vi "Main.vi"() -> ()   [LabVIEW 2015]
uses:
  CustomControl/Model.ctl
  CustomControl/Main Cluster.ctl
  CustomControl/TestParameter.ctl
  CustomControl/MLFB Info.ctl
  CustomControl/Report Info.ctl
  CustomControl/ReportTitle.ctl
  CustomControl/addrPower.ctl
  <vilib>/addons/database/Connection.llb/Conn ObjectReference.ctl
  CustomControl/Lang_Control.ctl
  CustomControl/Autority.ctl
  CustomControl/Keithly Action.ctl
  CustomControl/JustCode.ctl
  CustomControl/Process.ctl
  CustomControl/UserRight.ctl
  <vilib>/addons/database/NI_Database_API.lvlib
panel:
  in  "DisableCurtain":bool caption="关闭安全光幕"
  out "EnablePLC":i32
  out "Register":i32[](array[numeric])
  out "Current":dbl
  out "PLC":refnum<visa-resource-name>
  in  "LCOneT":bool
  out "LightCurtain":bool
  out "No Current":bool
  out "Abort":bool
  in  "Voltage Reset":bool caption="Reset"
  out "voltage":dbl[](array[numeric])
  out "34461":refnum<visa-resource-name>
  in  "Keithly":T1=enum."Null"
  out "IOLightCurtain":bool
  out "Run?":bool=TRUE
  in  "Output":refnum<k21>="Output"
  in  "Input":refnum<k21>="Input"
  out "Operator":string caption="员工"
  in  "Lang":T2
  in  "MainCluster":T3={"parameter"={"Instr"={"34461"="GPIB0::16::INSTR", "PLC"="221", "pwr485"="COM3"}, "pwrSwitch"="Power", "voltage"=[], "mesCurrent"=0.0, "testCurrent"=0.0, "baseCurrent"=0.0, "KG20"=[1.0500000000000007, 1.2, 1.3, 1.4], "KG"=0.0, "KTu"=[], "temperature"=[], "MLFB Info"={"MLFB"="", "Frame"="", "curRange"="", "thermoRs"=0.0, "releaseRs"=0.0, "circuitRs"=0.0, "IL_Current"=0.0, "IL_KG"=0.0, "IL_consTIme"=0, "uL_Current"=0.0, "uL_KG"=0.0, "uL_consTIme"=0, "DA"=0.0, "Action_P1"=0, "Action_P2"=0, "Limit_P1"=0, "Limit_P2"=0, "Limit_P3"=0, "Limit_P4"=0, "reTemperature"=0, "iGauge"=0.0, "oGauge"=0.0, "Torque"=""}, "path"={"template (empty)"=path "", "Report path"=path "", "Backup path"=path ""}, "Report"={"Title"={"订单数量"="", "订单号"="", "生产代码"="", "日期"="", "开始时间"="", "结束时间"="", "测试数量"="", "预载荷时间"=0, "载荷时间"=0, "检验员"="", "MLFB"="", "电流范围"="", "起动时间"="", "快速时间范围"=""}, "uL"={"KTU"=[], "Testing temp"=[], "consTime"=0, "KG"=0.0, "Tripped Time"=[], "test?"=FALSE, "KGR"=[]}, "IL"={"KTU"=[], "Testing temp"=[], "consTime"=0, "KG"=0.0, "Tripped Time"=[], "test?"=FALSE, "KGR"=[]}, "Voltage"=[], "preLoad"=0, "Load"=0, "Total"=0, "JustCode"=[]}, "IO"={"Break"="Tripped", "Out"="Output", "Input"="Input", "Contactor"="Tripped"}, "recordVoltageTime"=60, "buffer"={"temp"=0.0, "PowerSwitch"=[]}, "UL?"=FALSE, "numTrip"=[0, 0, 0, 0], "unIndex"=[], "Message"="", "addrPower"=enum."5A power", "errPower"=FALSE, "Tripped Time"=[], "KGR"=[], "consTime"=0, "Authority"=0, "MLFB"=refnum, "uninstallNum"=0, "trip"=[]}, "File Path"={"reportPath"=path "", "limitTemplate"=path "", "actionTemplate"=path "", "initialPath"=path "", "backupPath"=path ""}, "Period"=0, "Elapse"=0, "Start"=FALSE, "Clear"=FALSE, "Test Count"=0, "TrippedCount"=0, "DelayByUser"=0.0, "DelayInCase"=0.0, "CheckVoltage"=FALSE, "UpLimitVol"=0.0, "DownLimitVol"=0.0}
  in  "exit":bool
  in  "Set":bool
  in  "Edit":bool
  in  "New":bool
  in  "btnAbort":bool
  in  "Start":bool
  in  "Logout":bool caption="3RV极限电流测试系统"
  out "action2CurFactor":dbl caption="动作特性2"
  out "Tab":T10(tab)
  in  "Login":bool caption="登录"
  in  "Password":string caption="密码:"
  in  "UserID":string caption="员工号:"
  out "ShowTripTime":T11
  out "Total":string
  out "remaing":string caption="P1"
  out "EndTime":string caption="测试结束"
  out "StartTime":string caption="测试开始"
  out "totalHour":string
  out "totalSec":string caption="最长测试时间"
  out "trippedStatus":T12={"1"=TRUE, "2"=TRUE, "3"=TRUE, "4"=TRUE, "5"=TRUE, "6"=TRUE, "7"=TRUE, "8"=TRUE, "9"=TRUE, "10"=TRUE, "11"=TRUE, "12"=TRUE, "13"=TRUE, "14"=TRUE, "15"=TRUE, "16"=TRUE, "17"=TRUE, "18"=TRUE, "19"=TRUE, "20"=TRUE}
  in  "Report":bool caption="Generator Report"
  out "orderNum_M":string caption="订单号"
  out "MLFB_show":string caption="MLFB"
  out "process":string caption="测试类型"
  out "current":dbl caption="当前测试电流" format="%#.2g"
  in  "parameter":i32[](listbox)
  out "RunInfo":string caption="运行信息"
  out "Pass":bool caption="通过"
  out "Fail":bool caption="失败"
  out "pirntProcess":u8(slide) scale=0.0..10.0
  in  "ThermalTmFrame":string caption="快速时间范围"
  in  "AccelerationTime":string caption="起动时间"
  out "action2preload":i32 caption="动作特性2"
  out "Factor_Action2":string="7.2"
  out "action2":i32 caption="动作特性2"
  in  "orderNum_P":string caption="订单号"
  out "testCount":string caption="测试数量"
  in  "productCode":string caption="生产代码"
  in  "orderCount":string caption="订单数量"
  in  "TestModel":T13
  in  "Cancel_Para":bool caption="Test"
  in  "ok_Para":bool
  out "load_Limit":i32 caption="载荷"
  out "preload_Limit":i32 caption="预载荷"
  out "Test Date":string caption="测试日期"
  out "Frame":string caption="框架"
  out "Reference temp":i32=20 caption="基准温度"
  out "load_Action":i32 caption="动作特性 1"
  out "preload_Action":i32 caption="极限电流"
  out "Gauge_Out":dbl caption="出现线径"
  out "Gauge_In":dbl caption="进线线径"
  out "Factor_Limit":string="1.05->1.2->1.3->1.4" caption="电流系数"
  out "Factor_Action":string="1.05->1.2" caption="动作特性 2"
  out "Torque":string caption="扭矩"
  out "DA_uL":dbl
  out "DA_IL":dbl caption="期望值"
  out "KG20_uL":dbl
  out "KG20_IL":dbl caption="温度系数"
  out "consTime_uL":i32
  out "consTime_IL":i32 caption="时间常数"
  out "Current_uL":dbl
  out "Current_IL":dbl caption="测试电流"
  out "Operator_test":string caption="操作员"
  in  "MLFB":string
  out "Temperature":string caption="温度"
  in  "Just Code":T14
  in  "Cancel Add":bool
  in  "Add MLFB":bool caption="Add"
  in  "curRange N":string caption="电流范围"
  out "Factor_Limit N":string="1.05->1.2->1.3->1.4" caption="电流系数"
  in  "Preload_Limit N":i32 caption="预载荷"
  in  "Load_Limit N":i32 caption="载荷"
  in  "Resistance N":dbl caption="内阻"
  out "Factor_Action N":string="1.05->1.2"
  in  "Frame N":string caption="框架"
  in  "Current_IL N":dbl caption="电流范围"
  in  "Current_uL N":dbl
  in  "consTime_IL N":i32 caption="时间常数"
  in  "consTime_uL N":i32
  in  "KG20_IL N":dbl caption="温度系数"
  in  "KG20_uL N":dbl
  in  "DA N":dbl caption="期望值"
  in  "Torque N":string caption="扭矩"
  in  "Gauge_In N":dbl caption="进线线径"
  in  "Gauge_Out N":dbl caption="出线线径"
  in  "Preload_Release N":i32 caption="极限电流"
  in  "Load_Release N":i32 caption="动作特性"
  in  "reTemperature N":i32=20 caption="基准温度"
  in  "thermoRs":dbl caption="热元件电阻值"
  in  "releaseRs":dbl caption="电流脱扣器电阻值"
  in  "MLFB N":string caption="MLFB"
  in  "btnDelete":bool caption="删除"
  in  "Cancel_Edit":bool caption="Cancel"
  in  "Ok_Edit":bool caption="Edit"
  in  "Load_Limit E":i32 caption="载荷"
  in  "Preload_Limit E":i32 caption="预载荷"
  out "FactorLimit E":string="1.05->1.2->1.3->1.4" caption="电流系数"
  in  "reTemperature E":i32=20 caption="基准温度"
  in  "Load_Action E":i32 caption="动作特性"
  in  "Preload_Action E":i32 caption="极限电流"
  in  "Gauge_Out E":dbl caption="出线线径"
  in  "Gauge_In E":dbl caption="进线线径"
  in  "Torque E":string caption="扭矩"
  in  "DA E":dbl caption="期望值"
  in  "KG_uL E":dbl
  in  "KG_IL E":dbl caption="温度系数"
  in  "consTime_uL E":i32
  in  "consTime_IL E":i32 caption="时间常数"
  in  "Current_uL E":dbl
  in  "Current_IL E":dbl caption="电流范围"
  in  "MLFB E":string caption="MLFB"
  in  "Frame E":string caption="框架"
  out "FactorRelease E":string="1.05->1.2"
  in  "circuitRs E":dbl caption="内阻"
  in  "curRange E":string caption="电流范围"
  in  "releaseRs E":dbl caption="电流脱扣器电阻值"
  in  "thermoRs E":dbl caption="热元件电阻值"
  in  "btnEditLCConfig":bool caption="New"
  in  "btnReadLCConfig":bool caption="安全光幕"
  out "vlCalTpr":dbl caption="实测温度"
  in  "btnCalTpr":bool caption="温度校验"
  in  "btnReadUser":bool caption="New"
  in  "readCalibra":bool caption="Read"
  out "valueCalibra":dbl caption="测试值"
  in  "Authority":T15 caption="权限"
  in  "btnDeleteUser":bool
  in  "btnEditUser":bool
  in  "btnNewUser":bool caption="用户权限"
  in  "txtPassword":string caption="密码"
  in  "txtName":string caption="姓名"
  in  "txtID":string caption="用户ID"
  in  "setCalibra":dbl caption="设定值"
  in  "btnCalibration":bool caption="电流校验"
  in  "abortCalibra":bool caption="Abort"
  in  "btnReturn":bool caption="Return"
  in  "DelayByUser":string caption="自恢复时间"
  in  "DelayToFailed":string caption="误触发极限"
  # "3RV Limit Current"
  # "sec."
  # "sec."
  # "sec."
  # "A"
  # "h/min/sec"
  # "Test"
  # "Sec"
  # "Sec"
  # "I.L"
  # "u.L"
  # "A"
  # "N.m"
  # "mm2"
  # "mm2"
  # "℃"
  # "℃"
  # "Add"
  # "mΩ"
  # "sec"
  # "sec"
  # "mΩ"
  # "mΩ"
  # "A"
  # "I.L"
  # "u.L"
  # "mm2"
  # "A"
  # "℃"
  # "mm2"
  # "N.m"
  # "Edit"
  # "mΩ"
  # "sec"
  # "sec"
  # "mΩ"
  # "mΩ"
  # "I.L"
  # "u.L"
  # "A"
  # "mm2"
  # "A"
  # "℃"
  # "mm2"
  # "N.m"
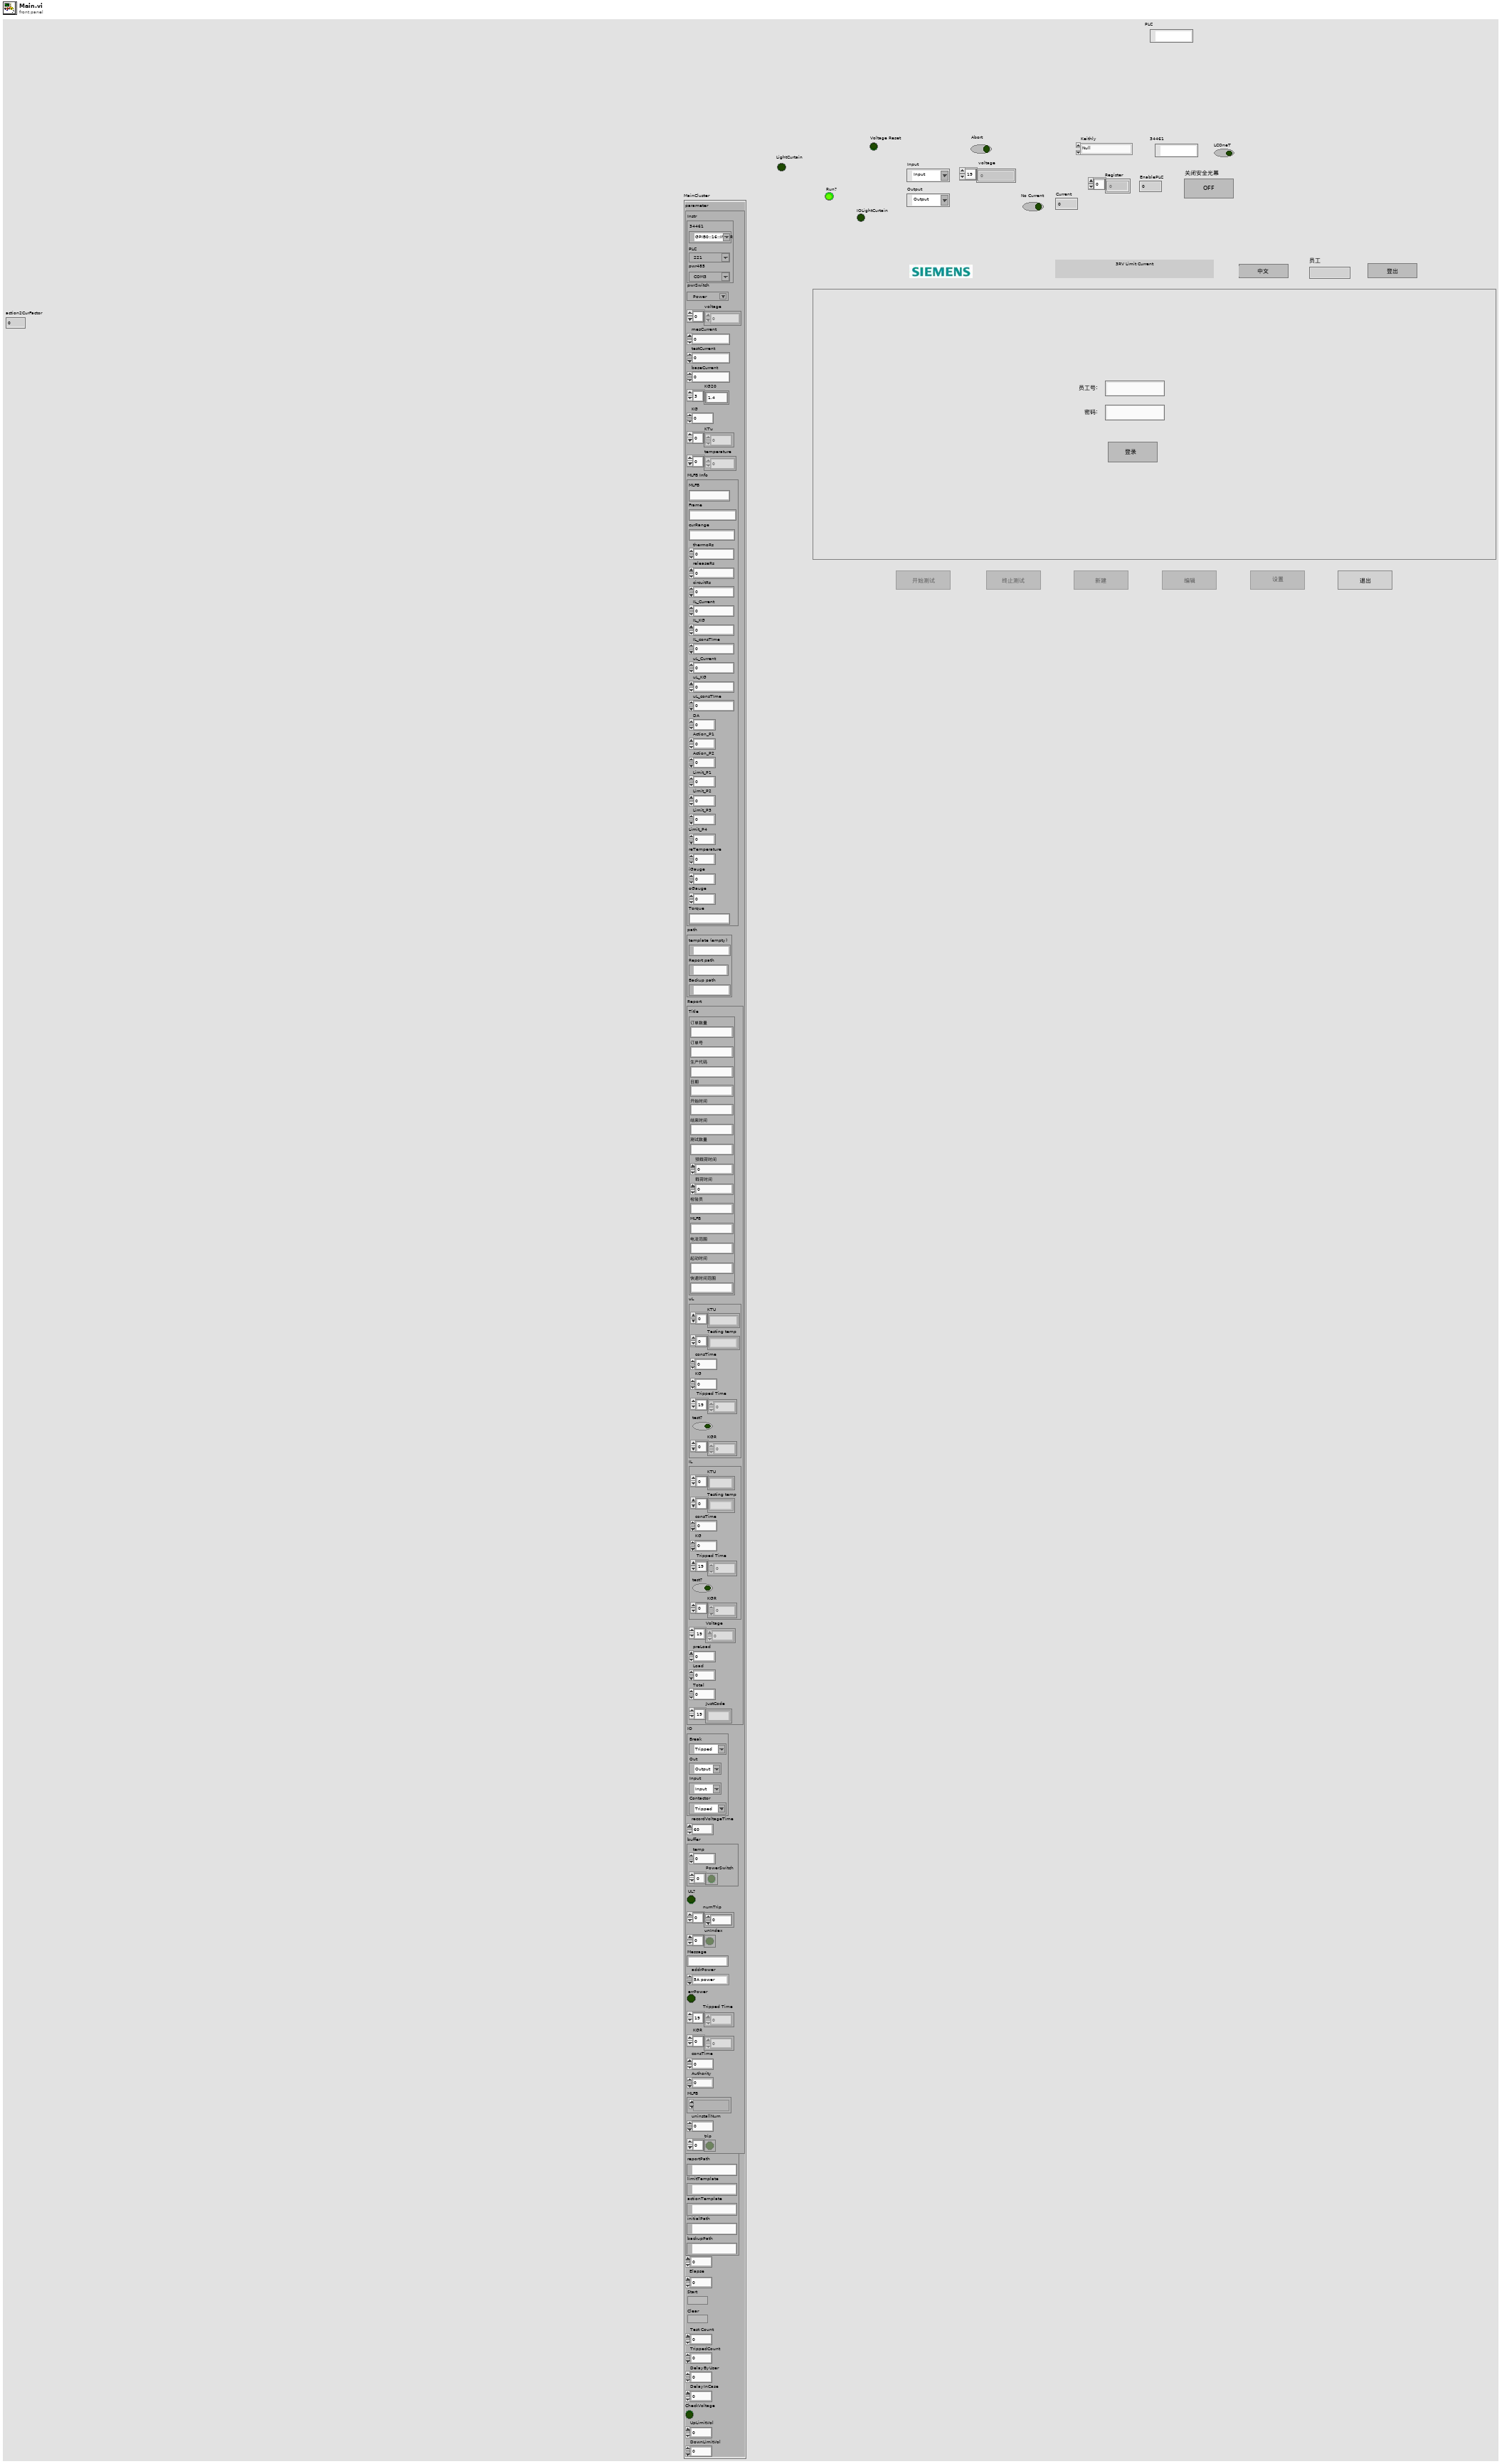
[diagram p1: front panel]
types:
  T1 = typedef "Keithly Action.ctl" = enum16{"Get Voltage", "Null"}
  T2 = typedef "Lang_Control.ctl" = enum16{"中文", "English"}
  T3 = typedef "Main Cluster.ctl" = cluster{"parameter":T4, "File Path":cluster{"reportPath":path, "limitTemplate":path, "actionTemplate":path, "initialPath":path, "backupPath":path}, "Period":u8, "Elapse":i32, "Start":bool, "Clear":bool, "Test Count":u8, "TrippedCount":i32, "DelayByUser":dbl, "DelayInCase":dbl, "CheckVoltage":bool, "UpLimitVol":dbl, "DownLimitVol":dbl}
  T4 = typedef "TestParameter.ctl" = cluster{"Instr":cluster{"34461":refnum<visa-resource-name>, "PLC":refnum<visa-resource-name>, "pwr485":refnum<visa-resource-name>}, "pwrSwitch":refnum<k21>, "voltage":dbl[], "mesCurrent":dbl, "testCurrent":dbl, "baseCurrent":dbl, "KG20":dbl[], "KG":dbl, "KTu":dbl[], "temperature":dbl[], "MLFB Info":T5, "path":cluster{"template (empty)":path, "Report path":path, "Backup path":path}, "Report":T6, "IO":cluster{"Break":refnum<k21>, "Out":refnum<k21>, "Input":refnum<k21>, "Contactor":refnum<k21>}, "recordVoltageTime":i32, "buffer":cluster{"temp":dbl, "PowerSwitch":bool[]}, "UL?":bool, "numTrip":i32[], "unIndex":bool[], "Message":string, "addrPower":T8, "errPower":bool, "Tripped Time":i32[], "KGR":dbl[], "consTime":i32, "Authority":u32, "MLFB":T9, "uninstallNum":i32, "trip":bool[]}
  T5 = typedef "MLFB Info.ctl" = cluster{"MLFB":string, "Frame":string, "curRange":string, "thermoRs":dbl, "releaseRs":dbl, "circuitRs":dbl, "IL_Current":dbl, "IL_KG":dbl, "IL_consTIme":i32, "uL_Current":dbl, "uL_KG":dbl, "uL_consTIme":i32, "DA":dbl, "Action_P1":i32, "Action_P2":i32, "Limit_P1":i32, "Limit_P2":i32, "Limit_P3":i32, "Limit_P4":i32, "reTemperature":i32, "iGauge":dbl, "oGauge":dbl, "Torque":string}
  T6 = typedef "Report Info.ctl" = cluster{"Title":T7, "uL":cluster{"KTU":string[], "Testing temp":string[], "consTime":i32, "KG":dbl, "Tripped Time":i32[], "test?":bool, "KGR":dbl[]}, "IL":cluster{"KTU":string[], "Testing temp":string[], "consTime":i32, "KG":dbl, "Tripped Time":i32[], "test?":bool, "KGR":dbl[]}, "Voltage":dbl[], "preLoad":i32, "Load":i32, "Total":i32, "JustCode":string[]}
  T7 = typedef "ReportTitle.ctl" = cluster{"订单数量":string, "订单号":string, "生产代码":string, "日期":string, "开始时间":string, "结束时间":string, "测试数量":string, "预载荷时间":i32, "载荷时间":i32, "检验员":string, "MLFB":string, "电流范围":string, "起动时间":string, "快速时间范围":string}
  T8 = typedef "addrPower.ctl" = enum16{"5A power", "300A power"}
  T9 = typedef "NI_Database_API.lvlib/Conn ObjectReference.ctl" = refnum<k1>
  T10 = enum32{"Login", "Test", "Parameter", "Add MLFB", "Edit MLFB", "Calibration Power"}
  T11 = cluster{"1":i32, "2":i32, "3":i32, "4":i32, "5":i32, "6":i32, "7":i32, "8":i32, "9":i32, "10":i32, "11":i32, "12":i32, "13":i32, "14":i32, "15":i32, "16":i32, "17":i32, "18":i32, "19":i32, "20":i32}
  T12 = cluster{"1":bool, "2":bool, "3":bool, "4":bool, "5":bool, "6":bool, "7":bool, "8":bool, "9":bool, "10":bool, "11":bool, "12":bool, "13":bool, "14":bool, "15":bool, "16":bool, "17":bool, "18":bool, "19":bool, "20":bool}
  T13 = typedef "Model.ctl" = enum32{"lowLimit", "upLimit", "lowAction1", "upAction1", "lowAction2", "upAction2"}
  T14 = typedef "JustCode.ctl" = cluster{"1":string, "2":string, "3":string, "4":string, "5":string, "6":string, "7":string, "8":string, "9":string, "10":string, "11":string, "12":string, "13":string, "14":string, "15":string, "16":string, "17":string, "18":string, "19":string, "20":string}
  T15 = typedef "Autority.ctl" = enum16{"Operator", "Engineer"}
  T16 = typedef "Process.ctl" = enum16{"Initial_Data", "Initial_HMI", "Language", "UI", "Login", "Authority", "Clear", "Initial Test Data", "Initial Test Data1", "Initial Test UI", "Test Parameter", "PowerRemote", "PowerON", "PowerCalibration", "PowerOFF", "Temperature", "TempOffset", "Trip", "ShowInfo", "Finish?", "Period?", "LoopCurrent", "Procedure", "KGR", "Passed", "Failed", "MLFB Decoding", "MLFB Test Info", "MLFB Edit Info", "MLFB Edit", "MLFB Insert", "MLFB Delete", "ReportGeneralInfo", "ReportResultInfo", "ReportPath", "Generate Report", "Print Report", "New User", "Edit User", "Delete User", "Read User", "Voltage", "Time", "Current Calibration", "ErrorHandle", "StartTest", "ActiveLightCur", "Uninstall Record", "Get Uninstall Count", "Abort Test", "Test Model?", "CheckLoopCurrent", "Release HW Source", "Exit", "Close DB Connection", "Test UI BTN Status", "unTest UI BTN Status", "Disable All BTN", "AbortCalibration", "TprCalibration", "ClearReportInfo", "Set Uninstall", "TestResult", "SetLightCur", "CheckVoltage", "ShowTripTime"}
  T17 = enum16{"HighVoltage", "LowVoltage", "Temperature", "AllOFF"}
  T18 = enum8{"Enabled", "Disabled", "Disabled and Grayed Out"}
  T19 = enum16{"HighVoltage", "LowVoltage", "Temperature"}
  T20 = typedef "UserRight.ctl" = cluster{"ID_Number":string, "Name":string, "Password":string, "Authority":i32}
  T21 = enum32{"invalid app kind", "Development System", "Run Time System", "Student Edition", "Embedded LabVIEW", "Evaluation", "Custom"}
  T22 = cluster{"[0]":bool, "[1]":bool, "[2]":bool, "[3]":bool, "[4]":bool, "[5]":bool, "[6]":bool, "[7]":bool, "[8]":bool, "[9]":bool, "[10]":bool, "[11]":bool, "[12]":bool, "[13]":bool, "[14]":bool, "[15]":bool, "[16]":bool, "[17]":bool, "[18]":bool, "[19]":bool}
  T23 = cluster{"[0]":i32, "[1]":i32, "[2]":i32, "[3]":i32, "[4]":i32, "[5]":i32, "[6]":i32, "[7]":i32, "[8]":i32, "[9]":i32, "[10]":i32, "[11]":i32, "[12]":i32, "[13]":i32, "[14]":i32, "[15]":i32, "[16]":i32, "[17]":i32, "[18]":i32, "[19]":i32}
  T24 = cluster{"trip[0]":bool, "trip[1]":bool, "trip[2]":bool, "trip[3]":bool, "trip[4]":bool, "trip[5]":bool, "trip[6]":bool, "trip[7]":bool, "trip[8]":bool, "trip[9]":bool, "trip[10]":bool, "trip[11]":bool, "trip[12]":bool, "trip[13]":bool, "trip[14]":bool, "trip[15]":bool, "trip[16]":bool, "trip[17]":bool, "trip[18]":bool, "trip[19]":bool}
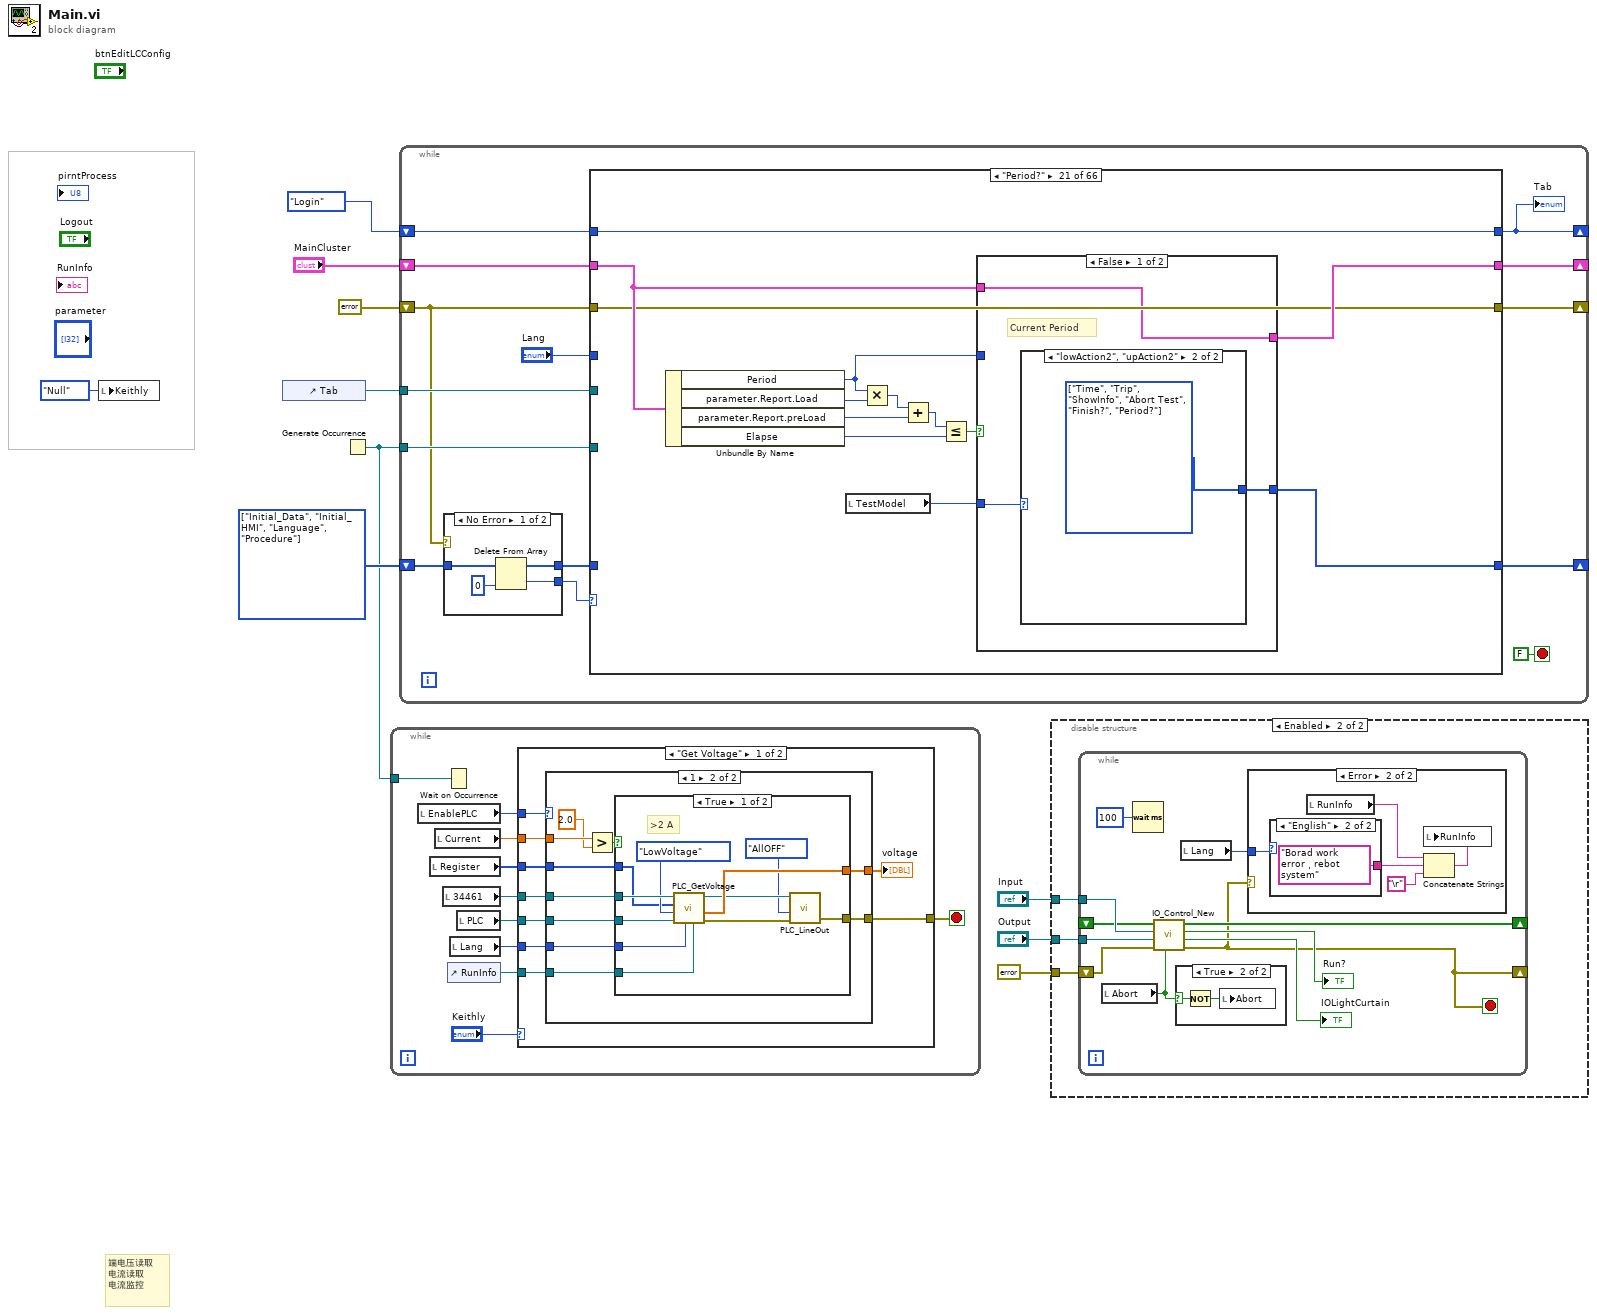
[diagram p0: block diagram]
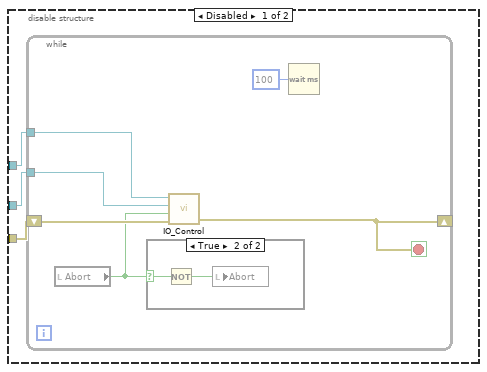
[diagram p2: hidden frame]
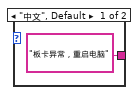
[diagram p5: hidden frame]
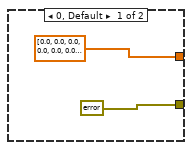
[diagram p7: hidden frame]
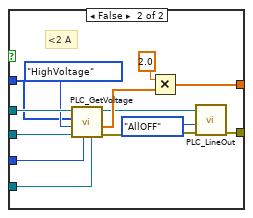
[diagram p8: hidden frame]
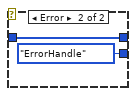
[diagram p10: hidden frame]
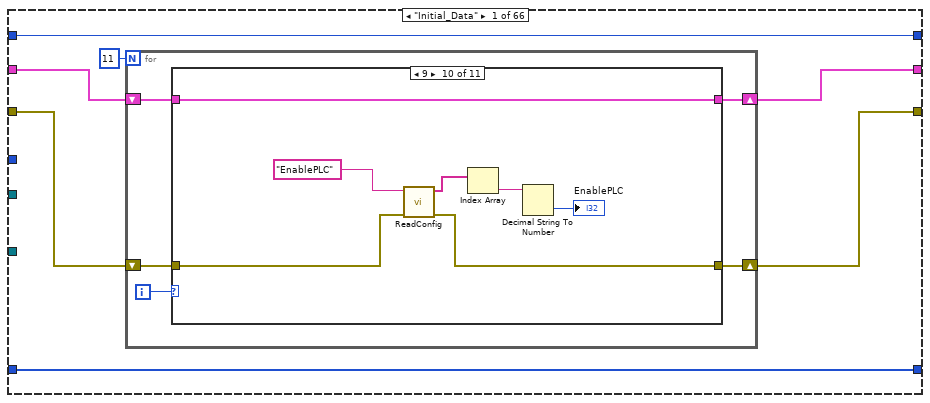
[diagram p11: hidden frame]
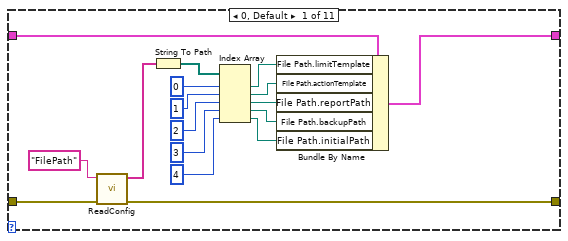
[diagram p12: hidden frame]
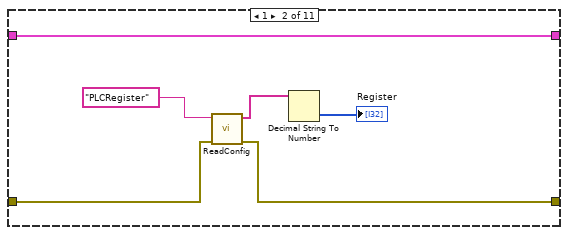
[diagram p13: hidden frame]
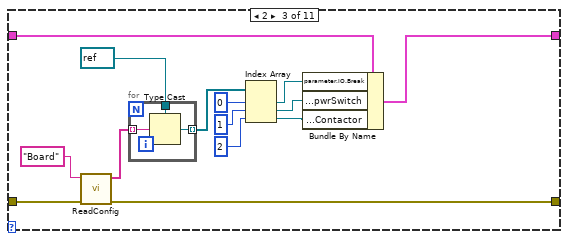
[diagram p14: hidden frame]
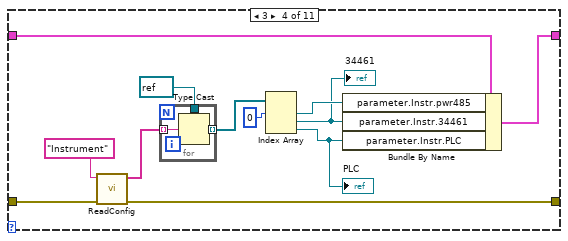
[diagram p15: hidden frame]
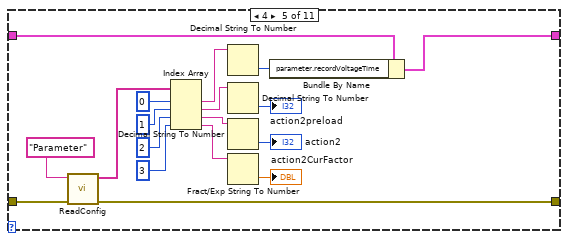
[diagram p16: hidden frame]
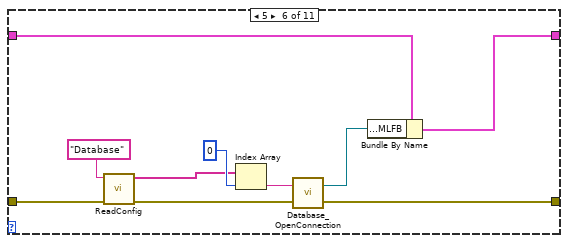
[diagram p17: hidden frame]
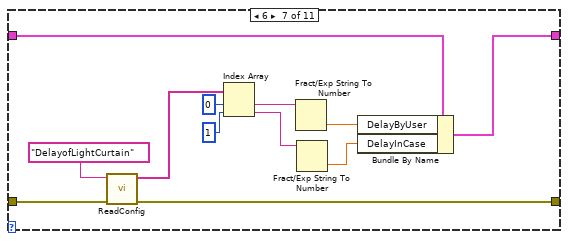
[diagram p18: hidden frame]
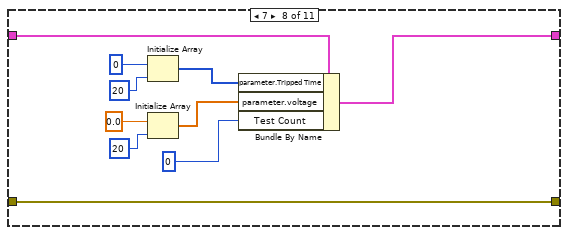
[diagram p19: hidden frame]
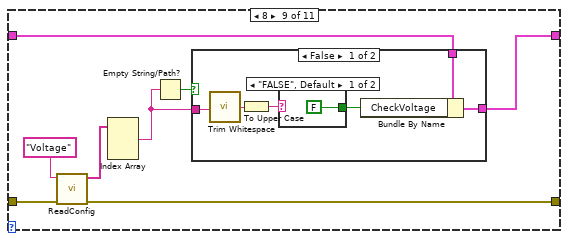
[diagram p20: hidden frame]
diagram:
  w7 = T16[] [enum."Initial_Data", enum."Initial_HMI", enum."Language", enum."Procedure"] items=["Initial_Data", "Initial_HMI", "Language", "UI", "Login", "Authority", "Clear", "Initial Test Data", "Initial Test Data1", "Initial Test UI", "Test Parameter", "PowerRemote", "PowerON", "PowerCalibration", "PowerOFF", "Temperature", "TempOffset", "Trip", "ShowInfo", "Finish?", "Period?", "LoopCurrent", "Procedure", "KGR", "Passed", "Failed", "MLFB Decoding", "MLFB Test Info", "MLFB Edit Info", "MLFB Edit", "MLFB Insert", "MLFB Delete", "ReportGeneralInfo", "ReportResultInfo", "ReportPath", "Generate Report", "Print Report", "New User", "Edit User", "Delete User", "Read User", "Voltage", "Time", "Current Calibration", "ErrorHandle", "StartTest", "ActiveLightCur", "Uninstall Record", "Get Uninstall Count", "Abort Test", "Test Model?", "CheckLoopCurrent", "Release HW Source", "Exit", "Close DB Connection", "Test UI BTN Status", "unTest UI BTN Status", "Disable All BTN", "AbortCalibration", "TprCalibration", "ClearReportInfo", "Set Uninstall", "TestResult", "SetLightCur", "CheckVoltage", "ShowTripTime"]
  # "端电压读取\n电流读取\n电流监控"
  n1 = local write "Keithly"(Keithly_Action."Null" ("Keithly")) -> ()
  n2 = control-ref of="Tab"() -> (w9:refnum<vi>)
  n3 = Generate Occurrence() -> (w5:refnum<k4>)
  n4 = while {
    tunnel: w5 -> [w20]
    stop <- w19 stop-if-true
    n5 = local read "EnablePLC"() -> (w14:i32)
    n6 = local read "Register"() -> (w13:i32[])
    n7 = local read "Current"() -> (w15:dbl)
    n8 = local read "34461"() -> (w18:refnum<visa-resource-name>)
    n9 = Wait on Occurrence(2:w20) -> ()  [unwired: 2 in, 1 out]
    n10 = control-ref of="RunInfo"() -> (w12:refnum<vi>)
    n11 = local read "Lang"() -> (w11:T2)
    n12 = local read "PLC"() -> (w16:refnum<visa-resource-name>)
    n13 = case shown="\"Get Voltage\"" "Keithly" {
      tunnel: [w28 _] -> w19
      tunnel: w18 -> [w29 _]
      tunnel: w16 -> [w26 _]
      tunnel: w15 -> [w25 _]
      tunnel: w14 -> [w24 _]
      tunnel: w13 -> [w23 _]
      tunnel: w12 -> [w22 _]
      tunnel: w11 -> [w21 _]
      frame "Get Voltage" {
        n14 = case shown="1" w24 {
          tunnel: w29 -> [_ w41]
          tunnel: [errorcluster {"status"=FALSE, "code"=0, "source"=""} ("error out") w35] -> w28
          tunnel: [dbl[] [0.0, 0.0, 0.0, 0.0, 0.0, 0.0, 0.0, 0.0, 0.0, 0.0, 0.0, 0.0, 0.0, 0.0, 0.0, 0.0, 0.0, 0.0, 0.0, 0.0] ("Array") w40] -> w27
          tunnel: w26 -> [_ w39]
          tunnel: w25 -> [_ w38]
          tunnel: w23 -> [_ w34]
          tunnel: w22 -> [_ w33]
          tunnel: w21 -> [_ w32]
          frame 0, Default {
          }
          frame 1 {
            n15 = Greater?(x=w38, y=2.0) -> (0:w37:bool)
            n16 = case shown="True" w37 {
              tunnel: w41 -> [w52 w65]
              tunnel: [w47 w59] -> w35
              tunnel: [w48 w62] -> w40
              tunnel: w39 -> [w50 w63]
              tunnel: w34 -> [w44 w55]
              tunnel: w33 -> [w42 w54]
              tunnel: w32 -> [w43 w53]
              frame True {
                # ">2 A"
                n17 = call "PLC_GetVoltage.vi"("Msg"=w42, "Language"=w43, "PLC"=w50, "Selection"=T17."LowVoltage", "VoltageIO"=w44, "VISA"=w52) -> ("error out"=w51:errorcluster, "Array"=w48:dbl[], "VISA resource name out"=w46:refnum<visa-resource-name>)  [unwired: 3 in]
                n18 = call "PLC_LineOut.vi"("error in (no error)"=w51, "Selection"=T17."AllOFF", "VISA resource name"=w46) -> ("error out"=w47:errorcluster)  [unwired: 2 in, 1 out]
              }
              frame False {
                # "<2 A"
                n19 = call "PLC_GetVoltage.vi"("Msg"=w54, "Language"=w53, "PLC"=w63, "Selection"=T17."HighVoltage", "VoltageIO"=w55, "VISA"=w65) -> ("error out"=w64:errorcluster, "Array"=w58:dbl[], "VISA resource name out"=w57:refnum<visa-resource-name>)  [unwired: 3 in]
                n20 = Multiply(x=2.0, y=w58) -> (x*y=w62:dbl[])
                n21 = call "PLC_LineOut.vi"("error in (no error)"=w64, "Selection"=T17."AllOFF", "VISA resource name"=w57) -> ("error out"=w59:errorcluster)  [unwired: 2 in, 1 out]
              }
            }
          }
        }
        "voltage" <- w27
      }
      frame "Null" {
      }
    }
  }
  n22 = while {
    shift-right: [w76] -> _
    shift-left: "MainCluster" -> [w78]
    shift-right: [w70] -> _
    shift-left: T10."Login" ("Tab") -> [w79]
    shift-right: [w77] -> _
    shift-left: errorcluster {"status"=FALSE, "code"=0, "source"=""} ("error out") -> [w67]
    tunnel: w9 -> [w75]
    shift-right: [w72] -> _
    shift-left: w7 -> [w74]
    tunnel: w5 -> [w68]
    stop <- FALSE stop-if-true
    n23 = case shown="No Error" w67 {
      tunnel: w74 -> [w83 w85]
      tunnel: [w80 w85] -> w73
      tunnel: [w81 Process."ErrorHandle" ("Process")] -> w66
      frame No Error {
        n24 = Delete From Array(array=w83, index=0) -> (deleted portion=w81:T16, array with subset deleted=w80:T16[])  [unwired: 1 in]
      }
      frame Error {
      }
    }
    n25 = case shown="\"Period?\"" w66 {
      tunnel: w79 -> [w92 w237 w279 w557 w745 w794 w803 w851 w856 w877 w891 w1030 w1044 w1057 w1069 w1079 w1096 w1126 w1133 w1166 w1192 w1217 w1221 w1233 w1239 w1262 w1290 w1312 w1340 w1373 w1416 w1456 w1479 w1493 w1525 w1535 w1564 w1578 w1608 w1625 w1655 w1666 w1683 w1687 w1693 w1709 w1730 w1743 w1770 w1779 w1799 w1828 w1837 w1844 w1855 w1861 w1867 w1872 w1879 w1891 w1897 w1905 w1912 w1951 w1983 w2015]
      tunnel: w78 -> [w91 w235 w280 w556 w749 w792 w802 w848 w853 w874 w888 w1026 w1039 w1054 w1064 w1076 w1105 w1117 w1131 w1153 w1182 w1213 w1220 w1224 w1236 w1259 w1288 w1309 w1337 w1372 w1415 w1452 w1475 w1480 w1509 w1533 w1563 w1577 w1607 w1623 w1654 w1660 w1678 w1688 w1695 w1713 w1729 w1736 w1767 w1778 w1794 w1827 w1836 w1845 w1851 w1860 w1866 w1871 w1878 w1888 w1893 w1902 w1910 w1948 w1980 w2012]
      tunnel: w67 -> [w90 w236 w281 w555 w753 w793 w801 w849 w855 w876 w889 w1029 w1045 w1055 w1068 w1072 w1099 w1129 w1132 w1152 w1181 w1215 w1218 w1231 w1238 w1261 w1286 w1310 w1338 w1363 w1414 w1455 w1478 w1494 w1524 w1534 w1561 w1565 w1603 w1624 w1642 w1665 w1682 w1686 w1702 w1712 w1728 w1742 w1768 w1777 w1798 w1826 w1835 w1846 w1853 w1859 w1865 w1870 w1876 w1884 w1895 w1904 w1911 w1945 w1978 w2014]
      tunnel: [w89 w236 w281 w554 w743 w793 w801 w849 w855 w876 w889 w1027 w1041 w1047 w1065 w1073 w1099 w1109 w1132 w1152 w1181 w1214 w1218 w1230 w1238 w1261 w1277 w1310 w1338 w1371 w1413 w1454 w1478 w1494 w1513 w1532 w1557 w1575 w1596 w1613 w1640 w1665 w1681 w1686 errorcluster {"status"=FALSE, "code"=0, "source"=""} ("error IO") w1712 w1727 w1742 w1757 w1777 w1798 w1826 w1834 w1846 w1852 w1859 w1865 w1870 w1873 w1889 w1895 w1903 w1911 w1945 w1977 w2014] -> w77
      tunnel: [w88 w235 w280 w553 w744 w792 w802 w836 w852 w874 w890 w1026 w1038 w1054 w1064 w1075 w1104 w1120 w1131 w1153 w1186 w1213 w1220 w1223 w1235 w1259 w1287 w1309 w1337 w1372 w1415 w1452 w1476 w1481 w1519 w1531 w1563 w1577 w1607 w1623 w1654 w1660 w1679 w1688 w1695 w1713 w1729 w1735 w1766 w1778 w1793 w1827 w1836 w1845 w1851 w1860 w1866 w1871 w1878 w1888 w1892 w1902 w1909 w1948 w1980 w2012] -> w76
      tunnel: w75 -> [_ _ _ _ _ _ _ _ _ _ _ _ _ _ _ _ _ _ _ _ _ _ _ _ _ _ _ _ _ _ _ _ _ _ _ _ _ _ _ _ _ _ _ _ _ _ _ _ _ _ _ _ _ _ _ _ _ _ _ _ _ _ _ _ _ _]
      tunnel: [w92 w237 w279 w550 w750 w794 w803 w851 w856 w877 w891 w1030 w1044 w1057 w1069 w1079 w1096 w1126 w1133 w1166 w1192 w1217 w1221 w1233 w1239 w1262 w1290 w1312 w1340 w1373 w1416 w1456 w1479 w1493 w1525 w1535 w1564 w1578 w1608 w1625 w1655 w1666 w1683 w1687 w1690 w1708 w1730 w1743 w1770 w1779 w1799 w1828 w1837 w1844 w1855 w1861 w1867 w1872 w1879 w1891 w1897 w1905 w1912 w1951 w1983 w2015] -> w70
      tunnel: [w86 w234 w278 w549 w741 w790 w799 w850 w854 w875 w885 w1025 w1040 w1056 w1063 w1078 w1095 w1121 w1130 w1158 w1187 w1216 w1219 w1232 w1237 w1260 w1289 w1311 w1339 w1367 w1407 w1457 w1477 w1492 w1518 w1536 w1560 w1574 w1597 w1622 w1645 w1664 w1684 w1685 w1700 w1707 w1731 w1741 w1764 w1776 w1797 w1824 w1838 w1847 w1854 w1858 w1864 w1869 w1877 w1890 w1896 w1899 w1907 w1950 w1982 w2013] -> w72
      tunnel: w73 -> [w86 w234 w278 _ w742 w790 w800 w850 w854 w875 w885 w1025 w1040 w1056 w1063 w1078 w1095 w1121 w1130 w1160 _ w1216 _ w1232 w1237 w1260 w1289 w1311 w1339 w1367 w1407 w1457 w1477 w1492 w1518 w1536 w1560 w1574 w1597 w1622 w1645 w1664 w1684 w1685 _ _ w1731 w1741 w1764 w1776 w1797 w1825 w1838 w1847 w1854 w1858 w1864 w1869 w1877 w1890 w1896 w1899 _ w1950 w1982 w2013]
      tunnel: "Lang" -> [_ w233 w277 w551 w751 _ _ _ _ _ w886 w1022 w1031 w1052 w1058 _ _ _ _ _ _ _ _ _ w1234 w1258 w1278 _ _ w1368 w1410 w1449 _ _ _ _ w1554 w1573 _ w1612 w1644 _ _ _ _ w1710 _ _ _ w1774 _ _ _ _ _ _ _ _ _ _ _ _ _ w1944 _ _]
      tunnel: w68 -> [_ _ _ _ _ _ _ _ _ _ _ _ _ _ _ _ _ _ _ _ _ _ _ _ _ _ _ _ _ _ _ _ _ _ _ _ _ _ _ _ _ w1663 _ _ _ _ _ _ _ _ _ _ _ _ _ _ _ _ _ _ _ _ _ _ _ _]
      frame "Initial_Data" {
        n26 = for {
          N: 11 -> [_]
          shift-right: [w96] -> w89
          shift-left: w90 -> [w97]
          shift-right: [w94] -> w88
          shift-left: w91 -> [w95]
          i -> [w93]
          n27 = case shown="9" w93 {
            tunnel: w97 -> [w113 w119 w134 w144 w170 w180 w191 w202 w210 w227 w232]
            tunnel: [w112 w118 w133 w145 w169 w175 w190 w202 w209 w226 w232] -> w96
            tunnel: w95 -> [w111 w120 w131 w148 w167 w178 w192 w201 w204 w228 w231]
            tunnel: [w98 w120 w123 w139 w156 w171 w181 w193 w203 w228 w230] -> w94
            frame 0, Default {
              n28 = call "ReadConfig.vi"("error in"=w113, "section"="FilePath") -> ("error out"=w112:errorcluster, "value"=w110:string[])  [unwired: 3 in, 1 out]
              n29 = String To Path(string=w110) -> (path=w109:path[])
              n30 = Index Array(array=w109, index #1=0 ("index"), index #2=1 ("index"), index #3=2 ("index"), index #4=3 ("index"), index #5=4 ("index")) -> (element #1=w103:path, element #2=w102:path, element #3=w101:path, element #4=w100:path, element #5=w99:path)
              n31 = Bundle By Name(cluster=w111, "File Path.limitTemplate"=w103, "File Path.actionTemplate"=w102, "File Path.reportPath"=w101, "File Path.backupPath"=w100, "File Path.initialPath"=w99) -> (w98:T3)
            }
            frame 1 {
              n32 = call "ReadConfig.vi"("error in"=w119, "section"="PLCRegister") -> ("error out"=w118:errorcluster, "value"=w116:string[])  [unwired: 3 in, 1 out]
              n33 = Decimal String To Number(string=w116) -> (number=→"Register":i32[])  [unwired: 2 in, 1 out]
            }
            frame 2 {
              n34 = call "ReadConfig.vi"("error in"=w134, "section"="Board") -> ("error out"=w133:errorcluster, "value"=w130:string[])  [unwired: 3 in, 1 out]
              n35 = for {
                tunnel: w130 -> [w137] mode=indexing
                tunnel: refnum<k21> refnum ("parameter.IO.Break") -> [w136]
                tunnel: [w135] -> w121 mode=indexing
                n36 = Type Cast(type=w136, x=w137) -> (*(type *) &x=w135:refnum<k21>)
              }
              n37 = Index Array(array=w121, index #1=0 ("index"), index #2=1 ("index"), index #3=2 ("index")) -> (element #1=w128:refnum<k21>, element #2=w127:refnum<k21>, element #3=w122:refnum<k21>)
              n38 = Bundle By Name(cluster=w131, "parameter.IO.Break"=w128, "parameter.pwrSwitch"=w127, "parameter.IO.Contactor"=w122) -> (w123:T3)
            }
            frame 3 {
              n39 = call "ReadConfig.vi"("error in"=w144, "section"="Instrument") -> ("error out"=w145:errorcluster, "value"=w147:string[])  [unwired: 3 in, 1 out]
              n40 = for {
                tunnel: w147 -> [w152] mode=indexing
                tunnel: refnum<visa-resource-name> refnum ("VISA resource name") -> [w151]
                tunnel: [w150] -> w143 mode=indexing
                n41 = Type Cast(type=w151, x=w152) -> (*(type *) &x=w150:refnum<visa-resource-name>)
              }
              n42 = Index Array(array=w143, index #1=0 ("index")) -> (element #1=w141:refnum<visa-resource-name>, element #2=w140:refnum<visa-resource-name>, element #3=w138:refnum<visa-resource-name>)  [unwired: 2 in]
              "34461" <- w140
              "PLC" <- w138
              n43 = Bundle By Name(cluster=w148, "parameter.Instr.pwr485"=w141, "parameter.Instr.34461"=w140, "parameter.Instr.PLC"=w138) -> (w139:T3)
            }
            frame 4 {
              n44 = call "ReadConfig.vi"("error in"=w170, "section"="Parameter") -> ("error out"=w169:errorcluster, "value"=w153:string[])  [unwired: 3 in, 1 out]
              n45 = Index Array(array=w153, index #1=0 ("index"), index #2=1 ("index"), index #3=2 ("index"), index #4=3 ("index")) -> (element #1=w163:string, element #2=w162:string, element #3=w160:string, element #4=w157:string)
              n46 = Decimal String To Number(string=w163) -> (number=w164:i32)  [unwired: 2 in, 1 out]
              n47 = Decimal String To Number(string=w162) -> (number=→"action2preload":i32)  [unwired: 2 in, 1 out]
              n48 = Decimal String To Number(string=w160) -> (number=→"action2":i32)  [unwired: 2 in, 1 out]
              n49 = Fract/Exp String To Number(string=w157) -> (number=→"action2CurFactor":dbl)  [unwired: 3 in, 1 out]
              n50 = Bundle By Name(cluster=w167, "parameter.recordVoltageTime"=w164) -> (w156:T3)
            }
            frame 5 {
              n51 = call "ReadConfig.vi"("error in"=w180, "section"="Database") -> ("error out"=w176:errorcluster, "value"=w173:string[])  [unwired: 3 in, 1 out]
              n52 = Index Array(array=w173, index=0) -> (element=w172:string)
              n53 = call "Database_OpenConnection.vi"("error in"=w176, "Database"=w172) -> ("error out"=w175:errorcluster, "connection reference"=w174:T9)
              n54 = Bundle By Name(cluster=w178, "parameter.MLFB"=w174) -> (w171:T3)
            }
            frame 6 {
              n55 = call "ReadConfig.vi"("error in"=w191, "section"="DelayofLightCurtain") -> ("error out"=w190:errorcluster, "value"=w188:string[])  [unwired: 3 in, 1 out]
              n56 = Index Array(array=w188, index #1=0 ("index"), index #2=1 ("index")) -> (element #1=w187:string, element #2=w184:string)
              n57 = Fract/Exp String To Number(string=w187) -> (number=w182:dbl)  [unwired: 3 in, 1 out]
              n58 = Fract/Exp String To Number(string=w184) -> (number=w183:dbl)  [unwired: 3 in, 1 out]
              n59 = Bundle By Name(cluster=w192, "DelayByUser"=w182, "DelayInCase"=w183) -> (w181:T3)
            }
            frame 7 {
              n60 = Initialize Array(0, 20) -> (w198:i32[])
              n61 = Initialize Array(0.0, 20) -> (w195:dbl[])
              n62 = Bundle By Name(cluster=w201, "parameter.Tripped Time"=w198, "parameter.voltage"=w195, "Test Count"=u8 0) -> (w193:T3)
            }
            frame 8 {
              n63 = call "ReadConfig.vi"("error in"=w210, "section"="Voltage") -> ("error out"=w209:errorcluster, "value"=w207:string[])  [unwired: 3 in, 1 out]
              n64 = Index Array(array=w207) -> (element #1=w205:string)  [unwired: 3 in, 2 out]
              n65 = Empty String/Path?(string/path=w205) -> (empty?=w206:bool)
              n66 = case shown="False" w206 {
                tunnel: w205 -> [w214 _]
                tunnel: w204 -> [w216 w221]
                tunnel: [w211 w219] -> w203
                frame False {
                  n67 = call <vilib>:"Trim Whitespace.vi"("string"=w214) -> ("trimmed string"=w213:string)  [unwired: 1 in]
                  n68 = To Upper Case(1:w213) -> (0:w215:string)
                  n69 = case shown="\"FALSE\", Default" w215 {
                    tunnel: [FALSE ("CheckVoltage") TRUE ("CheckVoltage")] -> w212
                    frame "FALSE", Default {
                    }
                    frame "TRUE" {
                    }
                  }
                  n70 = Bundle By Name(cluster=w216, "CheckVoltage"=w212) -> (w211:T3)
                }
                frame True {
                  n71 = Bundle By Name(cluster=w221, "CheckVoltage"=FALSE) -> (w219:T3)
                }
              }
            }
            frame 9 {
              n72 = call "ReadConfig.vi"("error in"=w227, "section"="EnablePLC") -> ("error out"=w226:errorcluster, "value"=w224:string[])  [unwired: 3 in, 1 out]
              n73 = Index Array(array=w224) -> (element=w223:string)  [unwired: 1 in]
              n74 = Decimal String To Number(string=w223) -> (number=→"EnablePLC":i32)  [unwired: 2 in, 1 out]
            }
            frame 10 {
              w229 = FALSE ("parameter.Report.uL.test?")
              n75 = Bundle By Name(cluster=w231, "parameter.Report.uL.test?"=w229, "parameter.Report.IL.test?"=w229) -> (w230:T3)
            }
          }
        }
      }
      frame "Initial_HMI" {
        n76 = stacked-sequence {
          tunnel: w233 -> [_ _ _ _ _]
          frame #0 {
            w240 = FALSE ("Fail")
            w245 = T18."Disabled and Grayed Out" ("Disabled")
            w244 = "1.05->1.2->1.3->1.4" ("Factor_Limit")
            w243 = "1.05->1.2" ("Factor_Action")
            n77 = property on="reTemperature N" class="DigNum (strict)"("Value"=20 ("reTemperature N")) -> ()  [unwired: 2 in, 2 out]
            n78 = property on="Temperature" class="Str"("Value"="" ("Temperature")) -> ()  [unwired: 2 in, 2 out]
            n79 = property on="Fail" class="Bool (strict)"("Value"=w240) -> ()  [unwired: 2 in, 2 out]
            n80 = property on="Pass" class="Bool (strict)"("Value"=w240) -> ()  [unwired: 2 in, 2 out]
            n81 = property on="btnAbort" class="Bool (strict)"("DisabledEnum"=w245) -> ()  [unwired: 2 in, 2 out]
            n82 = property on="Report" class="Bool (strict)"("DisabledEnum"=w245) -> ()  [unwired: 2 in, 2 out]
            n83 = property on="trippedStatus" class="Clust (strict)"() -> ("AllObjs[]"=w239:refnum<vi>[])  [unwired: 2 in, 2 out]
            n84 = for {
              tunnel: w239 -> [w249] mode=indexing
              tunnel: cluster{u32, u32}[] [{16711680, 16711680}, {6618880, 6618880}, {13816530, 16744703}, {3381759, 16777088}] ("Array") -> [w247]
              w250 = refnum<vi> refnum  # Boolean
              n85 = To More Specific Class(target class=w250, reference=w249) -> (specific class reference=w248:refnum<vi>)  [unwired: 1 in, 1 out]
              n86 = property class="Bool"(reference=w248, "Colors [4]"=w247) -> ()  [unwired: 1 in, 2 out]
            }
            "Factor_Action" <- w243
            "Factor_Limit" <- w244
            "Factor_Action2" <- "7.2" ("Factor_Action2")
            "Factor_Action N" <- w243
            "Factor_Limit N" <- w244
            "FactorLimit E" <- w244
            "FactorRelease E" <- w243
          }
          frame #1 {
            w252 = 0 ("load_Action")
            w251 = "" ("Operator_test")
            w253 = "" ("EndTime")
            w254 = "" ("Caption.Text")
            n87 = property on="Operator" class="Str"("Value"=w254) -> ()  [unwired: 2 in, 2 out]
            n88 = property on="UserID" class="Str"("Value"=w254) -> ()  [unwired: 2 in, 2 out]
            n89 = property on="Password" class="Str"("Value"=w254) -> ()  [unwired: 2 in, 2 out]
            n90 = property on="orderNum_M" class="Str"("Value"=w254) -> ()  [unwired: 2 in, 2 out]
            n91 = property on="process" class="Str"("Value"=w254) -> ()  [unwired: 2 in, 2 out]
            n92 = property on="StartTime" class="Str"("Value"=w254) -> ()  [unwired: 2 in, 2 out]
            n93 = property on="EndTime" class="Str"("Value"=w253) -> ()  [unwired: 2 in, 2 out]
            n94 = property on="totalSec" class="Str"("Value"=w253) -> ()  [unwired: 2 in, 2 out]
            n95 = property on="RunInfo" class="Str"("Value"=w253) -> ()  [unwired: 2 in, 2 out]
            n96 = property on="orderNum_P" class="Str"("Value"=w253) -> ()  [unwired: 2 in, 2 out]
            n97 = property on="orderCount" class="Str"("Value"=w253) -> ()  [unwired: 2 in, 2 out]
            n98 = property on="testCount" class="Str"("Value"=w253) -> ()  [unwired: 2 in, 2 out]
            n99 = property on="Operator_test" class="Str"("Value"=w251) -> ()  [unwired: 2 in, 2 out]
            n100 = property on="Frame" class="Str"("Value"=w251) -> ()  [unwired: 2 in, 2 out]
            n101 = property on="Test Date" class="Str"("Value"=w251) -> ()  [unwired: 2 in, 2 out]
            n102 = property on="Torque" class="Str"("Value"=w251) -> ()  [unwired: 2 in, 2 out]
            n103 = property on="AccelerationTime" class="Str"("Value"=w251) -> ()  [unwired: 2 in, 2 out]
            n104 = property on="ThermalTmFrame" class="Str"("Value"=w251) -> ()  [unwired: 2 in, 2 out]
            n105 = property on="load_Action" class="DigNum (strict)"("Value"=w252) -> ()  [unwired: 2 in, 2 out]
            n106 = property on="preload_Limit" class="DigNum (strict)"("Value"=w252) -> ()  [unwired: 2 in, 2 out]
            n107 = property on="load_Limit" class="DigNum (strict)"("Value"=w252) -> ()  [unwired: 2 in, 2 out]
            n108 = property on="consTime_IL" class="DigNum (strict)"("Value"=w252) -> ()  [unwired: 2 in, 2 out]
            n109 = property on="preload_Action" class="DigNum (strict)"("Value"=w252) -> ()  [unwired: 2 in, 2 out]
            n110 = property on="Reference temp" class="DigNum (strict)"("Value"=w252) -> ()  [unwired: 2 in, 2 out]
          }
          frame #2 {
            w255 = 0.0 ("current")
            w256 = "" ("Frame E")
            w257 = 0 ("Preload_Release N")
            w258 = 0.0 ("Current_IL N")
            n111 = property on="Current_IL N" class="DigNum (strict)"("Value"=w258) -> ()  [unwired: 2 in, 2 out]
            n112 = property on="Resistance N" class="DigNum (strict)"("Value"=w258) -> ()  [unwired: 2 in, 2 out]
            n113 = property on="thermoRs" class="DigNum (strict)"("Value"=w258) -> ()  [unwired: 2 in, 2 out]
            n114 = property on="releaseRs" class="DigNum (strict)"("Value"=w258) -> ()  [unwired: 2 in, 2 out]
            n115 = property on="Gauge_In N" class="DigNum (strict)"("Value"=w258) -> ()  [unwired: 2 in, 2 out]
            n116 = property on="Gauge_Out N" class="DigNum (strict)"("Value"=w258) -> ()  [unwired: 2 in, 2 out]
            n117 = property on="Preload_Release N" class="DigNum (strict)"("Value"=w257) -> ()  [unwired: 2 in, 2 out]
            n118 = property on="Load_Release N" class="DigNum (strict)"("Value"=w257) -> ()  [unwired: 2 in, 2 out]
            n119 = property on="TestModel" class="RadioBtnsControl (strict)"("Value"=w257) -> ()  [unwired: 2 in, 2 out]
            n120 = property on="Load_Limit N" class="DigNum (strict)"("Value"=w257) -> ()  [unwired: 2 in, 2 out]
            n121 = property on="consTime_IL N" class="DigNum (strict)"("Value"=w257) -> ()  [unwired: 2 in, 2 out]
            n122 = property on="Preload_Limit N" class="DigNum (strict)"("Value"=w257) -> ()  [unwired: 2 in, 2 out]
            n123 = property on="Frame N" class="Str"("Value"=w256) -> ()  [unwired: 2 in, 2 out]
            n124 = property on="curRange N" class="Str"("Value"=w256) -> ()  [unwired: 2 in, 2 out]
            n125 = property on="Torque N" class="Str"("Value"=w256) -> ()  [unwired: 2 in, 2 out]
            n126 = property on="Frame E" class="Str"("Value"=w256) -> ()  [unwired: 2 in, 2 out]
            n127 = property on="curRange E" class="Str"("Value"=w256) -> ()  [unwired: 2 in, 2 out]
            n128 = property on="Torque E" class="Str"("Value"=w256) -> ()  [unwired: 2 in, 2 out]
            n129 = property on="current" class="DigNum (strict)"("Value"=w255) -> ()  [unwired: 2 in, 2 out]
            n130 = property on="DA_IL" class="DigNum (strict)"("Value"=w255) -> ()  [unwired: 2 in, 2 out]
            n131 = property on="Current_IL" class="DigNum (strict)"("Value"=w255) -> ()  [unwired: 2 in, 2 out]
            n132 = property on="Gauge_In" class="DigNum (strict)"("Value"=w255) -> ()  [unwired: 2 in, 2 out]
            n133 = property on="KG20_IL" class="DigNum (strict)"("Value"=w255) -> ()  [unwired: 2 in, 2 out]
            n134 = property on="Gauge_Out" class="DigNum (strict)"("Value"=w255) -> ()  [unwired: 2 in, 2 out]
          }
          frame #3 {
            w259 = 0.0 ("KG20_IL N")
            w260 = "" ("MLFB")
            w262 = "" ("txtID")
            w263 = 0.0 ("DA E")
            w264 = 0 ("Load_Limit E")
            n135 = property on="Load_Limit E" class="DigNum (strict)"("Value"=w264) -> ()  [unwired: 2 in, 2 out]
            n136 = property on="consTime_IL E" class="DigNum (strict)"("Value"=w264) -> ()  [unwired: 2 in, 2 out]
            n137 = property on="Preload_Action E" class="DigNum (strict)"("Value"=w264) -> ()  [unwired: 2 in, 2 out]
            n138 = property on="Load_Action E" class="DigNum (strict)"("Value"=w264) -> ()  [unwired: 2 in, 2 out]
            n139 = property on="Preload_Limit E" class="DigNum (strict)"("Value"=w264) -> ()  [unwired: 2 in, 2 out]
            n140 = property on="reTemperature E" class="DigNum (strict)"("Value"=20 ("reTemperature E")) -> ()  [unwired: 2 in, 2 out]
            n141 = property on="DA E" class="DigNum (strict)"("Value"=w263) -> ()  [unwired: 2 in, 2 out]
            n142 = property on="Current_IL E" class="DigNum (strict)"("Value"=w263) -> ()  [unwired: 2 in, 2 out]
            n143 = property on="KG_IL E" class="DigNum (strict)"("Value"=w263) -> ()  [unwired: 2 in, 2 out]
            n144 = property on="circuitRs E" class="DigNum (strict)"("Value"=w263) -> ()  [unwired: 2 in, 2 out]
            n145 = property on="thermoRs E" class="DigNum (strict)"("Value"=w263) -> ()  [unwired: 2 in, 2 out]
            n146 = property on="releaseRs E" class="DigNum (strict)"("Value"=w263) -> ()  [unwired: 2 in, 2 out]
            n147 = property on="txtID" class="Str"("Value"=w262) -> ()  [unwired: 2 in, 2 out]
            n148 = property on="txtName" class="Str"("Value"=w262) -> ()  [unwired: 2 in, 2 out]
            n149 = property on="txtPassword" class="Str"("Value"=w262) -> ()  [unwired: 2 in, 2 out]
            n150 = property on="MLFB N" class="Str"("Value"=w262) -> ()  [unwired: 2 in, 2 out]
            n151 = property on="MLFB E" class="Str"("Value"=w262) -> ()  [unwired: 2 in, 2 out]
            n152 = property on="MLFB_show" class="Str"("Value"=w262) -> ()  [unwired: 2 in, 2 out]
            n153 = property on="MLFB" class="Str"("Value"=w260) -> ()  [unwired: 2 in, 2 out]
            n154 = local write "totalHour"(w260) -> ()
            n155 = property on="productCode" class="Str"("Value"=w260) -> ()  [unwired: 2 in, 2 out]
            n156 = property on="KG20_IL N" class="DigNum (strict)"("Value"=w259) -> ()  [unwired: 2 in, 2 out]
            n157 = property on="DA N" class="DigNum (strict)"("Value"=w259) -> ()  [unwired: 2 in, 2 out]
          }
          frame #4 {
            w271 = "0" ("remaing")
            w274 = T18."Disabled and Grayed Out" ("Disabled")
            w270 = 0.0 ("valueCalibra")
            n158 = Array To Cluster(array=bool[] [TRUE, TRUE, TRUE, TRUE, TRUE, TRUE, TRUE, TRUE, TRUE, TRUE, TRUE, TRUE, TRUE, TRUE, TRUE, TRUE, TRUE, TRUE, TRUE, TRUE]) -> (cluster=w267:T22)
            n159 = Array To Cluster(array=i32[] [0, 0, 0, 0, 0, 0, 0, 0, 0, 0, 0, 0, 0, 0, 0, 0, 0, 0, 0, 0]) -> (cluster=w265:T23)
            n160 = property on="parameter" class="MCListbox (strict)"("ItemNames"=string[][] [["", "", "", ""], ["", "", "", ""], ["", "", "", ""], ["", "", "", ""]] ("Item Names")) -> ()  [unwired: 2 in, 2 out]
            n161 = property on="remaing" class="Str"("Caption.Text"="P1") -> ()  [unwired: 2 in, 2 out]
            n162 = local write "pirntProcess"(u8 0 ("pirntProcess")) -> ()
            n163 = local write "ShowTripTime"(w265) -> ()
            n164 = local write "trippedStatus"(w267) -> ()
            n165 = property on="Start" class="Bool"("DisabledEnum"=w274) -> ()  [unwired: 2 in, 2 out]
            n166 = property on="New" class="Bool"("DisabledEnum"=w274) -> ()  [unwired: 2 in, 2 out]
            n167 = property on="Edit" class="Bool"("DisabledEnum"=w274) -> ()  [unwired: 2 in, 2 out]
            n168 = property on="Set" class="Bool"("DisabledEnum"=w274) -> ()  [unwired: 2 in, 2 out]
            n169 = local write "DisableCurtain"(FALSE ("DisableCurtain")) -> ()
            n170 = property on="setCalibra" class="DigNum (strict)"("Value"=w270) -> ()  [unwired: 2 in, 2 out]
            n171 = property on="vlCalTpr" class="DigNum (strict)"("Value"=w270) -> ()  [unwired: 2 in, 2 out]
            n172 = property on="Authority" class="Enum (strict)"("Value"=enum16{"Operator", "Engineer"}."Operator") -> ()  [unwired: 2 in, 2 out]
            n173 = property on="remaing" class="Str"("Value"=w271) -> ()  [unwired: 2 in, 2 out]
            n174 = property on="Total" class="Str"("Value"=w271) -> ()  [unwired: 2 in, 2 out]
          }
        }
      }
      frame "Language" {
        n175 = stacked-sequence {
          tunnel: w277 -> [w282 w321 w362 w398 w439 w480 w509]
          frame #0 {
            n176 = case shown="\"中文\", Default" w282 {
              frame "English" {
                n177 = property on="Edit" class="Bool"("BoolText.Text"="Edit" ("Boolean Text.Text")) -> ()  [unwired: 2 in, 2 out]
                n178 = property on="Set" class="Bool"("BoolText.Text"="Set" ("Boolean Text.Text")) -> ()  [unwired: 2 in, 2 out]
                n179 = property on="exit" class="Bool"("BoolText.Text"="Exit" ("Boolean Text.Text")) -> ()  [unwired: 2 in, 2 out]
                n180 = property on="New" class="Bool"("BoolText.Text"="New" ("Boolean Text.Text")) -> ()  [unwired: 2 in, 2 out]
                n181 = property on="Login" class="Bool"("BoolText.Text"="Login" ("Boolean Text.Text")) -> ()  [unwired: 2 in, 2 out]
                n182 = property on="UserID" class="Str"("Caption.Text"="UserID: ") -> ()  [unwired: 2 in, 2 out]
                n183 = property on="Logout" class="Bool"("BoolText.Text"="Logout" ("Boolean Text.Text")) -> ()  [unwired: 2 in, 2 out]
                n184 = property on="Pass" class="Bool (strict)"("Caption.Text"="Passed") -> ()  [unwired: 2 in, 2 out]
                n185 = property on="Fail" class="Bool (strict)"("Caption.Text"="Failed") -> ()  [unwired: 2 in, 2 out]
                n186 = property on="Operator" class="Str"("Caption.Text"="Operator") -> ()  [unwired: 2 in, 2 out]
                n187 = property on="process" class="Str"("Caption.Text"="Test Type") -> ()  [unwired: 2 in, 2 out]
                n188 = property on="StartTime" class="Str"("Caption.Text"="Test Start") -> ()  [unwired: 2 in, 2 out]
                n189 = property on="EndTime" class="Str"("Caption.Text"="Test End") -> ()  [unwired: 2 in, 2 out]
                n190 = property on="RunInfo" class="Str"("Caption.Text"="RunInfo") -> ()  [unwired: 2 in, 2 out]
                n191 = property on="Report" class="Bool (strict)"("BoolText.Text"="Generator" ("Caption.Text")) -> ()  [unwired: 2 in, 2 out]
                n192 = property on="Start" class="Bool"("BoolText.Text"="Start Test" ("Boolean Text.Text")) -> ()  [unwired: 2 in, 2 out]
                n193 = property on="totalSec" class="Str"("Caption.Text"="Maxmium") -> ()  [unwired: 2 in, 2 out]
                n194 = property on="Password" class="Str"("Caption.Text"="Password: ") -> ()  [unwired: 2 in, 2 out]
                n195 = property on="btnAbort" class="Bool (strict)"("BoolText.Text"="Abort Test" ("Boolean Text.Text")) -> ()  [unwired: 2 in, 2 out]
              }
              frame "中文", Default {
                n196 = property on="New" class="Bool"("BoolText.Text"="新建" ("Boolean Text.Text")) -> ()  [unwired: 2 in, 2 out]
                n197 = property on="Edit" class="Bool"("BoolText.Text"="编辑" ("Boolean Text.Text")) -> ()  [unwired: 2 in, 2 out]
                n198 = property on="Set" class="Bool"("BoolText.Text"="设置" ("Boolean Text.Text")) -> ()  [unwired: 2 in, 2 out]
                n199 = property on="exit" class="Bool"("BoolText.Text"="退出" ("Boolean Text.Text")) -> ()  [unwired: 2 in, 2 out]
                n200 = property on="Logout" class="Bool"("BoolText.Text"="登出" ("Boolean Text.Text")) -> ()  [unwired: 2 in, 2 out]
                n201 = property on="Password" class="Str"("Caption.Text"="密码: ") -> ()  [unwired: 2 in, 2 out]
                n202 = property on="Login" class="Bool"("BoolText.Text"="登录" ("Boolean Text.Text")) -> ()  [unwired: 2 in, 2 out]
                n203 = property on="Operator" class="Str"("Caption.Text"="员工") -> ()  [unwired: 2 in, 2 out]
                n204 = property on="Pass" class="Bool (strict)"("Caption.Text"="通过") -> ()  [unwired: 2 in, 2 out]
                n205 = property on="Fail" class="Bool (strict)"("Caption.Text"="失败") -> ()  [unwired: 2 in, 2 out]
                n206 = property on="Start" class="Bool"("BoolText.Text"="开始测试" ("Boolean Text.Text")) -> ()  [unwired: 2 in, 2 out]
                n207 = property on="btnAbort" class="Bool (strict)"("BoolText.Text"="终止测试" ("Boolean Text.Text")) -> ()  [unwired: 2 in, 2 out]
                n208 = property on="process" class="Str"("Caption.Text"="测试类型") -> ()  [unwired: 2 in, 2 out]
                n209 = property on="EndTime" class="Str"("Caption.Text"="测试结束") -> ()  [unwired: 2 in, 2 out]
                n210 = property on="StartTime" class="Str"("Caption.Text"="测试开始") -> ()  [unwired: 2 in, 2 out]
                n211 = property on="UserID" class="Str"("Caption.Text"="员工号: ") -> ()  [unwired: 2 in, 2 out]
                n212 = property on="Report" class="Bool (strict)"("BoolText.Text"="生成报表" ("Caption.Text")) -> ()  [unwired: 2 in, 2 out]
                n213 = property on="RunInfo" class="Str"("Caption.Text"="运行信息") -> ()  [unwired: 2 in, 2 out]
                n214 = property on="orderNum_M" class="Str"("Caption.Text"="订单号") -> ()  [unwired: 2 in, 2 out]
              }
            }
          }
          frame #1 {
            n215 = case shown="\"中文\"" w321 {
              frame "English" {
                n216 = property on="ok_Para" class="Bool"("BoolText.Text"="Test" ("Caption.Text")) -> ()  [unwired: 2 in, 2 out]
                n217 = property on="Cancel_Para" class="Bool"("BoolText.Text"="Cancel" ("Caption.Text")) -> ()  [unwired: 2 in, 2 out]
                n218 = property on="Frame" class="Str"("Caption.Text"="Frame") -> ()  [unwired: 2 in, 2 out]
                n219 = property on="load_Limit" class="DigNum (strict)"("Caption.Text"="Load") -> ()  [unwired: 2 in, 2 out]
                n220 = property on="preload_Action" class="DigNum (strict)"("Caption.Text"="Limit") -> ()  [unwired: 2 in, 2 out]
                n221 = property on="Torque" class="Str"("Caption.Text"="Torque") -> ()  [unwired: 2 in, 2 out]
                n222 = property on="preload_Limit" class="DigNum (strict)"("Caption.Text"="Preload") -> ()  [unwired: 2 in, 2 out]
                n223 = property on="DA_IL" class="DigNum (strict)"("Caption.Text"="Desired") -> ()  [unwired: 2 in, 2 out]
                n224 = property on="Gauge_In" class="DigNum (strict)"("Caption.Text"="Gauge In") -> ()  [unwired: 2 in, 2 out]
                n225 = property on="Gauge_Out" class="DigNum (strict)"("Caption.Text"="Gauge Out") -> ()  [unwired: 2 in, 2 out]
                n226 = property on="Test Date" class="Str"("Caption.Text"="Test Date") -> ()  [unwired: 2 in, 2 out]
                n227 = property on="load_Action" class="DigNum (strict)"("Caption.Text"="Action 1") -> ()  [unwired: 2 in, 2 out]
                n228 = property on="Factor_Action" class="Str"("Caption.Text"="Action 2") -> ()  [unwired: 2 in, 2 out]
                n229 = property on="Operator_test" class="Str"("Caption.Text"="Operator") -> ()  [unwired: 2 in, 2 out]
                n230 = property on="testCount" class="Str"("Caption.Text"="Test Count") -> ()  [unwired: 2 in, 2 out]
                n231 = property on="Add MLFB" class="Bool"("BoolText.Text"="Add" ("Caption.Text")) -> ()  [unwired: 2 in, 2 out]
                n232 = property on="Preload_Release N" class="DigNum (strict)"("Caption.Text"="Limit") -> ()  [unwired: 2 in, 2 out]
                n233 = property on="Load_Limit N" class="DigNum (strict)"("Caption.Text"="Load") -> ()  [unwired: 2 in, 2 out]
                n234 = property on="Frame N" class="Str"("Caption.Text"="Frame") -> ()  [unwired: 2 in, 2 out]
                n235 = property on="Preload_Limit N" class="DigNum (strict)"("Caption.Text"="Preload") -> ()  [unwired: 2 in, 2 out]
              }
              frame "中文" {
                n236 = property on="orderCount" class="Str"("Caption.Text"="订单数量") -> ()  [unwired: 2 in, 2 out]
                n237 = property on="testCount" class="Str"("Caption.Text"="测试数量") -> ()  [unwired: 2 in, 2 out]
                n238 = property on="productCode" class="Str"("Text.Text"="生产代码") -> ()  [unwired: 2 in, 2 out]
                n239 = property on="Factor_Limit" class="Str"("Caption.Text"="电流系数") -> ()  [unwired: 2 in, 2 out]
                n240 = property on="preload_Action" class="DigNum (strict)"("Caption.Text"="极限电流") -> ()  [unwired: 2 in, 2 out]
                n241 = property on="Current_IL" class="DigNum (strict)"("Caption.Text"="测试电流") -> ()  [unwired: 2 in, 2 out]
                n242 = property on="consTime_IL" class="DigNum (strict)"("Caption.Text"="时间常数") -> ()  [unwired: 2 in, 2 out]
                n243 = property on="KG20_IL" class="DigNum (strict)"("Caption.Text"="温度系数") -> ()  [unwired: 2 in, 2 out]
                n244 = property on="Test Date" class="Str"("Caption.Text"="测试日期") -> ()  [unwired: 2 in, 2 out]
                n245 = property on="Gauge_In" class="DigNum (strict)"("Caption.Text"="进线线径") -> ()  [unwired: 2 in, 2 out]
                n246 = property on="Temperature" class="Str"("Caption.Text"="温度") -> ()  [unwired: 2 in, 2 out]
                n247 = property on="ok_Para" class="Bool"("BoolText.Text"="测试" ("Caption.Text")) -> ()  [unwired: 2 in, 2 out]
                n248 = property on="Cancel_Para" class="Bool"("BoolText.Text"="取消" ("Caption.Text")) -> ()  [unwired: 2 in, 2 out]
                n249 = property on="Torque" class="Str"("Caption.Text"="扭矩") -> ()  [unwired: 2 in, 2 out]
                n250 = property on="Frame" class="Str"("Caption.Text"="框架") -> ()  [unwired: 2 in, 2 out]
                n251 = property on="Operator_test" class="Str"("Caption.Text"="操作员") -> ()  [unwired: 2 in, 2 out]
                n252 = property on="orderNum_P" class="Str"("Caption.Text"="订单号") -> ()  [unwired: 2 in, 2 out]
                n253 = property on="preload_Limit" class="DigNum (strict)"("Caption.Text"="预载荷") -> ()  [unwired: 2 in, 2 out]
                n254 = property on="DA_IL" class="DigNum (strict)"("Caption.Text"="期望值") -> ()  [unwired: 2 in, 2 out]
                n255 = property on="load_Limit" class="DigNum (strict)"("Caption.Text"="载荷") -> ()  [unwired: 2 in, 2 out]
              }
            }
          }
          frame #2 {
            n256 = case shown="\"English\"" w362 {
              frame "English" {
                n257 = property on="Factor_Limit N" class="Str"("Caption.Text"="Current Factor") -> ()  [unwired: 2 in, 2 out]
                n258 = property on="KG20_IL N" class="DigNum (strict)"("Caption.Text"="Temp.Factor") -> ()  [unwired: 2 in, 2 out]
                n259 = property on="Current_IL N" class="DigNum (strict)"("Caption.Text"="Current Range") -> ()  [unwired: 2 in, 2 out]
                n260 = property on="consTime_IL N" class="DigNum (strict)"("Caption.Text"="Time Constant") -> ()  [unwired: 2 in, 2 out]
                n261 = property on="curRange N" class="Str"("Caption.Text"="Current Range") -> ()  [unwired: 2 in, 2 out]
                n262 = property on="current" class="DigNum (strict)"("Caption.Text"="Testing Current") -> ()  [unwired: 2 in, 2 out]
                n263 = property on="orderNum_M" class="Str"("Caption.Text"="Order Number") -> ()  [unwired: 2 in, 2 out]
                n264 = property on="orderNum_P" class="Str"("Caption.Text"="Order Number") -> ()  [unwired: 2 in, 2 out]
                n265 = property on="Reference temp" class="DigNum (strict)"("Caption.Text"="Reference Temp") -> ()  [unwired: 2 in, 2 out]
                n266 = property on="consTime_IL" class="DigNum (strict)"("Caption.Text"="Time Constant") -> ()  [unwired: 2 in, 2 out]
                n267 = property on="KG20_IL" class="DigNum (strict)"("Caption.Text"="Temp.Factor") -> ()  [unwired: 2 in, 2 out]
                n268 = property on="Factor_Limit" class="Str"("Caption.Text"="Current Factor") -> ()  [unwired: 2 in, 2 out]
                n269 = property on="Temperature" class="Str"("Caption.Text"="Temperature") -> ()  [unwired: 2 in, 2 out]
                n270 = property on="orderCount" class="Str"("Caption.Text"="Order Count") -> ()  [unwired: 2 in, 2 out]
                n271 = property on="productCode" class="Str"("Text.Text"="Product Code") -> ()  [unwired: 2 in, 2 out]
              }
              frame "中文" {
                n272 = property on="Frame N" class="Str"("Caption.Text"="框架") -> ()  [unwired: 2 in, 2 out]
                n273 = property on="Load_Limit N" class="DigNum (strict)"("Caption.Text"="载荷") -> ()  [unwired: 2 in, 2 out]
                n274 = property on="Resistance N" class="DigNum (strict)"("Caption.Text"="内阻") -> ()  [unwired: 2 in, 2 out]
                n275 = property on="Torque N" class="Str"("Caption.Text"="扭矩" ("Text.Text")) -> ()  [unwired: 2 in, 2 out]
                n276 = property on="Add MLFB" class="Bool"("BoolText.Text"="新增" ("Caption.Text")) -> ()  [unwired: 2 in, 2 out]
                n277 = property on="Reference temp" class="DigNum (strict)"("Caption.Text"="基准温度") -> ()  [unwired: 2 in, 2 out]
                n278 = property on="Gauge_Out" class="DigNum (strict)"("Caption.Text"="出现线径") -> ()  [unwired: 2 in, 2 out]
                n279 = property on="curRange N" class="Str"("Caption.Text"="电流范围") -> ()  [unwired: 2 in, 2 out]
                n280 = property on="reTemperature N" class="DigNum (strict)"("Caption.Text"="基准温度") -> ()  [unwired: 2 in, 2 out]
                n281 = property on="Factor_Limit N" class="Str"("Caption.Text"="电流系数") -> ()  [unwired: 2 in, 2 out]
                n282 = property on="Current_IL N" class="DigNum (strict)"("Caption.Text"="电流范围") -> ()  [unwired: 2 in, 2 out]
                n283 = property on="consTime_IL N" class="DigNum (strict)"("Caption.Text"="时间常数") -> ()  [unwired: 2 in, 2 out]
                n284 = property on="KG20_IL N" class="DigNum (strict)"("Caption.Text"="温度系数") -> ()  [unwired: 2 in, 2 out]
                n285 = property on="Preload_Release N" class="DigNum (strict)"("Caption.Text"="极限电流") -> ()  [unwired: 2 in, 2 out]
                n286 = property on="Load_Release N" class="DigNum (strict)"("Caption.Text"="动作特性") -> ()  [unwired: 2 in, 2 out]
                n287 = property on="load_Action" class="DigNum (strict)"("Caption.Text"="动作特性 1") -> ()  [unwired: 2 in, 2 out]
                n288 = property on="Factor_Action" class="Str"("Caption.Text"="动作特性 2") -> ()  [unwired: 2 in, 2 out]
                n289 = property on="Gauge_In N" class="DigNum (strict)"("Caption.Text"="进线线径") -> ()  [unwired: 2 in, 2 out]
                n290 = property on="Gauge_Out N" class="DigNum (strict)"("Caption.Text"="出线线径") -> ()  [unwired: 2 in, 2 out]
                n291 = property on="curRange E" class="Str"("Caption.Text"="电流范围") -> ()  [unwired: 2 in, 2 out]
              }
            }
          }
          frame #3 {
            n292 = case shown="\"中文\"" w398 {
              frame "English" {
                n293 = property on="DA N" class="DigNum (strict)"("Caption.Text"="Desired") -> ()  [unwired: 2 in, 2 out]
                n294 = property on="Torque N" class="Str"("Caption.Text"="Torque" ("Text.Text")) -> ()  [unwired: 2 in, 2 out]
                n295 = property on="Cancel Add" class="Bool"("BoolText.Text"="Cancel" ("Caption.Text")) -> ()  [unwired: 2 in, 2 out]
                n296 = property on="Load_Release N" class="DigNum (strict)"("Caption.Text"="Action") -> ()  [unwired: 2 in, 2 out]
                n297 = property on="Torque E" class="Str"("Caption.Text"="Torque") -> ()  [unwired: 2 in, 2 out]
                n298 = property on="Frame E" class="Str"("Caption.Text"="Frame") -> ()  [unwired: 2 in, 2 out]
                n299 = property on="Ok_Edit" class="Bool"("BoolText.Text"="Edit" ("Caption.Text")) -> ()  [unwired: 2 in, 2 out]
                n300 = property on="Cancel_Edit" class="Bool"("BoolText.Text"="Cancel" ("Caption.Text")) -> ()  [unwired: 2 in, 2 out]
                n301 = property on="Load_Limit E" class="DigNum (strict)"("Caption.Text"="Load") -> ()  [unwired: 2 in, 2 out]
                n302 = property on="Preload_Action E" class="DigNum (strict)"("Caption.Text"="Limit") -> ()  [unwired: 2 in, 2 out]
                n303 = property on="Gauge_In N" class="DigNum (strict)"("Caption.Text"="Gauge In") -> ()  [unwired: 2 in, 2 out]
                n304 = property on="Load_Action E" class="DigNum (strict)"("Caption.Text"="Action") -> ()  [unwired: 2 in, 2 out]
                n305 = property on="DA E" class="DigNum (strict)"("Caption.Text"="Desired") -> ()  [unwired: 2 in, 2 out]
                n306 = property on="Preload_Limit E" class="DigNum (strict)"("Caption.Text"="Preload") -> ()  [unwired: 2 in, 2 out]
                n307 = property on="btnDelete" class="Bool"("BoolText.Text"="Delete" ("Caption.Text")) -> ()  [unwired: 2 in, 2 out]
                n308 = property on="Gauge_Out N" class="DigNum (strict)"("Caption.Text"="Gauge out") -> ()  [unwired: 2 in, 2 out]
                n309 = property on="Current_IL" class="DigNum (strict)"("Caption.Text"="Test Current") -> ()  [unwired: 2 in, 2 out]
                n310 = property on="Resistance N" class="DigNum (strict)"("Caption.Text"="Resistance") -> ()  [unwired: 2 in, 2 out]
                n311 = property on="FactorLimit E" class="Str"("Caption.Text"="Current Factor") -> ()  [unwired: 2 in, 2 out]
                n312 = property on="circuitRs E" class="DigNum (strict)"("Caption.Text"="Resistance") -> ()  [unwired: 2 in, 2 out]
              }
              frame "中文" {
                n313 = property on="Frame E" class="Str"("Caption.Text"="框架") -> ()  [unwired: 2 in, 2 out]
                n314 = property on="Cancel Add" class="Bool"("BoolText.Text"="取消" ("Caption.Text")) -> ()  [unwired: 2 in, 2 out]
                n315 = property on="Load_Limit E" class="DigNum (strict)"("Caption.Text"="载荷") -> ()  [unwired: 2 in, 2 out]
                n316 = property on="circuitRs E" class="DigNum (strict)"("Caption.Text"="内阻") -> ()  [unwired: 2 in, 2 out]
                n317 = property on="Torque E" class="Str"("Caption.Text"="扭矩") -> ()  [unwired: 2 in, 2 out]
                n318 = property on="consTime_IL E" class="DigNum (strict)"("Caption.Text"="时间常数") -> ()  [unwired: 2 in, 2 out]
                n319 = property on="KG_IL E" class="DigNum (strict)"("Caption.Text"="温度系数") -> ()  [unwired: 2 in, 2 out]
                n320 = property on="FactorLimit E" class="Str"("Caption.Text"="电流系数") -> ()  [unwired: 2 in, 2 out]
                n321 = property on="Preload_Action E" class="DigNum (strict)"("Caption.Text"="极限电流") -> ()  [unwired: 2 in, 2 out]
                n322 = property on="Load_Action E" class="DigNum (strict)"("Caption.Text"="动作特性") -> ()  [unwired: 2 in, 2 out]
                n323 = property on="Preload_Limit N" class="DigNum (strict)"("Caption.Text"="预载荷") -> ()  [unwired: 2 in, 2 out]
                n324 = property on="DA E" class="DigNum (strict)"("Caption.Text"="期望值") -> ()  [unwired: 2 in, 2 out]
                n325 = property on="Preload_Limit E" class="DigNum (strict)"("Caption.Text"="预载荷") -> ()  [unwired: 2 in, 2 out]
                n326 = property on="DA N" class="DigNum (strict)"("Caption.Text"="期望值") -> ()  [unwired: 2 in, 2 out]
                n327 = property on="Current_IL E" class="DigNum (strict)"("Caption.Text"="电流范围") -> ()  [unwired: 2 in, 2 out]
                n328 = property on="txtPassword" class="Str"("Caption.Text"="密码") -> ()  [unwired: 2 in, 2 out]
                n329 = property on="btnEditUser" class="Bool"("BoolText.Text"="编辑" ("Caption.Text")) -> ()  [unwired: 2 in, 2 out]
                n330 = property on="btnDeleteUser" class="Bool"("BoolText.Text"="删除" ("Caption.Text")) -> ()  [unwired: 2 in, 2 out]
                n331 = property on="btnNewUser" class="Bool"("BoolText.Text"="新建" ("Caption.Text")) -> ()  [unwired: 2 in, 2 out]
                n332 = property on="btnReadUser" class="Bool"("BoolText.Text"="读取" ("Boolean Text.Text")) -> ()  [unwired: 2 in, 2 out]
              }
            }
          }
          frame #4 {
            n333 = case shown="\"中文\"" w439 {
              frame "English" {
                n334 = property on="Gauge_In E" class="DigNum (strict)"("Caption.Text"="Gauge In") -> ()  [unwired: 2 in, 2 out]
                n335 = property on="valueCalibra" class="DigNum (strict)"("Caption.Text"="Test Value") -> ()  [unwired: 2 in, 2 out]
                n336 = property on="btnCalTpr" class="Bool"("BoolText.Text"="Meassure" ("Boolean Text.Text")) -> ()  [unwired: 2 in, 2 out]
                n337 = property on="txtPassword" class="Str"("Caption.Text"="Password") -> ()  [unwired: 2 in, 2 out]
                n338 = property on="Authority" class="Enum (strict)"("Caption.Text"="Authority") -> ()  [unwired: 2 in, 2 out]
                n339 = property on="btnReadUser" class="Bool"("BoolText.Text"="Read" ("Boolean Text.Text")) -> ()  [unwired: 2 in, 2 out]
                n340 = property on="readCalibra" class="Bool"("BoolText.Text"="Read" ("Caption.Text")) -> ()  [unwired: 2 in, 2 out]
                n341 = property on="abortCalibra" class="Bool"("BoolText.Text"="Abort" ("Caption.Text")) -> ()  [unwired: 2 in, 2 out]
                n342 = property on="btnNewUser" class="Bool"("BoolText.Text"="New" ("Caption.Text")) -> ()  [unwired: 2 in, 2 out]
                n343 = property on="btnEditUser" class="Bool"("BoolText.Text"="Edit" ("Caption.Text")) -> ()  [unwired: 2 in, 2 out]
                n344 = property on="txtID" class="Str"("Caption.Text"="UserID") -> ()  [unwired: 2 in, 2 out]
                n345 = property on="btnCalibration" class="Bool"("BoolText.Text"="Output" ("Boolean Text.Text")) -> ()  [unwired: 2 in, 2 out]
                n346 = property on="txtName" class="Str"("Caption.Text"="Name") -> ()  [unwired: 2 in, 2 out]
                n347 = property on="btnDeleteUser" class="Bool"("BoolText.Text"="Delete" ("Caption.Text")) -> ()  [unwired: 2 in, 2 out]
                n348 = property on="btnReturn" class="Bool"("BoolText.Text"="Return" ("Caption.Text")) -> ()  [unwired: 2 in, 2 out]
                n349 = property on="reTemperature N" class="DigNum (strict)"("Caption.Text"="Reference Temp") -> ()  [unwired: 2 in, 2 out]
                n350 = property on="releaseRs" class="DigNum (strict)"("Caption.Text"="Trip Resistance") -> ()  [unwired: 2 in, 2 out]
                n351 = property on="releaseRs E" class="DigNum (strict)"("Caption.Text"="Trip Resistance") -> ()  [unwired: 2 in, 2 out]
                n352 = property on="reTemperature E" class="DigNum (strict)"("Caption.Text"="Reference Temp") -> ()  [unwired: 2 in, 2 out]
                n353 = property on="curRange E" class="Str"("Caption.Text"="Current Range") -> ()  [unwired: 2 in, 2 out]
              }
              frame "中文" {
                n354 = property on="btnCalibration" class="Bool"("Caption.Text"="电流校验") -> ()  [unwired: 2 in, 2 out]
                n355 = property on="vlCalTpr" class="DigNum (strict)"("Caption.Text"="实测温度") -> ()  [unwired: 2 in, 2 out]
                n356 = property on="btnCalTpr" class="Bool"("BoolText.Text"="读取温度" ("Boolean Text.Text")) -> ()  [unwired: 2 in, 2 out]
                n357 = property on="Gauge_In E" class="DigNum (strict)"("Caption.Text"="进线线径") -> ()  [unwired: 2 in, 2 out]
                n358 = property on="Gauge_Out E" class="DigNum (strict)"("Caption.Text"="出线线径") -> ()  [unwired: 2 in, 2 out]
                n359 = property on="btnCalibration" class="Bool"("BoolText.Text"="输出" ("Boolean Text.Text")) -> ()  [unwired: 2 in, 2 out]
                n360 = property on="readCalibra" class="Bool"("BoolText.Text"="读取" ("Caption.Text")) -> ()  [unwired: 2 in, 2 out]
                n361 = property on="abortCalibra" class="Bool"("BoolText.Text"="停止" ("Caption.Text")) -> ()  [unwired: 2 in, 2 out]
                n362 = property on="Authority" class="Enum (strict)"("Caption.Text"="权限") -> ()  [unwired: 2 in, 2 out]
                n363 = property on="txtName" class="Str"("Caption.Text"="姓名") -> ()  [unwired: 2 in, 2 out]
                n364 = property on="DisableCurtain" class="Bool (strict)"("Caption.Text"="关闭安全光幕") -> ()  [unwired: 2 in, 2 out]
                n365 = property on="ThermalTmFrame" class="Str"("Caption.Text"="快速时间范围") -> ()  [unwired: 2 in, 2 out]
                n366 = property on="thermoRs" class="DigNum (strict)"("Caption.Text"="热元件电阻值") -> ()  [unwired: 2 in, 2 out]
                n367 = property on="thermoRs E" class="DigNum (strict)"("Caption.Text"="热元件电阻值") -> ()  [unwired: 2 in, 2 out]
                n368 = property on="current" class="DigNum (strict)"("Caption.Text"="当前测试电流") -> ()  [unwired: 2 in, 2 out]
                n369 = property on="Ok_Edit" class="Bool"("BoolText.Text"="编辑" ("Caption.Text")) -> ()  [unwired: 2 in, 2 out]
                n370 = property on="Cancel_Edit" class="Bool"("BoolText.Text"="取消" ("Caption.Text")) -> ()  [unwired: 2 in, 2 out]
                n371 = property on="btnDelete" class="Bool"("BoolText.Text"="删除" ("Caption.Text")) -> ()  [unwired: 2 in, 2 out]
                n372 = property on="setCalibra" class="DigNum (strict)"("Caption.Text"="设定值") -> ()  [unwired: 2 in, 2 out]
                n373 = property on="valueCalibra" class="DigNum (strict)"("Caption.Text"="测试值") -> ()  [unwired: 2 in, 2 out]
              }
            }
          }
          frame #5 {
            n374 = case shown="\"English\"" w480 {
              frame "中文", Default {
                n375 = property on="btnReadLCConfig" class="Bool"("Caption.Text"="安全光幕") -> ()  [unwired: 2 in, 2 out]
                n376 = property on="DelayByUser" class="Str"("Caption.Text"="自恢复时间") -> ()  [unwired: 2 in, 2 out]
                n377 = property on="DelayToFailed" class="Str"("Caption.Text"="误触发极限") -> ()  [unwired: 2 in, 2 out]
                n378 = property on="btnReturn" class="Bool"("BoolText.Text"="返回主界面" ("Caption.Text")) -> ()  [unwired: 2 in, 2 out]
                n379 = property on="reTemperature E" class="DigNum (strict)"("Caption.Text"="基准温度") -> ()  [unwired: 2 in, 2 out]
                n380 = property on="btnReadLCConfig" class="Bool"("BoolText.Text"="读取" ("Boolean Text.Text")) -> ()  [unwired: 2 in, 2 out]
                n381 = property on="btnEditLCConfig" class="Bool"("BoolText.Text"="编辑" ("Boolean Text.Text")) -> ()  [unwired: 2 in, 2 out]
                n382 = property on="txtID" class="Str"("Caption.Text"="用户ID") -> ()  [unwired: 2 in, 2 out]
                n383 = property on="AccelerationTime" class="Str"("Caption.Text"="起动时间") -> ()  [unwired: 2 in, 2 out]
                n384 = property on="btnCalTpr" class="Bool"("Caption.Text"="温度校验") -> ()  [unwired: 2 in, 2 out]
                n385 = property on="releaseRs E" class="DigNum (strict)"("Caption.Text"="电流脱扣器电阻值") -> ()  [unwired: 2 in, 2 out]
                n386 = property on="releaseRs" class="DigNum (strict)"("Caption.Text"="电流脱扣器电阻值") -> ()  [unwired: 2 in, 2 out]
                n387 = property on="totalSec" class="Str"("Caption.Text"="最长测试时间") -> ()  [unwired: 2 in, 2 out]
              }
              frame "English" {
                n388 = property on="ThermalTmFrame" class="Str"("Caption.Text"="Thermal Time Frame") -> ()  [unwired: 2 in, 2 out]
                n389 = property on="thermoRs E" class="DigNum (strict)"("Caption.Text"="Thermo Resistance") -> ()  [unwired: 2 in, 2 out]
                n390 = property on="DisableCurtain" class="Bool (strict)"("Caption.Text"="DisableSafetyCurtain") -> ()  [unwired: 2 in, 2 out]
                n391 = property on="thermoRs" class="DigNum (strict)"("Caption.Text"="Thermo Resistance") -> ()  [unwired: 2 in, 2 out]
                n392 = property on="btnCalTpr" class="Bool"("Caption.Text"="Temprature Calibration") -> ()  [unwired: 2 in, 2 out]
                n393 = property on="KG_IL E" class="DigNum (strict)"("Caption.Text"="Temp.Factor") -> ()  [unwired: 2 in, 2 out]
                n394 = property on="Current_IL E" class="DigNum (strict)"("Caption.Text"="Current Range") -> ()  [unwired: 2 in, 2 out]
                n395 = property on="consTime_IL E" class="DigNum (strict)"("Caption.Text"="Time Constant") -> ()  [unwired: 2 in, 2 out]
                n396 = property on="btnCalibration" class="Bool"("Caption.Text"="Power Calibration") -> ()  [unwired: 2 in, 2 out]
                n397 = property on="AccelerationTime" class="Str"("Caption.Text"="Acceleration Time") -> ()  [unwired: 2 in, 2 out]
                n398 = property on="btnReadLCConfig" class="Bool"("Caption.Text"="Safety Curtain") -> ()  [unwired: 2 in, 2 out]
                n399 = property on="DelayByUser" class="Str"("Caption.Text"="TimetoEnabe") -> ()  [unwired: 2 in, 2 out]
                n400 = property on="DelayToFailed" class="Str"("Caption.Text"="MaxtoFailed") -> ()  [unwired: 2 in, 2 out]
                n401 = property on="vlCalTpr" class="DigNum (strict)"("Caption.Text"="Temprature") -> ()  [unwired: 2 in, 2 out]
                n402 = property on="Gauge_Out E" class="DigNum (strict)"("Caption.Text"="Gauge Out") -> ()  [unwired: 2 in, 2 out]
              }
            }
          }
          frame #6 {
            n403 = case shown="\"English\"" w509 {
              frame "中文", Default {
                n404 = property on="TestModel" class="RadioBtnsControl (strict)"() -> ("Controls[]"=w511:refnum<vi>[])  [unwired: 2 in, 2 out]
                n405 = for {
                  tunnel: w511 -> [w514] mode=indexing
                  i -> [w515]
                  n406 = case shown="2" w515 {
                    tunnel: w514 -> [w517 w519 w521 w523 w525 w527]
                    tunnel: [w517 w519 w521 w523 w525 w527] -> w513
                    tunnel: ["极限电流小档" "极限电流大档" "动作特性1 小档" "动作特性1 大档" "动作特性2 小档" "动作特性2 大档"] -> w512
                    frame 0, Default {
                    }
                    frame 1 {
                    }
                    frame 2 {
                    }
                    frame 3 {
                    }
                    frame 4 {
                    }
                    frame 5 {
                    }
                  }
                  n407 = property class="Ctl"(reference=w513, "Caption.Text"=w512) -> ()  [unwired: 1 in, 2 out]
                }
                n408 = property on="parameter" class="MCListbox (strict)"("RowHdrs[]"=string[] ["电流系数", "温度补偿系数", "当前温度", "脱扣数量"] ("Row Header Strings[]")) -> ()  [unwired: 2 in, 2 out]
              }
              frame "English" {
                n409 = property on="btnReadLCConfig" class="Bool"("BoolText.Text"="Read" ("Boolean Text.Text")) -> ()  [unwired: 2 in, 2 out]
                n410 = property on="btnEditLCConfig" class="Bool"("BoolText.Text"="Edit" ("Boolean Text.Text")) -> ()  [unwired: 2 in, 2 out]
                n411 = property on="setCalibra" class="DigNum (strict)"("Caption.Text"="Output") -> ()  [unwired: 2 in, 2 out]
                n412 = property on="TestModel" class="RadioBtnsControl (strict)"() -> ("Controls[]"=w528:refnum<vi>[])  [unwired: 2 in, 2 out]
                n413 = for {
                  tunnel: w528 -> [w535] mode=indexing
                  i -> [w536]
                  n414 = case shown="5" w536 {
                    tunnel: w535 -> [w538 w540 w542 w544 w546 w548]
                    tunnel: [w538 w540 w542 w544 w546 w548] -> w534
                    tunnel: ["Limit Lower" "Limit Upper" "Action 1 Lower" "Action 1 Upper" "Action 2 Lower" "Action 2 Upper"] -> w533
                    frame 0, Default {
                    }
                    frame 1 {
                    }
                    frame 2 {
                    }
                    frame 3 {
                    }
                    frame 4 {
                    }
                    frame 5 {
                    }
                  }
                  n415 = property class="Ctl"(reference=w534, "Caption.Text"=w533) -> ()  [unwired: 1 in, 2 out]
                }
                n416 = property on="parameter" class="MCListbox (strict)"("RowHdrs[]"=string[] ["Limit Factor", "Temp.Factor", "Temprature", "Tripped"] ("Row Header Strings[]")) -> ()  [unwired: 2 in, 2 out]
              }
            }
          }
        }
      }
      frame "UI" {
        n417 = event shown="[14] \"Login\": Value Change" {
          selector: _ -> [_ _ _ _ _ _ _ _ _ _ _ _ _ _ _ _ _ _ _ _ _ _ _ _ _ _ _ _ _ _]
          dyn-events: _ -> [_ _ _ _ _ _ _ _ _ _ _ _ _ _ _ _ _ _ _ _ _ _ _ _ _ _ _ _ _ _]
          timeout: -1 ("Timeout") -> [_ _ _ _ _ _ _ _ _ _ _ _ _ _ _ _ _ _ _ _ _ _ _ _ _ _ _ _ _ _]
          tunnel: [w560 T10."Parameter" ("Tab") w576 w591 T10."Test" ("Tab") w600 T10."Test" ("Tab") T10."Add MLFB" ("Tab") T10."Edit MLFB" ("Tab") T10."Calibration Power" ("Tab") w625 w628 w641 T10."Test" ("Tab") w653 T10."Login" ("Tab") w666 w670 w676 w679 T10."Test" ("Tab") w689 w694 w700 w706 w711 w719 w723 w730 w738] -> w550
          tunnel: w557 -> [w560 _ w576 w591 _ w600 _ _ _ _ w625 w628 w641 _ w653 _ w666 w670 w676 w679 _ w689 w694 w700 w706 w711 w719 w723 w730 w738]
          tunnel: w556 -> [w558 w565 w567 w592 w596 w601 w608 w612 w615 w621 w624 w629 w633 w651 w655 w661 w663 w669 w675 w680 w684 w690 w693 w701 w707 w713 w718 w722 w728 w740]
          tunnel: w555 -> [w561 w566 w571 w593 w597 w602 w606 w611 w616 w620 w623 w630 w640 w650 w652 w662 w665 w671 w677 w681 w685 w687 w695 w702 w708 w712 w717 w721 w731 w732]
          tunnel: [w561 w566 w571 w593 w597 w602 w606 w611 w616 w620 w623 w630 w640 w650 w652 w662 w665 w671 w677 w681 w685 w687 w695 w702 w708 w712 w717 w721 w731 w733] -> w554
          tunnel: [w558 w565 w569 w592 w596 w601 w608 w612 w615 w621 w624 w629 w634 w651 w655 w660 w663 w669 w675 w680 w684 w690 w693 w701 w707 w713 w718 w722 w728 w740] -> w553
          tunnel: [w559 w563 w570 w590 w595 w599 w607 w609 w614 w618 w622 w627 w636 w649 w654 w658 w664 w668 w674 w678 w683 w688 w692 w699 w705 w710 w716 w720 w729 w739] -> w549
          tunnel: w551 -> [_ _ w568 _ _ _ _ _ _ _ _ _ _ _ _ _ _ _ _ _ _ _ _ _ _ _ _ _ _ _]
          event Timeout {
            w559 = T16[] [enum."Procedure"] items=["Initial_Data", "Initial_HMI", "Language", "UI", "Login", "Authority", "Clear", "Initial Test Data", "Initial Test Data1", "Initial Test UI", "Test Parameter", "PowerRemote", "PowerON", "PowerCalibration", "PowerOFF", "Temperature", "TempOffset", "Trip", "ShowInfo", "Finish?", "Period?", "LoopCurrent", "Procedure", "KGR", "Passed", "Failed", "MLFB Decoding", "MLFB Test Info", "MLFB Edit Info", "MLFB Edit", "MLFB Insert", "MLFB Delete", "ReportGeneralInfo", "ReportResultInfo", "ReportPath", "Generate Report", "Print Report", "New User", "Edit User", "Delete User", "Read User", "Voltage", "Time", "Current Calibration", "ErrorHandle", "StartTest", "ActiveLightCur", "Uninstall Record", "Get Uninstall Count", "Abort Test", "Test Model?", "CheckLoopCurrent", "Release HW Source", "Exit", "Close DB Connection", "Test UI BTN Status", "unTest UI BTN Status", "Disable All BTN", "AbortCalibration", "TprCalibration", "ClearReportInfo", "Set Uninstall", "TestResult", "SetLightCur", "CheckVoltage", "ShowTripTime"]
            n418 = event-data() -> ()  [unwired: 1 in, 1 out]
          }
          event "Start": Value Change {
            w563 = T16[] [enum."Clear", enum."Authority", enum."Test Model?", enum."Procedure"] items=["Initial_Data", "Initial_HMI", "Language", "UI", "Login", "Authority", "Clear", "Initial Test Data", "Initial Test Data1", "Initial Test UI", "Test Parameter", "PowerRemote", "PowerON", "PowerCalibration", "PowerOFF", "Temperature", "TempOffset", "Trip", "ShowInfo", "Finish?", "Period?", "LoopCurrent", "Procedure", "KGR", "Passed", "Failed", "MLFB Decoding", "MLFB Test Info", "MLFB Edit Info", "MLFB Edit", "MLFB Insert", "MLFB Delete", "ReportGeneralInfo", "ReportResultInfo", "ReportPath", "Generate Report", "Print Report", "New User", "Edit User", "Delete User", "Read User", "Voltage", "Time", "Current Calibration", "ErrorHandle", "StartTest", "ActiveLightCur", "Uninstall Record", "Get Uninstall Count", "Abort Test", "Test Model?", "CheckLoopCurrent", "Release HW Source", "Exit", "Close DB Connection", "Test UI BTN Status", "unTest UI BTN Status", "Disable All BTN", "AbortCalibration", "TprCalibration", "ClearReportInfo", "Set Uninstall", "TestResult", "SetLightCur", "CheckVoltage", "ShowTripTime"]
            n419 = event-data() -> ()  [unwired: 1 in, 1 out]
            n420 = property on="ok_Para" class="Bool"("DisabledEnum"=T18."Disabled and Grayed Out" ("Disabled")) -> ()  [unwired: 2 in, 2 out]
          }
          event "MLFB": Value Change {
            n421 = event-data() -> ("NewVal"=w572:string)  [unwired: 1 in]
            n422 = String Length(string=w572) -> (length=w574:i32)
            n423 = Equal?(x=w574, y=13) -> (x = y?=w575:bool)
            n424 = case shown="True" w575 {
              tunnel: [w581 w589] -> w570
              tunnel: [w577 w588] -> w569
              tunnel: w568 -> [w580 _]
              tunnel: w567 -> [w577 w586]
              frame False {
                w581 = T16[] [enum."Procedure"] items=["Initial_Data", "Initial_HMI", "Language", "UI", "Login", "Authority", "Clear", "Initial Test Data", "Initial Test Data1", "Initial Test UI", "Test Parameter", "PowerRemote", "PowerON", "PowerCalibration", "PowerOFF", "Temperature", "TempOffset", "Trip", "ShowInfo", "Finish?", "Period?", "LoopCurrent", "Procedure", "KGR", "Passed", "Failed", "MLFB Decoding", "MLFB Test Info", "MLFB Edit Info", "MLFB Edit", "MLFB Insert", "MLFB Delete", "ReportGeneralInfo", "ReportResultInfo", "ReportPath", "Generate Report", "Print Report", "New User", "Edit User", "Delete User", "Read User", "Voltage", "Time", "Current Calibration", "ErrorHandle", "StartTest", "ActiveLightCur", "Uninstall Record", "Get Uninstall Count", "Abort Test", "Test Model?", "CheckLoopCurrent", "Release HW Source", "Exit", "Close DB Connection", "Test UI BTN Status", "unTest UI BTN Status", "Disable All BTN", "AbortCalibration", "TprCalibration", "ClearReportInfo", "Set Uninstall", "TestResult", "SetLightCur", "CheckVoltage", "ShowTripTime"]
                n425 = case shown="\"English\"" w580 {
                  tunnel: ["MLFB无效" "Invalid MLFB"] -> w579
                  tunnel: ["确定" "OK"] -> w578
                  frame "中文", Default {
                  }
                  frame "English" {
                  }
                }
                n426 = One Button Dialog(message=w579, button name ("OK")=w578) -> ()  [unwired: 1 out]
              }
              frame True {
                w589 = T16[] [enum."MLFB Decoding", enum."Temperature", enum."MLFB Test Info", enum."Get Uninstall Count", enum."Procedure"] items=["Initial_Data", "Initial_HMI", "Language", "UI", "Login", "Authority", "Clear", "Initial Test Data", "Initial Test Data1", "Initial Test UI", "Test Parameter", "PowerRemote", "PowerON", "PowerCalibration", "PowerOFF", "Temperature", "TempOffset", "Trip", "ShowInfo", "Finish?", "Period?", "LoopCurrent", "Procedure", "KGR", "Passed", "Failed", "MLFB Decoding", "MLFB Test Info", "MLFB Edit Info", "MLFB Edit", "MLFB Insert", "MLFB Delete", "ReportGeneralInfo", "ReportResultInfo", "ReportPath", "Generate Report", "Print Report", "New User", "Edit User", "Delete User", "Read User", "Voltage", "Time", "Current Calibration", "ErrorHandle", "StartTest", "ActiveLightCur", "Uninstall Record", "Get Uninstall Count", "Abort Test", "Test Model?", "CheckLoopCurrent", "Release HW Source", "Exit", "Close DB Connection", "Test UI BTN Status", "unTest UI BTN Status", "Disable All BTN", "AbortCalibration", "TprCalibration", "ClearReportInfo", "Set Uninstall", "TestResult", "SetLightCur", "CheckVoltage", "ShowTripTime"]
                n427 = Bundle By Name(cluster=w586, "parameter.MLFB Info.MLFB"="MLFB") -> (w588:T3)
              }
            }
          }
          event "ok_Para": Value Change {
            w590 = T16[] [enum."StartTest"] items=["Initial_Data", "Initial_HMI", "Language", "UI", "Login", "Authority", "Clear", "Initial Test Data", "Initial Test Data1", "Initial Test UI", "Test Parameter", "PowerRemote", "PowerON", "PowerCalibration", "PowerOFF", "Temperature", "TempOffset", "Trip", "ShowInfo", "Finish?", "Period?", "LoopCurrent", "Procedure", "KGR", "Passed", "Failed", "MLFB Decoding", "MLFB Test Info", "MLFB Edit Info", "MLFB Edit", "MLFB Insert", "MLFB Delete", "ReportGeneralInfo", "ReportResultInfo", "ReportPath", "Generate Report", "Print Report", "New User", "Edit User", "Delete User", "Read User", "Voltage", "Time", "Current Calibration", "ErrorHandle", "StartTest", "ActiveLightCur", "Uninstall Record", "Get Uninstall Count", "Abort Test", "Test Model?", "CheckLoopCurrent", "Release HW Source", "Exit", "Close DB Connection", "Test UI BTN Status", "unTest UI BTN Status", "Disable All BTN", "AbortCalibration", "TprCalibration", "ClearReportInfo", "Set Uninstall", "TestResult", "SetLightCur", "CheckVoltage", "ShowTripTime"]
            n428 = event-data() -> ()  [unwired: 1 in, 1 out]
          }
          event "Cancel_Para": Value Change {
            w595 = T16[] [enum."Clear", enum."Procedure"] items=["Initial_Data", "Initial_HMI", "Language", "UI", "Login", "Authority", "Clear", "Initial Test Data", "Initial Test Data1", "Initial Test UI", "Test Parameter", "PowerRemote", "PowerON", "PowerCalibration", "PowerOFF", "Temperature", "TempOffset", "Trip", "ShowInfo", "Finish?", "Period?", "LoopCurrent", "Procedure", "KGR", "Passed", "Failed", "MLFB Decoding", "MLFB Test Info", "MLFB Edit Info", "MLFB Edit", "MLFB Insert", "MLFB Delete", "ReportGeneralInfo", "ReportResultInfo", "ReportPath", "Generate Report", "Print Report", "New User", "Edit User", "Delete User", "Read User", "Voltage", "Time", "Current Calibration", "ErrorHandle", "StartTest", "ActiveLightCur", "Uninstall Record", "Get Uninstall Count", "Abort Test", "Test Model?", "CheckLoopCurrent", "Release HW Source", "Exit", "Close DB Connection", "Test UI BTN Status", "unTest UI BTN Status", "Disable All BTN", "AbortCalibration", "TprCalibration", "ClearReportInfo", "Set Uninstall", "TestResult", "SetLightCur", "CheckVoltage", "ShowTripTime"]
            n429 = event-data() -> ()  [unwired: 1 in, 1 out]
          }
          event "Add MLFB": Value Change {
            n430 = event-data() -> ("NewVal"=w598:bool)  [unwired: 1 in]
            n431 = case shown="False" w598 {
              tunnel: [w603 w604] -> w599
              frame False {
                w603 = T16[] [enum."Procedure"] items=["Initial_Data", "Initial_HMI", "Language", "UI", "Login", "Authority", "Clear", "Initial Test Data", "Initial Test Data1", "Initial Test UI", "Test Parameter", "PowerRemote", "PowerON", "PowerCalibration", "PowerOFF", "Temperature", "TempOffset", "Trip", "ShowInfo", "Finish?", "Period?", "LoopCurrent", "Procedure", "KGR", "Passed", "Failed", "MLFB Decoding", "MLFB Test Info", "MLFB Edit Info", "MLFB Edit", "MLFB Insert", "MLFB Delete", "ReportGeneralInfo", "ReportResultInfo", "ReportPath", "Generate Report", "Print Report", "New User", "Edit User", "Delete User", "Read User", "Voltage", "Time", "Current Calibration", "ErrorHandle", "StartTest", "ActiveLightCur", "Uninstall Record", "Get Uninstall Count", "Abort Test", "Test Model?", "CheckLoopCurrent", "Release HW Source", "Exit", "Close DB Connection", "Test UI BTN Status", "unTest UI BTN Status", "Disable All BTN", "AbortCalibration", "TprCalibration", "ClearReportInfo", "Set Uninstall", "TestResult", "SetLightCur", "CheckVoltage", "ShowTripTime"]
              }
              frame True {
                w604 = T16[] [enum."MLFB Insert", enum."Clear", enum."Procedure"] items=["Initial_Data", "Initial_HMI", "Language", "UI", "Login", "Authority", "Clear", "Initial Test Data", "Initial Test Data1", "Initial Test UI", "Test Parameter", "PowerRemote", "PowerON", "PowerCalibration", "PowerOFF", "Temperature", "TempOffset", "Trip", "ShowInfo", "Finish?", "Period?", "LoopCurrent", "Procedure", "KGR", "Passed", "Failed", "MLFB Decoding", "MLFB Test Info", "MLFB Edit Info", "MLFB Edit", "MLFB Insert", "MLFB Delete", "ReportGeneralInfo", "ReportResultInfo", "ReportPath", "Generate Report", "Print Report", "New User", "Edit User", "Delete User", "Read User", "Voltage", "Time", "Current Calibration", "ErrorHandle", "StartTest", "ActiveLightCur", "Uninstall Record", "Get Uninstall Count", "Abort Test", "Test Model?", "CheckLoopCurrent", "Release HW Source", "Exit", "Close DB Connection", "Test UI BTN Status", "unTest UI BTN Status", "Disable All BTN", "AbortCalibration", "TprCalibration", "ClearReportInfo", "Set Uninstall", "TestResult", "SetLightCur", "CheckVoltage", "ShowTripTime"]
              }
            }
          }
          event "Cancel Add": Value Change {
            w607 = T16[] [enum."Clear", enum."Procedure"] items=["Initial_Data", "Initial_HMI", "Language", "UI", "Login", "Authority", "Clear", "Initial Test Data", "Initial Test Data1", "Initial Test UI", "Test Parameter", "PowerRemote", "PowerON", "PowerCalibration", "PowerOFF", "Temperature", "TempOffset", "Trip", "ShowInfo", "Finish?", "Period?", "LoopCurrent", "Procedure", "KGR", "Passed", "Failed", "MLFB Decoding", "MLFB Test Info", "MLFB Edit Info", "MLFB Edit", "MLFB Insert", "MLFB Delete", "ReportGeneralInfo", "ReportResultInfo", "ReportPath", "Generate Report", "Print Report", "New User", "Edit User", "Delete User", "Read User", "Voltage", "Time", "Current Calibration", "ErrorHandle", "StartTest", "ActiveLightCur", "Uninstall Record", "Get Uninstall Count", "Abort Test", "Test Model?", "CheckLoopCurrent", "Release HW Source", "Exit", "Close DB Connection", "Test UI BTN Status", "unTest UI BTN Status", "Disable All BTN", "AbortCalibration", "TprCalibration", "ClearReportInfo", "Set Uninstall", "TestResult", "SetLightCur", "CheckVoltage", "ShowTripTime"]
            n432 = event-data() -> ()  [unwired: 1 in, 1 out]
          }
          event "New": Value Change {
            w609 = T16[] [enum."Clear", enum."Procedure"] items=["Initial_Data", "Initial_HMI", "Language", "UI", "Login", "Authority", "Clear", "Initial Test Data", "Initial Test Data1", "Initial Test UI", "Test Parameter", "PowerRemote", "PowerON", "PowerCalibration", "PowerOFF", "Temperature", "TempOffset", "Trip", "ShowInfo", "Finish?", "Period?", "LoopCurrent", "Procedure", "KGR", "Passed", "Failed", "MLFB Decoding", "MLFB Test Info", "MLFB Edit Info", "MLFB Edit", "MLFB Insert", "MLFB Delete", "ReportGeneralInfo", "ReportResultInfo", "ReportPath", "Generate Report", "Print Report", "New User", "Edit User", "Delete User", "Read User", "Voltage", "Time", "Current Calibration", "ErrorHandle", "StartTest", "ActiveLightCur", "Uninstall Record", "Get Uninstall Count", "Abort Test", "Test Model?", "CheckLoopCurrent", "Release HW Source", "Exit", "Close DB Connection", "Test UI BTN Status", "unTest UI BTN Status", "Disable All BTN", "AbortCalibration", "TprCalibration", "ClearReportInfo", "Set Uninstall", "TestResult", "SetLightCur", "CheckVoltage", "ShowTripTime"]
            n433 = event-data() -> ()  [unwired: 1 in, 1 out]
          }
          event "Edit": Value Change {
            w614 = T16[] [enum."Clear", enum."Procedure"] items=["Initial_Data", "Initial_HMI", "Language", "UI", "Login", "Authority", "Clear", "Initial Test Data", "Initial Test Data1", "Initial Test UI", "Test Parameter", "PowerRemote", "PowerON", "PowerCalibration", "PowerOFF", "Temperature", "TempOffset", "Trip", "ShowInfo", "Finish?", "Period?", "LoopCurrent", "Procedure", "KGR", "Passed", "Failed", "MLFB Decoding", "MLFB Test Info", "MLFB Edit Info", "MLFB Edit", "MLFB Insert", "MLFB Delete", "ReportGeneralInfo", "ReportResultInfo", "ReportPath", "Generate Report", "Print Report", "New User", "Edit User", "Delete User", "Read User", "Voltage", "Time", "Current Calibration", "ErrorHandle", "StartTest", "ActiveLightCur", "Uninstall Record", "Get Uninstall Count", "Abort Test", "Test Model?", "CheckLoopCurrent", "Release HW Source", "Exit", "Close DB Connection", "Test UI BTN Status", "unTest UI BTN Status", "Disable All BTN", "AbortCalibration", "TprCalibration", "ClearReportInfo", "Set Uninstall", "TestResult", "SetLightCur", "CheckVoltage", "ShowTripTime"]
            n434 = event-data() -> ()  [unwired: 1 in, 1 out]
          }
          event "Set": Value Change {
            w618 = T16[] [enum."Clear", enum."Procedure"] items=["Initial_Data", "Initial_HMI", "Language", "UI", "Login", "Authority", "Clear", "Initial Test Data", "Initial Test Data1", "Initial Test UI", "Test Parameter", "PowerRemote", "PowerON", "PowerCalibration", "PowerOFF", "Temperature", "TempOffset", "Trip", "ShowInfo", "Finish?", "Period?", "LoopCurrent", "Procedure", "KGR", "Passed", "Failed", "MLFB Decoding", "MLFB Test Info", "MLFB Edit Info", "MLFB Edit", "MLFB Insert", "MLFB Delete", "ReportGeneralInfo", "ReportResultInfo", "ReportPath", "Generate Report", "Print Report", "New User", "Edit User", "Delete User", "Read User", "Voltage", "Time", "Current Calibration", "ErrorHandle", "StartTest", "ActiveLightCur", "Uninstall Record", "Get Uninstall Count", "Abort Test", "Test Model?", "CheckLoopCurrent", "Release HW Source", "Exit", "Close DB Connection", "Test UI BTN Status", "unTest UI BTN Status", "Disable All BTN", "AbortCalibration", "TprCalibration", "ClearReportInfo", "Set Uninstall", "TestResult", "SetLightCur", "CheckVoltage", "ShowTripTime"]
            n435 = event-data() -> ()  [unwired: 1 in, 1 out]
            n436 = property on="txtID" class="Str"("DisabledEnum"=T18."Enabled" ("Disabled")) -> ()  [unwired: 2 in, 2 out]
          }
          event "exit": Value Change; Application Instance Close {
            w622 = T16[] [enum."Release HW Source", enum."Close DB Connection", enum."Exit", enum."Procedure"] items=["Initial_Data", "Initial_HMI", "Language", "UI", "Login", "Authority", "Clear", "Initial Test Data", "Initial Test Data1", "Initial Test UI", "Test Parameter", "PowerRemote", "PowerON", "PowerCalibration", "PowerOFF", "Temperature", "TempOffset", "Trip", "ShowInfo", "Finish?", "Period?", "LoopCurrent", "Procedure", "KGR", "Passed", "Failed", "MLFB Decoding", "MLFB Test Info", "MLFB Edit Info", "MLFB Edit", "MLFB Insert", "MLFB Delete", "ReportGeneralInfo", "ReportResultInfo", "ReportPath", "Generate Report", "Print Report", "New User", "Edit User", "Delete User", "Read User", "Voltage", "Time", "Current Calibration", "ErrorHandle", "StartTest", "ActiveLightCur", "Uninstall Record", "Get Uninstall Count", "Abort Test", "Test Model?", "CheckLoopCurrent", "Release HW Source", "Exit", "Close DB Connection", "Test UI BTN Status", "unTest UI BTN Status", "Disable All BTN", "AbortCalibration", "TprCalibration", "ClearReportInfo", "Set Uninstall", "TestResult", "SetLightCur", "CheckVoltage", "ShowTripTime"]
            n437 = event-data() -> ()  [unwired: 1 in, 1 out]
          }
          event "Ok_Edit": Value Change {
            n438 = event-data() -> ("NewVal"=w626:bool)  [unwired: 1 in]
            n439 = case shown="True" w626 {
              tunnel: [w631 w632] -> w627
              frame False {
                w631 = T16[] [enum."Procedure"] items=["Initial_Data", "Initial_HMI", "Language", "UI", "Login", "Authority", "Clear", "Initial Test Data", "Initial Test Data1", "Initial Test UI", "Test Parameter", "PowerRemote", "PowerON", "PowerCalibration", "PowerOFF", "Temperature", "TempOffset", "Trip", "ShowInfo", "Finish?", "Period?", "LoopCurrent", "Procedure", "KGR", "Passed", "Failed", "MLFB Decoding", "MLFB Test Info", "MLFB Edit Info", "MLFB Edit", "MLFB Insert", "MLFB Delete", "ReportGeneralInfo", "ReportResultInfo", "ReportPath", "Generate Report", "Print Report", "New User", "Edit User", "Delete User", "Read User", "Voltage", "Time", "Current Calibration", "ErrorHandle", "StartTest", "ActiveLightCur", "Uninstall Record", "Get Uninstall Count", "Abort Test", "Test Model?", "CheckLoopCurrent", "Release HW Source", "Exit", "Close DB Connection", "Test UI BTN Status", "unTest UI BTN Status", "Disable All BTN", "AbortCalibration", "TprCalibration", "ClearReportInfo", "Set Uninstall", "TestResult", "SetLightCur", "CheckVoltage", "ShowTripTime"]
              }
              frame True {
                w632 = T16[] [enum."MLFB Edit", enum."Procedure"] items=["Initial_Data", "Initial_HMI", "Language", "UI", "Login", "Authority", "Clear", "Initial Test Data", "Initial Test Data1", "Initial Test UI", "Test Parameter", "PowerRemote", "PowerON", "PowerCalibration", "PowerOFF", "Temperature", "TempOffset", "Trip", "ShowInfo", "Finish?", "Period?", "LoopCurrent", "Procedure", "KGR", "Passed", "Failed", "MLFB Decoding", "MLFB Test Info", "MLFB Edit Info", "MLFB Edit", "MLFB Insert", "MLFB Delete", "ReportGeneralInfo", "ReportResultInfo", "ReportPath", "Generate Report", "Print Report", "New User", "Edit User", "Delete User", "Read User", "Voltage", "Time", "Current Calibration", "ErrorHandle", "StartTest", "ActiveLightCur", "Uninstall Record", "Get Uninstall Count", "Abort Test", "Test Model?", "CheckLoopCurrent", "Release HW Source", "Exit", "Close DB Connection", "Test UI BTN Status", "unTest UI BTN Status", "Disable All BTN", "AbortCalibration", "TprCalibration", "ClearReportInfo", "Set Uninstall", "TestResult", "SetLightCur", "CheckVoltage", "ShowTripTime"]
              }
            }
          }
          event "MLFB E": Value Change {
            n440 = event-data() -> ("NewVal"=w635:string)  [unwired: 1 in]
            n441 = String Length(string=w635) -> (length=w639:i32)
            n442 = Equal?(x=w639, y=13) -> (x = y?=w637:bool)
            n443 = case shown="True" w637 {
              tunnel: [w643 w647] -> w636
              tunnel: [w642 w646] -> w634
              tunnel: w633 -> [w642 w644]
              frame False {
                w643 = T16[] [enum."Procedure"] items=["Initial_Data", "Initial_HMI", "Language", "UI", "Login", "Authority", "Clear", "Initial Test Data", "Initial Test Data1", "Initial Test UI", "Test Parameter", "PowerRemote", "PowerON", "PowerCalibration", "PowerOFF", "Temperature", "TempOffset", "Trip", "ShowInfo", "Finish?", "Period?", "LoopCurrent", "Procedure", "KGR", "Passed", "Failed", "MLFB Decoding", "MLFB Test Info", "MLFB Edit Info", "MLFB Edit", "MLFB Insert", "MLFB Delete", "ReportGeneralInfo", "ReportResultInfo", "ReportPath", "Generate Report", "Print Report", "New User", "Edit User", "Delete User", "Read User", "Voltage", "Time", "Current Calibration", "ErrorHandle", "StartTest", "ActiveLightCur", "Uninstall Record", "Get Uninstall Count", "Abort Test", "Test Model?", "CheckLoopCurrent", "Release HW Source", "Exit", "Close DB Connection", "Test UI BTN Status", "unTest UI BTN Status", "Disable All BTN", "AbortCalibration", "TprCalibration", "ClearReportInfo", "Set Uninstall", "TestResult", "SetLightCur", "CheckVoltage", "ShowTripTime"]
              }
              frame True {
                w647 = T16[] [enum."MLFB Decoding", enum."MLFB Edit Info", enum."Procedure"] items=["Initial_Data", "Initial_HMI", "Language", "UI", "Login", "Authority", "Clear", "Initial Test Data", "Initial Test Data1", "Initial Test UI", "Test Parameter", "PowerRemote", "PowerON", "PowerCalibration", "PowerOFF", "Temperature", "TempOffset", "Trip", "ShowInfo", "Finish?", "Period?", "LoopCurrent", "Procedure", "KGR", "Passed", "Failed", "MLFB Decoding", "MLFB Test Info", "MLFB Edit Info", "MLFB Edit", "MLFB Insert", "MLFB Delete", "ReportGeneralInfo", "ReportResultInfo", "ReportPath", "Generate Report", "Print Report", "New User", "Edit User", "Delete User", "Read User", "Voltage", "Time", "Current Calibration", "ErrorHandle", "StartTest", "ActiveLightCur", "Uninstall Record", "Get Uninstall Count", "Abort Test", "Test Model?", "CheckLoopCurrent", "Release HW Source", "Exit", "Close DB Connection", "Test UI BTN Status", "unTest UI BTN Status", "Disable All BTN", "AbortCalibration", "TprCalibration", "ClearReportInfo", "Set Uninstall", "TestResult", "SetLightCur", "CheckVoltage", "ShowTripTime"]
                n444 = local read "MLFB E"() -> (w645:string)
                n445 = Bundle By Name(cluster=w644, "parameter.MLFB Info.MLFB"=w645) -> (w646:T3)
              }
            }
          }
          event "Cancel_Edit": Value Change {
            w649 = T16[] [enum."Clear", enum."Procedure"] items=["Initial_Data", "Initial_HMI", "Language", "UI", "Login", "Authority", "Clear", "Initial Test Data", "Initial Test Data1", "Initial Test UI", "Test Parameter", "PowerRemote", "PowerON", "PowerCalibration", "PowerOFF", "Temperature", "TempOffset", "Trip", "ShowInfo", "Finish?", "Period?", "LoopCurrent", "Procedure", "KGR", "Passed", "Failed", "MLFB Decoding", "MLFB Test Info", "MLFB Edit Info", "MLFB Edit", "MLFB Insert", "MLFB Delete", "ReportGeneralInfo", "ReportResultInfo", "ReportPath", "Generate Report", "Print Report", "New User", "Edit User", "Delete User", "Read User", "Voltage", "Time", "Current Calibration", "ErrorHandle", "StartTest", "ActiveLightCur", "Uninstall Record", "Get Uninstall Count", "Abort Test", "Test Model?", "CheckLoopCurrent", "Release HW Source", "Exit", "Close DB Connection", "Test UI BTN Status", "unTest UI BTN Status", "Disable All BTN", "AbortCalibration", "TprCalibration", "ClearReportInfo", "Set Uninstall", "TestResult", "SetLightCur", "CheckVoltage", "ShowTripTime"]
            n446 = event-data() -> ()  [unwired: 1 in, 1 out]
          }
          event "Login": Value Change {
            w654 = T16[] [enum."Login", enum."Authority", enum."Procedure"] items=["Initial_Data", "Initial_HMI", "Language", "UI", "Login", "Authority", "Clear", "Initial Test Data", "Initial Test Data1", "Initial Test UI", "Test Parameter", "PowerRemote", "PowerON", "PowerCalibration", "PowerOFF", "Temperature", "TempOffset", "Trip", "ShowInfo", "Finish?", "Period?", "LoopCurrent", "Procedure", "KGR", "Passed", "Failed", "MLFB Decoding", "MLFB Test Info", "MLFB Edit Info", "MLFB Edit", "MLFB Insert", "MLFB Delete", "ReportGeneralInfo", "ReportResultInfo", "ReportPath", "Generate Report", "Print Report", "New User", "Edit User", "Delete User", "Read User", "Voltage", "Time", "Current Calibration", "ErrorHandle", "StartTest", "ActiveLightCur", "Uninstall Record", "Get Uninstall Count", "Abort Test", "Test Model?", "CheckLoopCurrent", "Release HW Source", "Exit", "Close DB Connection", "Test UI BTN Status", "unTest UI BTN Status", "Disable All BTN", "AbortCalibration", "TprCalibration", "ClearReportInfo", "Set Uninstall", "TestResult", "SetLightCur", "CheckVoltage", "ShowTripTime"]
            n447 = event-data() -> ()  [unwired: 1 in, 1 out]
          }
          event "Logout": Value Change {
            w658 = T16[] [enum."Procedure"] items=["Initial_Data", "Initial_HMI", "Language", "UI", "Login", "Authority", "Clear", "Initial Test Data", "Initial Test Data1", "Initial Test UI", "Test Parameter", "PowerRemote", "PowerON", "PowerCalibration", "PowerOFF", "Temperature", "TempOffset", "Trip", "ShowInfo", "Finish?", "Period?", "LoopCurrent", "Procedure", "KGR", "Passed", "Failed", "MLFB Decoding", "MLFB Test Info", "MLFB Edit Info", "MLFB Edit", "MLFB Insert", "MLFB Delete", "ReportGeneralInfo", "ReportResultInfo", "ReportPath", "Generate Report", "Print Report", "New User", "Edit User", "Delete User", "Read User", "Voltage", "Time", "Current Calibration", "ErrorHandle", "StartTest", "ActiveLightCur", "Uninstall Record", "Get Uninstall Count", "Abort Test", "Test Model?", "CheckLoopCurrent", "Release HW Source", "Exit", "Close DB Connection", "Test UI BTN Status", "unTest UI BTN Status", "Disable All BTN", "AbortCalibration", "TprCalibration", "ClearReportInfo", "Set Uninstall", "TestResult", "SetLightCur", "CheckVoltage", "ShowTripTime"]
            w657 = ""
            n448 = event-data() -> ()  [unwired: 1 in, 1 out]
            n449 = Bundle By Name(cluster=w661, "parameter.Authority"=u32 0) -> (w660:T3)
            n450 = local write "Password"(w657) -> ()
            n451 = local write "Operator"(w657) -> ()
            n452 = local write "UserID"(w657) -> ()
          }
          event Value Change {
            w664 = T16[] [enum."Language", enum."Procedure"] items=["Initial_Data", "Initial_HMI", "Language", "UI", "Login", "Authority", "Clear", "Initial Test Data", "Initial Test Data1", "Initial Test UI", "Test Parameter", "PowerRemote", "PowerON", "PowerCalibration", "PowerOFF", "Temperature", "TempOffset", "Trip", "ShowInfo", "Finish?", "Period?", "LoopCurrent", "Procedure", "KGR", "Passed", "Failed", "MLFB Decoding", "MLFB Test Info", "MLFB Edit Info", "MLFB Edit", "MLFB Insert", "MLFB Delete", "ReportGeneralInfo", "ReportResultInfo", "ReportPath", "Generate Report", "Print Report", "New User", "Edit User", "Delete User", "Read User", "Voltage", "Time", "Current Calibration", "ErrorHandle", "StartTest", "ActiveLightCur", "Uninstall Record", "Get Uninstall Count", "Abort Test", "Test Model?", "CheckLoopCurrent", "Release HW Source", "Exit", "Close DB Connection", "Test UI BTN Status", "unTest UI BTN Status", "Disable All BTN", "AbortCalibration", "TprCalibration", "ClearReportInfo", "Set Uninstall", "TestResult", "SetLightCur", "CheckVoltage", "ShowTripTime"]
            n453 = event-data() -> ()  [unwired: 1 in, 1 out]
          }
          event "Report": Value Change {
            n454 = event-data() -> ("NewVal"=w667:bool)  [unwired: 1 in]
            n455 = case shown="True" w667 {
              tunnel: [w672 w673] -> w668
              frame False {
                w672 = T16[] [enum."Procedure"] items=["Initial_Data", "Initial_HMI", "Language", "UI", "Login", "Authority", "Clear", "Initial Test Data", "Initial Test Data1", "Initial Test UI", "Test Parameter", "PowerRemote", "PowerON", "PowerCalibration", "PowerOFF", "Temperature", "TempOffset", "Trip", "ShowInfo", "Finish?", "Period?", "LoopCurrent", "Procedure", "KGR", "Passed", "Failed", "MLFB Decoding", "MLFB Test Info", "MLFB Edit Info", "MLFB Edit", "MLFB Insert", "MLFB Delete", "ReportGeneralInfo", "ReportResultInfo", "ReportPath", "Generate Report", "Print Report", "New User", "Edit User", "Delete User", "Read User", "Voltage", "Time", "Current Calibration", "ErrorHandle", "StartTest", "ActiveLightCur", "Uninstall Record", "Get Uninstall Count", "Abort Test", "Test Model?", "CheckLoopCurrent", "Release HW Source", "Exit", "Close DB Connection", "Test UI BTN Status", "unTest UI BTN Status", "Disable All BTN", "AbortCalibration", "TprCalibration", "ClearReportInfo", "Set Uninstall", "TestResult", "SetLightCur", "CheckVoltage", "ShowTripTime"]
              }
              frame True {
                w673 = T16[] [enum."ReportPath", enum."Generate Report", enum."ClearReportInfo", enum."Print Report", enum."Procedure"] items=["Initial_Data", "Initial_HMI", "Language", "UI", "Login", "Authority", "Clear", "Initial Test Data", "Initial Test Data1", "Initial Test UI", "Test Parameter", "PowerRemote", "PowerON", "PowerCalibration", "PowerOFF", "Temperature", "TempOffset", "Trip", "ShowInfo", "Finish?", "Period?", "LoopCurrent", "Procedure", "KGR", "Passed", "Failed", "MLFB Decoding", "MLFB Test Info", "MLFB Edit Info", "MLFB Edit", "MLFB Insert", "MLFB Delete", "ReportGeneralInfo", "ReportResultInfo", "ReportPath", "Generate Report", "Print Report", "New User", "Edit User", "Delete User", "Read User", "Voltage", "Time", "Current Calibration", "ErrorHandle", "StartTest", "ActiveLightCur", "Uninstall Record", "Get Uninstall Count", "Abort Test", "Test Model?", "CheckLoopCurrent", "Release HW Source", "Exit", "Close DB Connection", "Test UI BTN Status", "unTest UI BTN Status", "Disable All BTN", "AbortCalibration", "TprCalibration", "ClearReportInfo", "Set Uninstall", "TestResult", "SetLightCur", "CheckVoltage", "ShowTripTime"]
              }
            }
          }
          event "btnCalibration": Value Change {
            w674 = T16[] [enum."PowerRemote", enum."PowerCalibration", enum."Procedure"] items=["Initial_Data", "Initial_HMI", "Language", "UI", "Login", "Authority", "Clear", "Initial Test Data", "Initial Test Data1", "Initial Test UI", "Test Parameter", "PowerRemote", "PowerON", "PowerCalibration", "PowerOFF", "Temperature", "TempOffset", "Trip", "ShowInfo", "Finish?", "Period?", "LoopCurrent", "Procedure", "KGR", "Passed", "Failed", "MLFB Decoding", "MLFB Test Info", "MLFB Edit Info", "MLFB Edit", "MLFB Insert", "MLFB Delete", "ReportGeneralInfo", "ReportResultInfo", "ReportPath", "Generate Report", "Print Report", "New User", "Edit User", "Delete User", "Read User", "Voltage", "Time", "Current Calibration", "ErrorHandle", "StartTest", "ActiveLightCur", "Uninstall Record", "Get Uninstall Count", "Abort Test", "Test Model?", "CheckLoopCurrent", "Release HW Source", "Exit", "Close DB Connection", "Test UI BTN Status", "unTest UI BTN Status", "Disable All BTN", "AbortCalibration", "TprCalibration", "ClearReportInfo", "Set Uninstall", "TestResult", "SetLightCur", "CheckVoltage", "ShowTripTime"]
            n456 = event-data() -> ()  [unwired: 1 in, 1 out]
          }
          event "abortCalibra": Value Change {
            w678 = T16[] [enum."PowerOFF", enum."AbortCalibration", enum."Procedure"] items=["Initial_Data", "Initial_HMI", "Language", "UI", "Login", "Authority", "Clear", "Initial Test Data", "Initial Test Data1", "Initial Test UI", "Test Parameter", "PowerRemote", "PowerON", "PowerCalibration", "PowerOFF", "Temperature", "TempOffset", "Trip", "ShowInfo", "Finish?", "Period?", "LoopCurrent", "Procedure", "KGR", "Passed", "Failed", "MLFB Decoding", "MLFB Test Info", "MLFB Edit Info", "MLFB Edit", "MLFB Insert", "MLFB Delete", "ReportGeneralInfo", "ReportResultInfo", "ReportPath", "Generate Report", "Print Report", "New User", "Edit User", "Delete User", "Read User", "Voltage", "Time", "Current Calibration", "ErrorHandle", "StartTest", "ActiveLightCur", "Uninstall Record", "Get Uninstall Count", "Abort Test", "Test Model?", "CheckLoopCurrent", "Release HW Source", "Exit", "Close DB Connection", "Test UI BTN Status", "unTest UI BTN Status", "Disable All BTN", "AbortCalibration", "TprCalibration", "ClearReportInfo", "Set Uninstall", "TestResult", "SetLightCur", "CheckVoltage", "ShowTripTime"]
            n457 = event-data() -> ()  [unwired: 1 in, 1 out]
          }
          event "btnReturn": Value Change {
            w683 = T16[] [enum."Clear", enum."Procedure"] items=["Initial_Data", "Initial_HMI", "Language", "UI", "Login", "Authority", "Clear", "Initial Test Data", "Initial Test Data1", "Initial Test UI", "Test Parameter", "PowerRemote", "PowerON", "PowerCalibration", "PowerOFF", "Temperature", "TempOffset", "Trip", "ShowInfo", "Finish?", "Period?", "LoopCurrent", "Procedure", "KGR", "Passed", "Failed", "MLFB Decoding", "MLFB Test Info", "MLFB Edit Info", "MLFB Edit", "MLFB Insert", "MLFB Delete", "ReportGeneralInfo", "ReportResultInfo", "ReportPath", "Generate Report", "Print Report", "New User", "Edit User", "Delete User", "Read User", "Voltage", "Time", "Current Calibration", "ErrorHandle", "StartTest", "ActiveLightCur", "Uninstall Record", "Get Uninstall Count", "Abort Test", "Test Model?", "CheckLoopCurrent", "Release HW Source", "Exit", "Close DB Connection", "Test UI BTN Status", "unTest UI BTN Status", "Disable All BTN", "AbortCalibration", "TprCalibration", "ClearReportInfo", "Set Uninstall", "TestResult", "SetLightCur", "CheckVoltage", "ShowTripTime"]
            n458 = event-data() -> ()  [unwired: 1 in, 1 out]
          }
          event "btnNewUser": Value Change {
            w688 = T16[] [enum."New User", enum."Procedure"] items=["Initial_Data", "Initial_HMI", "Language", "UI", "Login", "Authority", "Clear", "Initial Test Data", "Initial Test Data1", "Initial Test UI", "Test Parameter", "PowerRemote", "PowerON", "PowerCalibration", "PowerOFF", "Temperature", "TempOffset", "Trip", "ShowInfo", "Finish?", "Period?", "LoopCurrent", "Procedure", "KGR", "Passed", "Failed", "MLFB Decoding", "MLFB Test Info", "MLFB Edit Info", "MLFB Edit", "MLFB Insert", "MLFB Delete", "ReportGeneralInfo", "ReportResultInfo", "ReportPath", "Generate Report", "Print Report", "New User", "Edit User", "Delete User", "Read User", "Voltage", "Time", "Current Calibration", "ErrorHandle", "StartTest", "ActiveLightCur", "Uninstall Record", "Get Uninstall Count", "Abort Test", "Test Model?", "CheckLoopCurrent", "Release HW Source", "Exit", "Close DB Connection", "Test UI BTN Status", "unTest UI BTN Status", "Disable All BTN", "AbortCalibration", "TprCalibration", "ClearReportInfo", "Set Uninstall", "TestResult", "SetLightCur", "CheckVoltage", "ShowTripTime"]
            n459 = event-data() -> ()  [unwired: 1 in, 1 out]
            n460 = property on="txtPassword" class="Str"("Display Style"=u32 0) -> ()  [unwired: 2 in, 2 out]
          }
          event "btnReadUser": Value Change {
            n461 = event-data() -> ("NewVal"=w691:bool)  [unwired: 1 in]
            n462 = case shown="True" w691 {
              tunnel: [w696 w697] -> w692
              frame False {
                w696 = T16[] [enum."Procedure"] items=["Initial_Data", "Initial_HMI", "Language", "UI", "Login", "Authority", "Clear", "Initial Test Data", "Initial Test Data1", "Initial Test UI", "Test Parameter", "PowerRemote", "PowerON", "PowerCalibration", "PowerOFF", "Temperature", "TempOffset", "Trip", "ShowInfo", "Finish?", "Period?", "LoopCurrent", "Procedure", "KGR", "Passed", "Failed", "MLFB Decoding", "MLFB Test Info", "MLFB Edit Info", "MLFB Edit", "MLFB Insert", "MLFB Delete", "ReportGeneralInfo", "ReportResultInfo", "ReportPath", "Generate Report", "Print Report", "New User", "Edit User", "Delete User", "Read User", "Voltage", "Time", "Current Calibration", "ErrorHandle", "StartTest", "ActiveLightCur", "Uninstall Record", "Get Uninstall Count", "Abort Test", "Test Model?", "CheckLoopCurrent", "Release HW Source", "Exit", "Close DB Connection", "Test UI BTN Status", "unTest UI BTN Status", "Disable All BTN", "AbortCalibration", "TprCalibration", "ClearReportInfo", "Set Uninstall", "TestResult", "SetLightCur", "CheckVoltage", "ShowTripTime"]
              }
              frame True {
                w697 = T16[] [enum."Read User", enum."Procedure"] items=["Initial_Data", "Initial_HMI", "Language", "UI", "Login", "Authority", "Clear", "Initial Test Data", "Initial Test Data1", "Initial Test UI", "Test Parameter", "PowerRemote", "PowerON", "PowerCalibration", "PowerOFF", "Temperature", "TempOffset", "Trip", "ShowInfo", "Finish?", "Period?", "LoopCurrent", "Procedure", "KGR", "Passed", "Failed", "MLFB Decoding", "MLFB Test Info", "MLFB Edit Info", "MLFB Edit", "MLFB Insert", "MLFB Delete", "ReportGeneralInfo", "ReportResultInfo", "ReportPath", "Generate Report", "Print Report", "New User", "Edit User", "Delete User", "Read User", "Voltage", "Time", "Current Calibration", "ErrorHandle", "StartTest", "ActiveLightCur", "Uninstall Record", "Get Uninstall Count", "Abort Test", "Test Model?", "CheckLoopCurrent", "Release HW Source", "Exit", "Close DB Connection", "Test UI BTN Status", "unTest UI BTN Status", "Disable All BTN", "AbortCalibration", "TprCalibration", "ClearReportInfo", "Set Uninstall", "TestResult", "SetLightCur", "CheckVoltage", "ShowTripTime"]
              }
            }
          }
          event "btnEditUser": Value Change {
            n463 = event-data() -> ("NewVal"=w698:bool)  [unwired: 1 in]
            n464 = case shown="False" w698 {
              tunnel: [w703 w704] -> w699
              frame False {
                w703 = T16[] [enum."Procedure"] items=["Initial_Data", "Initial_HMI", "Language", "UI", "Login", "Authority", "Clear", "Initial Test Data", "Initial Test Data1", "Initial Test UI", "Test Parameter", "PowerRemote", "PowerON", "PowerCalibration", "PowerOFF", "Temperature", "TempOffset", "Trip", "ShowInfo", "Finish?", "Period?", "LoopCurrent", "Procedure", "KGR", "Passed", "Failed", "MLFB Decoding", "MLFB Test Info", "MLFB Edit Info", "MLFB Edit", "MLFB Insert", "MLFB Delete", "ReportGeneralInfo", "ReportResultInfo", "ReportPath", "Generate Report", "Print Report", "New User", "Edit User", "Delete User", "Read User", "Voltage", "Time", "Current Calibration", "ErrorHandle", "StartTest", "ActiveLightCur", "Uninstall Record", "Get Uninstall Count", "Abort Test", "Test Model?", "CheckLoopCurrent", "Release HW Source", "Exit", "Close DB Connection", "Test UI BTN Status", "unTest UI BTN Status", "Disable All BTN", "AbortCalibration", "TprCalibration", "ClearReportInfo", "Set Uninstall", "TestResult", "SetLightCur", "CheckVoltage", "ShowTripTime"]
              }
              frame True {
                w704 = T16[] [enum."Edit User", enum."Procedure"] items=["Initial_Data", "Initial_HMI", "Language", "UI", "Login", "Authority", "Clear", "Initial Test Data", "Initial Test Data1", "Initial Test UI", "Test Parameter", "PowerRemote", "PowerON", "PowerCalibration", "PowerOFF", "Temperature", "TempOffset", "Trip", "ShowInfo", "Finish?", "Period?", "LoopCurrent", "Procedure", "KGR", "Passed", "Failed", "MLFB Decoding", "MLFB Test Info", "MLFB Edit Info", "MLFB Edit", "MLFB Insert", "MLFB Delete", "ReportGeneralInfo", "ReportResultInfo", "ReportPath", "Generate Report", "Print Report", "New User", "Edit User", "Delete User", "Read User", "Voltage", "Time", "Current Calibration", "ErrorHandle", "StartTest", "ActiveLightCur", "Uninstall Record", "Get Uninstall Count", "Abort Test", "Test Model?", "CheckLoopCurrent", "Release HW Source", "Exit", "Close DB Connection", "Test UI BTN Status", "unTest UI BTN Status", "Disable All BTN", "AbortCalibration", "TprCalibration", "ClearReportInfo", "Set Uninstall", "TestResult", "SetLightCur", "CheckVoltage", "ShowTripTime"]
              }
            }
          }
          event "btnDeleteUser": Value Change {
            w705 = T16[] [enum."Delete User", enum."Procedure"] items=["Initial_Data", "Initial_HMI", "Language", "UI", "Login", "Authority", "Clear", "Initial Test Data", "Initial Test Data1", "Initial Test UI", "Test Parameter", "PowerRemote", "PowerON", "PowerCalibration", "PowerOFF", "Temperature", "TempOffset", "Trip", "ShowInfo", "Finish?", "Period?", "LoopCurrent", "Procedure", "KGR", "Passed", "Failed", "MLFB Decoding", "MLFB Test Info", "MLFB Edit Info", "MLFB Edit", "MLFB Insert", "MLFB Delete", "ReportGeneralInfo", "ReportResultInfo", "ReportPath", "Generate Report", "Print Report", "New User", "Edit User", "Delete User", "Read User", "Voltage", "Time", "Current Calibration", "ErrorHandle", "StartTest", "ActiveLightCur", "Uninstall Record", "Get Uninstall Count", "Abort Test", "Test Model?", "CheckLoopCurrent", "Release HW Source", "Exit", "Close DB Connection", "Test UI BTN Status", "unTest UI BTN Status", "Disable All BTN", "AbortCalibration", "TprCalibration", "ClearReportInfo", "Set Uninstall", "TestResult", "SetLightCur", "CheckVoltage", "ShowTripTime"]
            n465 = event-data() -> ()  [unwired: 1 in, 1 out]
          }
          event "btnDelete": Value Change {
            n466 = event-data() -> ("NewVal"=w709:bool)  [unwired: 1 in]
            n467 = case shown="True" w709 {
              tunnel: [w714 w715] -> w710
              frame False {
                w714 = T16[] [enum."Procedure"] items=["Initial_Data", "Initial_HMI", "Language", "UI", "Login", "Authority", "Clear", "Initial Test Data", "Initial Test Data1", "Initial Test UI", "Test Parameter", "PowerRemote", "PowerON", "PowerCalibration", "PowerOFF", "Temperature", "TempOffset", "Trip", "ShowInfo", "Finish?", "Period?", "LoopCurrent", "Procedure", "KGR", "Passed", "Failed", "MLFB Decoding", "MLFB Test Info", "MLFB Edit Info", "MLFB Edit", "MLFB Insert", "MLFB Delete", "ReportGeneralInfo", "ReportResultInfo", "ReportPath", "Generate Report", "Print Report", "New User", "Edit User", "Delete User", "Read User", "Voltage", "Time", "Current Calibration", "ErrorHandle", "StartTest", "ActiveLightCur", "Uninstall Record", "Get Uninstall Count", "Abort Test", "Test Model?", "CheckLoopCurrent", "Release HW Source", "Exit", "Close DB Connection", "Test UI BTN Status", "unTest UI BTN Status", "Disable All BTN", "AbortCalibration", "TprCalibration", "ClearReportInfo", "Set Uninstall", "TestResult", "SetLightCur", "CheckVoltage", "ShowTripTime"]
              }
              frame True {
                w715 = T16[] [enum."MLFB Delete", enum."Clear", enum."Procedure"] items=["Initial_Data", "Initial_HMI", "Language", "UI", "Login", "Authority", "Clear", "Initial Test Data", "Initial Test Data1", "Initial Test UI", "Test Parameter", "PowerRemote", "PowerON", "PowerCalibration", "PowerOFF", "Temperature", "TempOffset", "Trip", "ShowInfo", "Finish?", "Period?", "LoopCurrent", "Procedure", "KGR", "Passed", "Failed", "MLFB Decoding", "MLFB Test Info", "MLFB Edit Info", "MLFB Edit", "MLFB Insert", "MLFB Delete", "ReportGeneralInfo", "ReportResultInfo", "ReportPath", "Generate Report", "Print Report", "New User", "Edit User", "Delete User", "Read User", "Voltage", "Time", "Current Calibration", "ErrorHandle", "StartTest", "ActiveLightCur", "Uninstall Record", "Get Uninstall Count", "Abort Test", "Test Model?", "CheckLoopCurrent", "Release HW Source", "Exit", "Close DB Connection", "Test UI BTN Status", "unTest UI BTN Status", "Disable All BTN", "AbortCalibration", "TprCalibration", "ClearReportInfo", "Set Uninstall", "TestResult", "SetLightCur", "CheckVoltage", "ShowTripTime"]
              }
            }
          }
          event "readCalibra": Value Change {
            w716 = T16[] [enum."Current Calibration", enum."Procedure"] items=["Initial_Data", "Initial_HMI", "Language", "UI", "Login", "Authority", "Clear", "Initial Test Data", "Initial Test Data1", "Initial Test UI", "Test Parameter", "PowerRemote", "PowerON", "PowerCalibration", "PowerOFF", "Temperature", "TempOffset", "Trip", "ShowInfo", "Finish?", "Period?", "LoopCurrent", "Procedure", "KGR", "Passed", "Failed", "MLFB Decoding", "MLFB Test Info", "MLFB Edit Info", "MLFB Edit", "MLFB Insert", "MLFB Delete", "ReportGeneralInfo", "ReportResultInfo", "ReportPath", "Generate Report", "Print Report", "New User", "Edit User", "Delete User", "Read User", "Voltage", "Time", "Current Calibration", "ErrorHandle", "StartTest", "ActiveLightCur", "Uninstall Record", "Get Uninstall Count", "Abort Test", "Test Model?", "CheckLoopCurrent", "Release HW Source", "Exit", "Close DB Connection", "Test UI BTN Status", "unTest UI BTN Status", "Disable All BTN", "AbortCalibration", "TprCalibration", "ClearReportInfo", "Set Uninstall", "TestResult", "SetLightCur", "CheckVoltage", "ShowTripTime"]
            n468 = event-data() -> ()  [unwired: 1 in, 1 out]
          }
          event "btnCalTpr": Value Change {
            w720 = T16[] [enum."TprCalibration", enum."Procedure"] items=["Initial_Data", "Initial_HMI", "Language", "UI", "Login", "Authority", "Clear", "Initial Test Data", "Initial Test Data1", "Initial Test UI", "Test Parameter", "PowerRemote", "PowerON", "PowerCalibration", "PowerOFF", "Temperature", "TempOffset", "Trip", "ShowInfo", "Finish?", "Period?", "LoopCurrent", "Procedure", "KGR", "Passed", "Failed", "MLFB Decoding", "MLFB Test Info", "MLFB Edit Info", "MLFB Edit", "MLFB Insert", "MLFB Delete", "ReportGeneralInfo", "ReportResultInfo", "ReportPath", "Generate Report", "Print Report", "New User", "Edit User", "Delete User", "Read User", "Voltage", "Time", "Current Calibration", "ErrorHandle", "StartTest", "ActiveLightCur", "Uninstall Record", "Get Uninstall Count", "Abort Test", "Test Model?", "CheckLoopCurrent", "Release HW Source", "Exit", "Close DB Connection", "Test UI BTN Status", "unTest UI BTN Status", "Disable All BTN", "AbortCalibration", "TprCalibration", "ClearReportInfo", "Set Uninstall", "TestResult", "SetLightCur", "CheckVoltage", "ShowTripTime"]
            n469 = event-data() -> ()  [unwired: 1 in, 1 out]
          }
          event "btnReadLCConfig": Value Change {
            w729 = T16[] [enum."Procedure"] items=["Initial_Data", "Initial_HMI", "Language", "UI", "Login", "Authority", "Clear", "Initial Test Data", "Initial Test Data1", "Initial Test UI", "Test Parameter", "PowerRemote", "PowerON", "PowerCalibration", "PowerOFF", "Temperature", "TempOffset", "Trip", "ShowInfo", "Finish?", "Period?", "LoopCurrent", "Procedure", "KGR", "Passed", "Failed", "MLFB Decoding", "MLFB Test Info", "MLFB Edit Info", "MLFB Edit", "MLFB Insert", "MLFB Delete", "ReportGeneralInfo", "ReportResultInfo", "ReportPath", "Generate Report", "Print Report", "New User", "Edit User", "Delete User", "Read User", "Voltage", "Time", "Current Calibration", "ErrorHandle", "StartTest", "ActiveLightCur", "Uninstall Record", "Get Uninstall Count", "Abort Test", "Test Model?", "CheckLoopCurrent", "Release HW Source", "Exit", "Close DB Connection", "Test UI BTN Status", "unTest UI BTN Status", "Disable All BTN", "AbortCalibration", "TprCalibration", "ClearReportInfo", "Set Uninstall", "TestResult", "SetLightCur", "CheckVoltage", "ShowTripTime"]
            n470 = event-data() -> ()  [unwired: 1 in, 1 out]
            n471 = Unbundle By Name(w728) -> ("DelayByUser"=w727:dbl, "DelayInCase"=w725:dbl)
            n472 = Number To Decimal String(number=w725) -> (decimal integer string=w724:string)  [unwired: 1 in]
            n473 = Number To Decimal String(number=w727) -> (decimal integer string=w726:string)  [unwired: 1 in]
            n474 = local write "DelayByUser"(w726) -> ()
            n475 = local write "DelayToFailed"(w724) -> ()
          }
          event "btnEditLCConfig": Value Change {
            w739 = T16[] [enum."Procedure"] items=["Initial_Data", "Initial_HMI", "Language", "UI", "Login", "Authority", "Clear", "Initial Test Data", "Initial Test Data1", "Initial Test UI", "Test Parameter", "PowerRemote", "PowerON", "PowerCalibration", "PowerOFF", "Temperature", "TempOffset", "Trip", "ShowInfo", "Finish?", "Period?", "LoopCurrent", "Procedure", "KGR", "Passed", "Failed", "MLFB Decoding", "MLFB Test Info", "MLFB Edit Info", "MLFB Edit", "MLFB Insert", "MLFB Delete", "ReportGeneralInfo", "ReportResultInfo", "ReportPath", "Generate Report", "Print Report", "New User", "Edit User", "Delete User", "Read User", "Voltage", "Time", "Current Calibration", "ErrorHandle", "StartTest", "ActiveLightCur", "Uninstall Record", "Get Uninstall Count", "Abort Test", "Test Model?", "CheckLoopCurrent", "Release HW Source", "Exit", "Close DB Connection", "Test UI BTN Status", "unTest UI BTN Status", "Disable All BTN", "AbortCalibration", "TprCalibration", "ClearReportInfo", "Set Uninstall", "TestResult", "SetLightCur", "CheckVoltage", "ShowTripTime"]
            n476 = event-data() -> ()  [unwired: 1 in, 1 out]
            n477 = Build Array("DelayByUser", "DelayToFailed") -> (w734:string[])
            n478 = call "WriteConfig.vi"("error in"=w732, "Value"=w734, "section"="[DelayofLightCurtain]") -> ("error out"=w733:errorcluster)  [unwired: 2 in]
          }
        }
      }
      frame "Login" {
        n479 = Unbundle By Name(w749) -> ("parameter.MLFB"=w752:T9)
        n480 = call "Database_User_Read.vi"("error in"=w753, "Language"=w751, "ID_Number"="UserID", "connection reference"=w752) -> ("error out"=w743:errorcluster, "Ok?"=w746:bool, "Message"=w756:string, "UserRight"=w755:T20)  [unwired: 4 in]
        n481 = case shown="True" w746 {
          tunnel: w756 -> [w760 _]
          tunnel: w755 -> [_ w776]
          tunnel: [w758 w774] -> w750
          tunnel: [_ w770] -> w747
          tunnel: [2 ("Authority") w769] -> w748
          tunnel: w751 -> [_ w768]
          tunnel: w745 -> [w758 w765]
          tunnel: w742 -> [w757 w764]
          tunnel: [w757 w763] -> w741
          frame False {
            n482 = stacked-sequence {
              tunnel: w760 -> [w761 _]
              frame #0 {
                n483 = One Button Dialog(message=w761) -> ()  [unwired: 1 in, 1 out]
              }
              frame #1 {
                n484 = local write "UserID"("" ("UserID")) -> ()
              }
            }
          }
          frame True {
            n485 = Unbundle By Name(w776) -> ("Password"=w773:string, "Authority"=w772:i32, "Name"=w771:string)
            n486 = call <vilib>:"Trim Whitespace.vi"("string"="Password") -> ("trimmed string"=w766:string)  [unwired: 1 in]
            n487 = Equal?(x=w766, y=w773) -> (x = y?=w775:bool)
            n488 = case shown="True" w775 {
              tunnel: [w778 T10."Test" ("Tab")] -> w774
              tunnel: w772 -> [_ w787]
              tunnel: [_ w788] -> w770
              tunnel: w771 -> [_ w788]
              tunnel: [2 ("Authority") w787] -> w769
              tunnel: w768 -> [w781 _]
              tunnel: w765 -> [w778 _]
              tunnel: w764 -> [w777 w786]
              tunnel: [w777 w786] -> w763
              frame False {
                n489 = case shown="\"中文\"" w781 {
                  tunnel: ["Password Error" "密码错误"] -> w779
                  frame "English" {
                  }
                  frame "中文" {
                  }
                }
                n490 = stacked-sequence {
                  tunnel: w779 -> [w782 _]
                  frame #0 {
                    n491 = One Button Dialog(message=w782) -> ()  [unwired: 1 in, 1 out]
                  }
                  frame #1 {
                    n492 = local write "Password"("" ("Password")) -> ()
                  }
                }
              }
              frame True {
              }
            }
          }
        }
        "Operator" <- w747
        n493 = Bundle By Name(cluster=w749, "parameter.Authority"=w748) -> (w744:T3)
      }
      frame "Authority" {
        n494 = Unbundle By Name(w792) -> ("parameter.Authority"=w791:u32)
        n495 = case shown="0, Default" w791 {
          frame 0, Default {
            w795 = T18."Enabled" ("Disabled")
            w796 = T18."Disabled and Grayed Out" ("Disabled")
            # "worker"
            n496 = property on="New" class="Bool"("DisabledEnum"=w796) -> ()  [unwired: 2 in, 2 out]
            n497 = property on="Edit" class="Bool"("DisabledEnum"=w796) -> ()  [unwired: 2 in, 2 out]
            n498 = property on="Set" class="Bool"("DisabledEnum"=w796) -> ()  [unwired: 2 in, 2 out]
            n499 = property on="btnAbort" class="Bool (strict)"("DisabledEnum"=w796) -> ()  [unwired: 2 in, 2 out]
            n500 = property on="Start" class="Bool"("DisabledEnum"=w795) -> ()  [unwired: 2 in, 2 out]
            n501 = property on="exit" class="Bool"("DisabledEnum"=w795) -> ()  [unwired: 2 in, 2 out]
          }
          frame 1 {
            w797 = T18."Enabled" ("Disabled")
            # "engineer"
            n502 = property on="Start" class="Bool"("DisabledEnum"=w797) -> ()  [unwired: 2 in, 2 out]
            n503 = property on="Set" class="Bool"("DisabledEnum"=w797) -> ()  [unwired: 2 in, 2 out]
            n504 = property on="New" class="Bool"("DisabledEnum"=w797) -> ()  [unwired: 2 in, 2 out]
            n505 = property on="Edit" class="Bool"("DisabledEnum"=w797) -> ()  [unwired: 2 in, 2 out]
            n506 = property on="exit" class="Bool"("DisabledEnum"=w797) -> ()  [unwired: 2 in, 2 out]
            n507 = property on="btnAbort" class="Bool (strict)"("DisabledEnum"=T18."Disabled and Grayed Out" ("Disabled")) -> ()  [unwired: 2 in, 2 out]
          }
        }
      }
      frame "Clear" {
        n508 = stacked-sequence {
          tunnel: w800 -> [_ _ _ _ w835]
          tunnel: [_ _ _ _ w835] -> w799
          frame #0 {
            w804 = 0.0 ("KG20_IL N")
            w805 = 0 ("consTime_IL")
            w807 = "" ("MLFB_show")
            w806 = "" ("Torque N")
            w809 = "" ("MLFB")
            w808 = "" ("MLFB_show")
            n509 = property on="MLFB_show" class="Str"("Value"=w808) -> ()  [unwired: 2 in, 2 out]
            n510 = property on="orderNum_M" class="Str"("Value"=w808) -> ()  [unwired: 2 in, 2 out]
            n511 = property on="process" class="Str"("Value"=w808) -> ()  [unwired: 2 in, 2 out]
            n512 = property on="remaing" class="Str"("Value"=w808) -> ()  [unwired: 2 in, 2 out]
            n513 = property on="Total" class="Str"("Value"=w808) -> ()  [unwired: 2 in, 2 out]
            n514 = property on="StartTime" class="Str"("Value"=w807) -> ()  [unwired: 2 in, 2 out]
            n515 = property on="AccelerationTime" class="Str"("Value"=w807) -> ()  [unwired: 2 in, 2 out]
            n516 = property on="Torque" class="Str"("Value"=w807) -> ()  [unwired: 2 in, 2 out]
            n517 = property on="Frame N" class="Str"("Value"=w807) -> ()  [unwired: 2 in, 2 out]
            n518 = property on="curRange N" class="Str"("Value"=w807) -> ()  [unwired: 2 in, 2 out]
            n519 = property on="MLFB" class="Str"("Value"=w809) -> ()  [unwired: 2 in, 2 out]
            n520 = property on="Operator_test" class="Str"("Value"=w809) -> ()  [unwired: 2 in, 2 out]
            n521 = property on="orderNum_P" class="Str"("Value"=w809) -> ()  [unwired: 2 in, 2 out]
            n522 = property on="orderCount" class="Str"("Value"=w809) -> ()  [unwired: 2 in, 2 out]
            n523 = property on="testCount" class="Str"("Value"=w809) -> ()  [unwired: 2 in, 2 out]
            n524 = property on="Torque N" class="Str"("Value"=w806) -> ()  [unwired: 2 in, 2 out]
            n525 = property on="MLFB N" class="Str"("Value"=w806) -> ()  [unwired: 2 in, 2 out]
            n526 = property on="Test Date" class="Str"("Value"=w806) -> ()  [unwired: 2 in, 2 out]
            n527 = property on="productCode" class="Str"("Value"=w806) -> ()  [unwired: 2 in, 2 out]
            n528 = property on="Frame" class="Str"("Value"=w806) -> ()  [unwired: 2 in, 2 out]
            n529 = property on="consTime_IL" class="DigNum (strict)"("Value"=w805) -> ()  [unwired: 2 in, 2 out]
            n530 = property on="Preload_Limit N" class="DigNum (strict)"("Value"=w805) -> ()  [unwired: 2 in, 2 out]
            n531 = property on="KG20_IL N" class="DigNum (strict)"("Value"=w804) -> ()  [unwired: 2 in, 2 out]
            n532 = property on="DA E" class="DigNum (strict)"("Value"=w804) -> ()  [unwired: 2 in, 2 out]
          }
          frame #1 {
            w810 = 0 ("preload_Limit")
            w811 = u8 0 ("pirntProcess")
            w812 = 0.0 ("Resistance N")
            w813 = 0.0 ("current")
            w814 = 0.0 ("current")
            n533 = property on="current" class="DigNum (strict)"("Value"=w814) -> ()  [unwired: 2 in, 2 out]
            n534 = property on="Current_IL" class="DigNum (strict)"("Value"=w814) -> ()  [unwired: 2 in, 2 out]
            n535 = property on="DA_IL" class="DigNum (strict)"("Value"=w814) -> ()  [unwired: 2 in, 2 out]
            n536 = property on="DA_uL" class="DigNum (strict)"("Value"=w814) -> ()  [unwired: 2 in, 2 out]
            n537 = property on="DA N" class="DigNum (strict)"("Value"=w814) -> ()  [unwired: 2 in, 2 out]
            n538 = property on="Gauge_In" class="DigNum (strict)"("Value"=w813) -> ()  [unwired: 2 in, 2 out]
            n539 = property on="Gauge_Out" class="DigNum (strict)"("Value"=w813) -> ()  [unwired: 2 in, 2 out]
            n540 = property on="Current_uL N" class="DigNum (strict)"("Value"=w813) -> ()  [unwired: 2 in, 2 out]
            n541 = property on="KG20_uL N" class="DigNum (strict)"("Value"=w813) -> ()  [unwired: 2 in, 2 out]
            n542 = property on="Gauge_Out N" class="DigNum (strict)"("Value"=w813) -> ()  [unwired: 2 in, 2 out]
            n543 = property on="Resistance N" class="DigNum (strict)"("Value"=w812) -> ()  [unwired: 2 in, 2 out]
            n544 = property on="thermoRs" class="DigNum (strict)"("Value"=w812) -> ()  [unwired: 2 in, 2 out]
            n545 = property on="releaseRs" class="DigNum (strict)"("Value"=w812) -> ()  [unwired: 2 in, 2 out]
            n546 = property on="Gauge_In N" class="DigNum (strict)"("Value"=w812) -> ()  [unwired: 2 in, 2 out]
            n547 = property on="KG20_IL" class="DigNum (strict)"("Value"=w812) -> ()  [unwired: 2 in, 2 out]
            n548 = property on="pirntProcess" class="Slide (strict)"("Value"=w811) -> ()  [unwired: 2 in, 2 out]
            n549 = property on="consTime_IL N" class="DigNum (strict)"("Value"=w811) -> ()  [unwired: 2 in, 2 out]
            n550 = property on="Load_Release N" class="DigNum (strict)"("Value"=w811) -> ()  [unwired: 2 in, 2 out]
            n551 = property on="Preload_Release N" class="DigNum (strict)"("Value"=w811) -> ()  [unwired: 2 in, 2 out]
            n552 = property on="Load_Limit N" class="DigNum (strict)"("Value"=w811) -> ()  [unwired: 2 in, 2 out]
            n553 = property on="preload_Limit" class="DigNum (strict)"("Value"=w810) -> ()  [unwired: 2 in, 2 out]
            n554 = property on="preload_Action" class="DigNum (strict)"("Value"=w810) -> ()  [unwired: 2 in, 2 out]
            n555 = property on="load_Limit" class="DigNum (strict)"("Value"=w810) -> ()  [unwired: 2 in, 2 out]
            n556 = property on="load_Action" class="DigNum (strict)"("Value"=w810) -> ()  [unwired: 2 in, 2 out]
            n557 = property on="consTime_uL N" class="DigNum (strict)"("Value"=w810) -> ()  [unwired: 2 in, 2 out]
          }
          frame #2 {
            w821 = FALSE ("Pass")
            w822 = 0 ("Preload_Action E")
            w823 = "" ("Torque E")
            w824 = "" ("Torque E")
            w825 = "" ("MLFB E")
            n558 = property on="MLFB E" class="Str"("Value"=w825) -> ()  [unwired: 2 in, 2 out]
            n559 = property on="Frame E" class="Str"("Value"=w825) -> ()  [unwired: 2 in, 2 out]
            n560 = property on="curRange E" class="Str"("Value"=w825) -> ()  [unwired: 2 in, 2 out]
            n561 = property on="EndTime" class="Str"("Value"=w825) -> ()  [unwired: 2 in, 2 out]
            n562 = property on="totalSec" class="Str"("Value"=w825) -> ()  [unwired: 2 in, 2 out]
            n563 = property on="Torque E" class="Str"("Value"=w824) -> ()  [unwired: 2 in, 2 out]
            n564 = property on="txtID" class="Str"("Value"=w824) -> ()  [unwired: 2 in, 2 out]
            n565 = property on="txtName" class="Str"("Value"=w824) -> ()  [unwired: 2 in, 2 out]
            n566 = property on="Temperature" class="Str"("Value"=w824) -> ()  [unwired: 2 in, 2 out]
            n567 = property on="ThermalTmFrame" class="Str"("Value"=w824) -> ()  [unwired: 2 in, 2 out]
            n568 = property on="Preload_Action E" class="DigNum (strict)"("Value"=w822) -> ()  [unwired: 2 in, 2 out]
            n569 = property on="Preload_Limit E" class="DigNum (strict)"("Value"=w822) -> ()  [unwired: 2 in, 2 out]
            n570 = property on="consTime_uL E" class="DigNum (strict)"("Value"=w822) -> ()  [unwired: 2 in, 2 out]
            n571 = property on="Load_Limit E" class="DigNum (strict)"("Value"=w822) -> ()  [unwired: 2 in, 2 out]
            n572 = property on="Load_Action E" class="DigNum (strict)"("Value"=w822) -> ()  [unwired: 2 in, 2 out]
            n573 = property on="consTime_IL E" class="DigNum (strict)"("Value"=0 ("consTime_IL E")) -> ()  [unwired: 2 in, 2 out]
            n574 = property on="totalHour" class="Str"("Value"=w823) -> ()  [unwired: 2 in, 2 out]
            n575 = property on="txtPassword" class="Str"("Value"=w823) -> ()  [unwired: 2 in, 2 out]
            n576 = property on="Pass" class="Bool (strict)"("Value"=w821) -> ()  [unwired: 2 in, 2 out]
            n577 = property on="Fail" class="Bool (strict)"("Value"=w821) -> ()  [unwired: 2 in, 2 out]
            n578 = property on="remaing" class="Str"("Caption.Text"="P1") -> ()  [unwired: 2 in, 2 out]
            n579 = local write "RunInfo"("" ("RunInfo")) -> ()
            n580 = local write "btnAbort"(FALSE ("btnAbort")) -> ()
            n581 = property on="consTime_uL" class="DigNum (strict)"("Value"=0 ("consTime_uL")) -> ()  [unwired: 2 in, 2 out]
            n582 = property on="Just Code" class="Clust (strict)"("Value"=T14 {"1"="", "2"="", "3"="", "4"="", "5"="", "6"="", "7"="", "8"="", "9"="", "10"="", "11"="", "12"="", "13"="", "14"="", "15"="", "16"="", "17"="", "18"="", "19"="", "20"=""} ("Just Code")) -> ()  [unwired: 2 in, 2 out]
          }
          frame #3 {
            w834 = 0.0 ("DA E")
            w833 = 0.0 ("Current_uL")
            w832 = 0.0 ("thermoRs E")
            n583 = property on="thermoRs E" class="DigNum (strict)"("Value"=w832) -> ()  [unwired: 2 in, 2 out]
            n584 = property on="Current_IL E" class="DigNum (strict)"("Value"=w832) -> ()  [unwired: 2 in, 2 out]
            n585 = property on="KG_uL E" class="DigNum (strict)"("Value"=w832) -> ()  [unwired: 2 in, 2 out]
            n586 = property on="KG_IL E" class="DigNum (strict)"("Value"=w832) -> ()  [unwired: 2 in, 2 out]
            n587 = property on="Current_uL E" class="DigNum (strict)"("Value"=w832) -> ()  [unwired: 2 in, 2 out]
            n588 = property on="releaseRs E" class="DigNum (strict)"("Value"=w833) -> ()  [unwired: 2 in, 2 out]
            n589 = property on="circuitRs E" class="DigNum (strict)"("Value"=w833) -> ()  [unwired: 2 in, 2 out]
            n590 = property on="Current_uL" class="DigNum (strict)"("Value"=w833) -> ()  [unwired: 2 in, 2 out]
            n591 = property on="KG20_uL" class="DigNum (strict)"("Value"=w833) -> ()  [unwired: 2 in, 2 out]
            n592 = property on="valueCalibra" class="DigNum (strict)"("Value"=w833) -> ()  [unwired: 2 in, 2 out]
            n593 = property on="setCalibra" class="DigNum (strict)"("Value"=w834) -> ()  [unwired: 2 in, 2 out]
            n594 = property on="Gauge_Out E" class="DigNum (strict)"("Value"=w834) -> ()  [unwired: 2 in, 2 out]
            n595 = property on="Gauge_In E" class="DigNum (strict)"("Value"=w834) -> ()  [unwired: 2 in, 2 out]
            n596 = property on="Current_IL N" class="DigNum (strict)"("Value"=w834) -> ()  [unwired: 2 in, 2 out]
            n597 = property on="vlCalTpr" class="DigNum (strict)"("Value"=w834) -> ()  [unwired: 2 in, 2 out]
            n598 = Array To Cluster(array=bool[] [TRUE, TRUE, TRUE, TRUE, TRUE, TRUE, TRUE, TRUE, TRUE, TRUE, TRUE, TRUE, TRUE, TRUE, TRUE, TRUE, TRUE, TRUE, TRUE, TRUE]) -> (cluster=w829:T22)
            n599 = local write "TestModel"(Model."lowLimit" ("TestModel")) -> ()
            n600 = local write "pirntProcess"(u8 0 ("pirntProcess")) -> ()
            n601 = local write "trippedStatus"(w829) -> ()
            n602 = property on="parameter" class="MCListbox (strict)"("ItemNames"=string[][] [["", "", "", ""], ["", "", "", ""], ["", "", "", ""], ["", "", "", ""]] ("Item Names")) -> ()  [unwired: 2 in, 2 out]
            n603 = property on="Authority" class="Enum (strict)"("Value"=enum16{"Operator", "Engineer"}."Operator") -> ()  [unwired: 2 in, 2 out]
          }
          frame #4 {
          }
        }
      }
      frame "Initial Test Data" {
        w846 = path "" ("parameter.path.template (empty)")
        w838 = dbl[] [] ("parameter.KG20")
        w837 = 0.0 ("parameter.mesCurrent")
        n604 = Bundle By Name(cluster=w848, "parameter.voltage"=dbl[] [0.0, 0.0, 0.0, 0.0, 0.0, 0.0, 0.0, 0.0, 0.0, 0.0, 0.0, 0.0, 0.0, 0.0, 0.0, 0.0, 0.0, 0.0, 0.0, 0.0], "parameter.mesCurrent"=w837, "parameter.testCurrent"=w837, "parameter.baseCurrent"=w837, "parameter.KG"=w837, "parameter.KG20"=w838, "parameter.KTu"=w838, "parameter.temperature"=w838, "parameter.path.template (empty)"=w846, "parameter.path.Report path"=w846, "parameter.path.Backup path"=w846, "parameter.UL?"=FALSE, "parameter.numTrip"=i32[] [0, 0, 0, 0], "parameter.Message"="", "parameter.Tripped Time"=i32[] [0, 0, 0, 0, 0, 0, 0, 0, 0, 0, 0, 0, 0, 0, 0, 0, 0, 0, 0, 0], "parameter.KGR"=dbl[] [0.0, 0.0, 0.0, 0.0, 0.0, 0.0, 0.0, 0.0, 0.0, 0.0, 0.0, 0.0, 0.0, 0.0, 0.0, 0.0, 0.0, 0.0, 0.0, 0.0], "parameter.consTime"=0, "parameter.trip"=bool[] [FALSE, FALSE, FALSE, FALSE, FALSE, FALSE, FALSE, FALSE, FALSE, FALSE, FALSE, FALSE, FALSE, FALSE, FALSE, FALSE, FALSE, FALSE, FALSE, FALSE]) -> (w836:T3)
      }
      frame "Initial Test Data1" {
        n605 = stacked-sequence {
          tunnel: w853 -> [_ _ w870]
          tunnel: [_ _ w869] -> w852
          frame #0 {
            n606 = property on="trippedStatus" class="Clust (strict)"() -> ("AllObjs[]"=w857:refnum<vi>[])  [unwired: 2 in, 2 out]
            n607 = for {
              tunnel: w857 -> [w861] mode=indexing
              tunnel: cluster{u32, u32}[] [{16711680, 16711680}, {6618880, 6618880}, {13816530, 16744703}, {3381759, 16777088}] ("Array") -> [w859]
              w862 = refnum<vi> refnum  # Boolean
              n608 = To More Specific Class(target class=w862, reference=w861) -> (specific class reference=w860:refnum<vi>)  [unwired: 1 in, 1 out]
              n609 = property class="Bool"(reference=w860, "Colors [4]"=w859) -> ()  [unwired: 1 in, 2 out]
            }
          }
          frame #1 {
            n610 = local write "LightCurtain"(FALSE ("LightCurtain")) -> ()
            n611 = local write "Voltage Reset"(FALSE ("Voltage Reset")) -> ()
            n612 = local write "No Current"(FALSE ("No Current")) -> ()
            n613 = Initialize Array(0.0 ("element"), 20 ("dimension size")) -> (w865:dbl[])
            n614 = local write "voltage"(w865) -> ()
          }
          frame #2 {
            w873 = FALSE ("Start")
            n615 = Bundle By Name(cluster=w870, "Period"=u8 0, "Elapse"=0, "Start"=w873, "Clear"=w873) -> (w869:T3)
          }
        }
      }
      frame "Initial Test UI" {
        n616 = stacked-sequence {
          tunnel: w874 -> [w878 _ _]
          frame #0 {
            n617 = Unbundle By Name(w878) -> ("parameter.unIndex"=w880:bool[], "parameter.MLFB Info.MLFB"=→"MLFB_show":string)
            n618 = control-ref of="trippedStatus"() -> (w879:refnum<vi>)
            n619 = call "InitialUninstall.vi"("unIndex"=w880, "Trip Status"=w879) -> ()  [unwired: 2 in]
          }
          frame #1 {
            n620 = local read "orderNum_P"() -> (→"orderNum_M":string)
            n621 = property on="Report" class="Bool (strict)"("DisabledEnum"=T18."Disabled and Grayed Out" ("Disabled")) -> ()  [unwired: 2 in, 2 out]
          }
          frame #2 {
            w884 = FALSE ("DisableCurtain")
            n622 = local write "DisableCurtain"(w884) -> ()
            n623 = local write "Fail"(w884) -> ()
            n624 = local write "Pass"(w884) -> ()
          }
        }
      }
      frame "Test Parameter" {
        w897 = dbl[] [1.05, 1.2]  # Action
        w896 = dbl[] [1.05, 1.2, 1.3, 1.4]  # Limit
        n625 = Get Date/Time String() -> (time string=→"StartTime":string)  [unwired: 3 in, 1 out]
        n626 = case shown="\"lowAction2\"" "TestModel" {
          tunnel: w888 -> [w915 w935 w955 w975 w996 w1017]
          tunnel: [w914 w934 w954 w974 w981 w1016] -> w890
          tunnel: [w910 w923 w951 w970 w980 w999] -> w893
          tunnel: [w898 w918 w938 w958 w979 w1014] -> w894
          tunnel: [w909 w933 w950 w969 w992 w1013] -> w892
          tunnel: w897 -> [_ _ w941 w968 _ _]
          tunnel: w896 -> [w908 w932 _ _ _ _]
          tunnel: w888 -> [w906 w922 w947 w961 w988 w1010]
          tunnel: w886 -> [w900 w921 w940 w960 w982 w1002]
          frame "lowLimit", Default {
            n627 = case shown="\"English\"" w900 {
              tunnel: ["极限电流小档" ("process") "Limit Lower" ("process")] -> w909
              frame "中文", Default {
              }
              frame "English" {
              }
            }
            n628 = Unbundle By Name(w906) -> ("File Path.limitTemplate"=w905:path, "parameter.MLFB Info.IL_Current"=w904:dbl, "parameter.MLFB Info.IL_KG"=w903:dbl, "parameter.MLFB Info.IL_consTIme"=w899:i32, "parameter.MLFB Info.Limit_P1"=w902:i32, "parameter.MLFB Info.Limit_P2"=w901:i32)
            n629 = call "TotalTime.vi"("factor"=3, "loadTime"=w901, "preloadTime"=w902) -> ("strSec"=w910:string, "strHour"=w898:string, "total"=w911:i32)
            n630 = Bundle By Name(cluster=w915, "parameter.KG20"=w908, "parameter.path.template (empty)"=w905, "parameter.baseCurrent"=w904, "parameter.KG"=w903, "parameter.Report.IL.consTime"=w899, "parameter.consTime"=w899, "parameter.Report.preLoad"=w902, "parameter.Report.Load"=w901, "parameter.Report.Total"=w911, "parameter.Report.IL.test?"=TRUE ("test?"), "parameter.UL?"=FALSE ("test?")) -> (w914:T3)
          }
          frame "upLimit" {
            n631 = Unbundle By Name(w922) -> ("File Path.limitTemplate"=w929:path, "parameter.MLFB Info.uL_Current"=w928:dbl, "parameter.MLFB Info.uL_KG"=w927:dbl, "parameter.MLFB Info.uL_consTIme"=w920:i32, "parameter.MLFB Info.Limit_P1"=w926:i32, "parameter.MLFB Info.Limit_P2"=w924:i32)
            n632 = case shown="\"中文\", Default" w921 {
              tunnel: ["极限电流大档" ("process") "Limit Upper" ("process")] -> w933
              frame "中文", Default {
              }
              frame "English" {
              }
            }
            n633 = call "TotalTime.vi"("factor"=3, "loadTime"=w924, "preloadTime"=w926) -> ("strSec"=w923:string, "strHour"=w918:string, "total"=w919:i32)
            n634 = Bundle By Name(cluster=w935, "parameter.KG20"=w932, "parameter.path.template (empty)"=w929, "parameter.baseCurrent"=w928, "parameter.KG"=w927, "parameter.Report.uL.consTime"=w920, "parameter.consTime"=w920, "parameter.Report.preLoad"=w926, "parameter.Report.Load"=w924, "parameter.Report.Total"=w919, "parameter.Report.uL.test?"=TRUE ("test?"), "parameter.UL?"=TRUE ("test?")) -> (w934:T3)
          }
          frame "lowAction1" {
            n635 = case shown="\"English\"" w940 {
              tunnel: ["动作特性1小档" ("process") "Action Lower 1" ("process")] -> w950
              frame "中文", Default {
              }
              frame "English" {
              }
            }
            n636 = Unbundle By Name(w947) -> ("File Path.actionTemplate"=w946:path, "parameter.MLFB Info.IL_Current"=w945:dbl, "parameter.MLFB Info.IL_KG"=w944:dbl, "parameter.MLFB Info.IL_consTIme"=w939:i32, "parameter.MLFB Info.Action_P1"=w943:i32, "parameter.MLFB Info.Action_P2"=w942:i32)
            n637 = call "TotalTime.vi"("factor"=1, "loadTime"=w942, "preloadTime"=w943) -> ("strSec"=w951:string, "strHour"=w938:string, "total"=w952:i32)
            n638 = Bundle By Name(cluster=w955, "parameter.KG20"=w941, "parameter.path.template (empty)"=w946, "parameter.baseCurrent"=w945, "parameter.KG"=w944, "parameter.Report.IL.consTime"=w939, "parameter.consTime"=w939, "parameter.Report.preLoad"=w943, "parameter.Report.Load"=w942, "parameter.Report.Total"=w952, "parameter.Report.IL.test?"=TRUE ("test?"), "parameter.UL?"=FALSE ("test?")) -> (w954:T3)
          }
          frame "upAction1" {
            n639 = Unbundle By Name(w961) -> ("parameter.path.template (empty)"=w966:path, "parameter.MLFB Info.uL_Current"=w965:dbl, "parameter.MLFB Info.uL_KG"=w964:dbl, "parameter.MLFB Info.uL_consTIme"=w959:i32, "parameter.MLFB Info.Action_P1"=w962:i32, "parameter.MLFB Info.Action_P2"=w963:i32)
            n640 = case shown="\"English\"" w960 {
              tunnel: ["动作特性1大档" ("process") "Action Upper 1" ("process")] -> w969
              frame "中文", Default {
              }
              frame "English" {
              }
            }
            n641 = call "TotalTime.vi"("factor"=1, "loadTime"=w963, "preloadTime"=w962) -> ("strSec"=w970:string, "strHour"=w958:string, "total"=w971:i32)
            n642 = Bundle By Name(cluster=w975, "parameter.KG20"=w968, "parameter.path.template (empty)"=w966, "parameter.baseCurrent"=w965, "parameter.KG"=w964, "parameter.Report.uL.consTime"=w959, "parameter.consTime"=w959, "parameter.Report.preLoad"=w962, "parameter.Report.Load"=w963, "parameter.Report.Total"=w971, "parameter.Report.uL.test?"=TRUE ("test?"), "parameter.UL?"=TRUE ("test?")) -> (w974:T3)
          }
          frame "lowAction2" {
            n643 = local read "action2preload"() -> (w983:i32)
            n644 = Unbundle By Name(w988) -> ("File Path.actionTemplate"=w987:path, "parameter.MLFB Info.IL_Current"=w986:dbl, "parameter.MLFB Info.IL_KG"=w985:dbl, "parameter.MLFB Info.IL_consTIme"=w978:i32)
            n645 = case shown="\"English\"" w982 {
              tunnel: ["动作特性2小档" ("process") "Action Lower 2" ("process")] -> w992
              frame "中文", Default {
              }
              frame "English" {
              }
            }
            n646 = local read "action2"() -> (w984:i32)
            n647 = call "TotalTime.vi"("factor"=0, "loadTime"=w984, "preloadTime"=w983) -> ("strSec"=w980:string, "strHour"=w979:string, "total"=w993:i32)
            n648 = Build Array(7.2) -> (w990:dbl[])
            n649 = Bundle By Name(cluster=w996, "parameter.KG20"=w990, "parameter.path.template (empty)"=w987, "parameter.baseCurrent"=w986, "parameter.KG"=w985, "parameter.Report.IL.consTime"=w978, "parameter.consTime"=w978, "parameter.Report.preLoad"=w983, "parameter.Report.Load"=w984, "parameter.Report.Total"=w993, "parameter.Report.IL.test?"=TRUE ("test?"), "parameter.UL?"=FALSE ("test?")) -> (w981:T3)
          }
          frame "upAction2" {
            n650 = Unbundle By Name(w1010) -> ("File Path.actionTemplate"=w1009:path, "parameter.MLFB Info.uL_Current"=w1008:dbl, "parameter.MLFB Info.uL_KG"=w1007:dbl, "parameter.MLFB Info.uL_consTIme"=w1001:i32)
            n651 = local read "action2preload"() -> (w1006:i32)
            n652 = case shown="\"English\"" w1002 {
              tunnel: ["动作特性2大档" ("process") "Action Upper 2" ("process")] -> w1013
              frame "中文", Default {
              }
              frame "English" {
              }
            }
            n653 = local read "action2"() -> (w1005:i32)
            n654 = Build Array(7.2) -> (w1011:dbl[])
            n655 = call "TotalTime.vi"("factor"=0, "loadTime"=w1005, "preloadTime"=w1006) -> ("strSec"=w999:string, "strHour"=w1014:string, "total"=w1000:i32)
            n656 = Bundle By Name(cluster=w1017, "parameter.KG20"=w1011, "parameter.path.template (empty)"=w1009, "parameter.baseCurrent"=w1008, "parameter.KG"=w1007, "parameter.Report.uL.consTime"=w1001, "parameter.consTime"=w1001, "parameter.Report.preLoad"=w1006, "parameter.Report.Load"=w1005, "parameter.Report.Total"=w1000, "parameter.Report.uL.test?"=TRUE ("test?"), "parameter.UL?"=TRUE ("test?")) -> (w1016:T3)
          }
        }
        "totalHour" <- w894
        "totalSec" <- w893
        "process" <- w892
      }
      frame "PowerRemote" {
        n657 = Unbundle By Name(w1026) -> ("parameter.Instr.pwr485"=w1028:refnum<visa-resource-name>)
        n658 = call "NewPower_Init.vi"("error in"=w1029, "Language"=w1022, "power485"=w1028) -> ("error out"=w1027:errorcluster, "Message"=w1021:string)
        n659 = local read "RunInfo"() -> (w1023:string)
        n660 = Concatenate Strings(w1023, w1021, "\r") -> (w1024:string)
        n661 = local write "RunInfo"(w1024) -> ()
      }
      frame "PowerON" {
        n662 = Unbundle By Name(w1039) -> ("parameter.testCurrent"=w1032:dbl, "parameter.Instr.pwr485"=w1042:refnum<visa-resource-name>, "parameter.pwrSwitch"=w1043:refnum<k21>)
        n663 = call "NewPower_Current.vi"("testCurrent"=w1032, "error in"=w1045, "Language"=w1031, "pwrSwitch"=w1043, "power485"=w1042) -> ("error out"=w1041:errorcluster, "switch"=w1037:bool[], "Message"=w1035:string)  [unwired: 4 in]
        n664 = local read "RunInfo"() -> (w1036:string)
        n665 = Bundle By Name(cluster=w1039, "parameter.buffer.PowerSwitch"=w1037) -> (w1038:T3)
        n666 = Concatenate Strings(w1036, w1035, "\r") -> (w1033:string)
        n667 = local write "RunInfo"(w1033) -> ()
      }
      frame "PowerCalibration" {
        n668 = Unbundle By Name(w1054) -> ("parameter.Instr.pwr485"=w1053:refnum<visa-resource-name>, "parameter.pwrSwitch"=w1050:refnum<k21>)
        n669 = call "NewPower_Current.vi"("testCurrent"="setCalibra", "error in"=w1055, "Language"=w1052, "pwrSwitch"=w1050, "power485"=w1053) -> ("error out"=w1048:errorcluster)  [unwired: 4 in, 2 out]
        n670 = call "DigitalWrite_MultiTask.vi"("error in"=w1048, "input"=bool[] [TRUE, TRUE], "mutiTask"=refnum<k21> "Power Calibration") -> ("error out"=w1047:errorcluster)  [unwired: 1 in]
      }
      frame "PowerOFF" {
        n671 = Unbundle By Name(w1064) -> ("parameter.Instr.pwr485"=w1066:refnum<visa-resource-name>, "parameter.pwrSwitch"=w1067:refnum<k21>)
        n672 = call "NewPower_Close.vi"("error in"=w1068, "Language"=w1058, "powerSwitch"=w1067, "power485"=w1066) -> ("error out"=w1065:errorcluster, "Message"=w1059:string)  [unwired: 6 in]
        n673 = local read "RunInfo"() -> (w1061:string)
        n674 = Concatenate Strings(w1061, w1059, "\r") -> (w1062:string)
        n675 = local write "RunInfo"(w1062) -> ()
      }
      frame "Temperature" {
        n676 = Unbundle By Name(w1076) -> ("parameter.Instr.34461"=w1077:refnum<visa-resource-name>, "parameter.Instr.PLC"=w1071:refnum<visa-resource-name>)
        n677 = local read "EnablePLC"() -> (w1070:i32)
        n678 = case shown="1" w1070 {
          tunnel: w1077 -> [_ w1092]
          tunnel: [20.0 ("Measurement") w1091] -> w1074
          tunnel: [w1081 w1090] -> w1073
          tunnel: w1072 -> [w1081 w1089]
          tunnel: w1071 -> [_ w1088]
          frame 0, Default {
          }
          frame 1 {
            w1087 = 8 items=["Continuity", "Current AC", "Current DC", "Diode", "Frequency", "Resistance 4-wire", "Period", "Resistance 2-wire", "Temperature", "Voltage AC", "Voltage DC", "Voltage DC Ratio"] ("Measurement Function (10: Voltage DC)")
            n679 = call-poly "PLC_OutPut.vi"("error in (no error)"=w1089, "Selection"=T19."Temperature", "Resistor"=24, "VISA resource name"=w1088) -> ("error out"=w1084:errorcluster)  [unwired: 1 in, 1 out]
            n680 = call "Delay"("error in (no error)"=w1084, "Delay Time (s)"=0.5) -> ("error out"=w1083:errorcluster)  [unwired: 9 in]
            n681 = call "Multi_Read_Single.vi"("error in"=w1083, "Measurement Function (10: Voltage DC)"=w1087, "VISA resource name"=w1092) -> ("error out"=w1090:errorcluster, "Measurement"=w1091:dbl)  [unwired: 7 in]
          }
        }
        n682 = Bundle By Name(cluster=w1076, "parameter.buffer.temp"=w1074) -> (w1075:T3)
      }
      frame "TempOffset" {
        n683 = Unbundle By Name(w1105) -> ("parameter.KTu"=w1108:dbl[], "parameter.KG20"=w1107:dbl[], "parameter.KG"=w1106:dbl, "parameter.baseCurrent"=w1101:dbl, "parameter.temperature"=w1098:dbl[], "parameter.buffer.temp"=w1097:dbl)
        n684 = call "Formula_6.2.vi"("temprature"=w1097, "KG"=w1106, "KG20"=w1107, "KTU In"=w1108) -> ("ktu"=w1102:dbl, "KTU Out"=w1103:dbl[])  [unwired: 6 in]
        n685 = Insert Into Array(array=w1098, new element=w1097) -> (w1093:dbl[])  [unwired: 1 in]
        n686 = Multiply(x=w1102, y=w1101) -> (x*y=w1100:dbl)
        "Current" <- w1100
        n687 = Bundle By Name(cluster=w1105, "parameter.KTu"=w1103, "parameter.testCurrent"=w1100, "parameter.temperature"=w1093, "Start"=FALSE) -> (w1104:T3)
      }
      frame "Trip" {
        n688 = Unbundle By Name(w1117) -> ("parameter.numTrip"=w1122:i32[], "Period"=w1114:u8, "parameter.uninstallNum"=w1124:i32, "parameter.Tripped Time"=w1125:i32[], "Elapse"=w1118:i32, "parameter.IO.Break"=w1115:refnum<k21>, "parameter.IO.Contactor"=w1116:refnum<k21>)
        n689 = local read "TestModel"() -> (w1111:T13)
        n690 = call "Test_Switch.vi"("TestModel"=w1111, "error in (no error)"=w1129, "Contactor"=w1116, "Break"=w1115) -> ("error out"=w1128:errorcluster, "Break"=w1123:bool[])
        n691 = call "Test_TripTime.vi"("error in (no error)"=w1128, "Break in"=w1123, "Time"=w1118, "Trip Time in"=w1125) -> ("error out"=w1127:errorcluster, "Trip Time out"=w1110:i32[])
        n692 = call "Test_numTrip.vi"("error in"=w1127, "numUninstall"=w1124, "Break"=w1123) -> ("error out"=w1109:errorcluster, "tripped count"=w1112:i32, "numTrip"=w1113:i32)
        n693 = Replace Array Subset(array=w1122, new element=w1113, index=w1114) -> (w1119:i32[])
        n694 = Bundle By Name(cluster=w1117, "parameter.Tripped Time"=w1110, "parameter.trip"=w1123, "parameter.numTrip"=w1119, "TrippedCount"=w1112) -> (w1120:T3)
      }
      frame "ShowInfo" {
        n695 = stacked-sequence {
          tunnel: w1131 -> [w1141 w1148 w1151]
          frame #0 {
            n696 = Unbundle By Name(w1141) -> ("parameter.Report.preLoad"=w1140:i32, "parameter.Report.Load"=w1139:i32, "Period"=w1135:u8, "Elapse"=w1138:i32)
            n697 = call "Test_Remain.vi"("elapsed"=w1138, "Period"=w1135, "load"=w1139, "preload"=w1140) -> ("used"=→"Total":string, "Period"=w1136:string, "remain"=→"remaing":string)
            n698 = property on="remaing" class="Str"("Caption.Text"=w1136) -> ()  [unwired: 2 in, 2 out]
          }
          frame #1 {
            n699 = Unbundle By Name(w1148) -> ("Period"=w1146:u8, "parameter.numTrip"=w1145:i32[], "parameter.KTu"=w1144:dbl[], "parameter.KG20"=w1143:dbl[], "parameter.temperature"=w1142:dbl[])
            n700 = call "MultiTest Status.vi"("numTrip"=w1145, "Period"=w1146, "KTu"=w1144, "KG20"=w1143, "temperature"=w1142) -> ("Status"=w1147:string[][])
            n701 = property on="parameter" class="MCListbox (strict)"("ItemNames"=w1147) -> ()  [unwired: 2 in, 2 out]
          }
          frame #2 {
            n702 = Unbundle By Name(w1151) -> ("parameter.trip"=w1149:bool[])
            n703 = Array To Cluster(array=w1149) -> (cluster=→"trippedStatus":T24)
          }
        }
      }
      frame "Finish?" {
        n704 = Unbundle By Name(w1153) -> ("parameter.trip"=w1165:bool[], "parameter.Report.Total"=w1157:i32, "Elapse"=w1155:i32)
        n705 = local read "No Current"() -> (w1154:bool)
        n706 = local read "Run?"() -> (w1162:bool)
        n707 = Or Array Elements(Boolean array=w1165) -> (logical OR=w1164:bool)
        n708 = Not(x=w1162) -> (.not. x?=w1156:bool)
        n709 = Less Or Equal?(x=w1157, y=w1155) -> (x <= y?=w1163:bool)
        n710 = Not(x=w1164) -> (.not. x?=w1159:bool)
        n711 = Compound Arithmetic op=OR(w1159, w1163, w1156, w1154) -> (w1161:bool)
        n712 = case shown="False" w1161 {
          tunnel: w1160 -> [w1170 _]
          tunnel: [w1169 w1179] -> w1158
          frame False {
            # "Keep testing"
            n713 = call "Elapsed Time"("Time Target (s)"=60.0) -> ("Time has Elapsed"=w1167:bool)  [unwired: 11 in, 7 out]
            n714 = case shown="True" w1167 {
              tunnel: w1170 -> [w1171 w1176]
              tunnel: [w1171 w1175] -> w1169
              frame False {
              }
              frame True {
                n715 = Insert Into Array(array=w1176, index=0, new element #1=Process."LoopCurrent" ("new element/subarray"), new element #2=Process."CheckLoopCurrent" ("new element/subarray")) -> (w1175:T16[])
              }
            }
          }
          frame True {
            w1179 = T16[] [enum."PowerOFF", enum."ShowTripTime", enum."Release HW Source", enum."TestResult", enum."Procedure"] items=["Initial_Data", "Initial_HMI", "Language", "UI", "Login", "Authority", "Clear", "Initial Test Data", "Initial Test Data1", "Initial Test UI", "Test Parameter", "PowerRemote", "PowerON", "PowerCalibration", "PowerOFF", "Temperature", "TempOffset", "Trip", "ShowInfo", "Finish?", "Period?", "LoopCurrent", "Procedure", "KGR", "Passed", "Failed", "MLFB Decoding", "MLFB Test Info", "MLFB Edit Info", "MLFB Edit", "MLFB Insert", "MLFB Delete", "ReportGeneralInfo", "ReportResultInfo", "ReportPath", "Generate Report", "Print Report", "New User", "Edit User", "Delete User", "Read User", "Voltage", "Time", "Current Calibration", "ErrorHandle", "StartTest", "ActiveLightCur", "Uninstall Record", "Get Uninstall Count", "Abort Test", "Test Model?", "CheckLoopCurrent", "Release HW Source", "Exit", "Close DB Connection", "Test UI BTN Status", "unTest UI BTN Status", "Disable All BTN", "AbortCalibration", "TprCalibration", "ClearReportInfo", "Set Uninstall", "TestResult", "SetLightCur", "CheckVoltage", "ShowTripTime"]
            # "Abort Test"
            n716 = local write "Abort"(TRUE ("Abort")) -> ()
            n717 = Get Date/Time String() -> (time string=→"EndTime":string)  [unwired: 3 in, 1 out]
          }
        }
      }
      frame "Period?" {
        n718 = Unbundle By Name(w1182) -> ("Period"=w1183:u8, "parameter.Report.Load"=w1191:i32, "parameter.Report.preLoad"=w1184:i32, "Elapse"=w1185:i32)
        n719 = local read "TestModel"() -> (w1180:T13)
        n720 = Multiply(x=w1183, y=w1191) -> (x*y=w1190:i32)
        n721 = Add(x=w1190, y=w1184) -> (x+y=w1189:i32)
        n722 = Less Or Equal?(x=w1189, y=w1185) -> (x <= y?=w1188:bool)
        n723 = case shown="False" w1188 {
          tunnel: [w1195 w1204] -> w1187
          tunnel: w1183 -> [_ w1202]
          tunnel: [w1194 w1203] -> w1186
          tunnel: w1182 -> [w1194 w1199]
          tunnel: w1180 -> [w1193 _]
          frame False {
            # "Current Period"
            n724 = case shown="\"lowAction2\", \"upAction2\"" w1193 {
              tunnel: [w1196 w1197] -> w1195
              frame "lowLimit", Default {
                w1196 = T16[] [enum."Time", enum."Trip", enum."ShowInfo", enum."Voltage", enum."Abort Test", enum."Finish?", enum."Period?"] items=["Initial_Data", "Initial_HMI", "Language", "UI", "Login", "Authority", "Clear", "Initial Test Data", "Initial Test Data1", "Initial Test UI", "Test Parameter", "PowerRemote", "PowerON", "PowerCalibration", "PowerOFF", "Temperature", "TempOffset", "Trip", "ShowInfo", "Finish?", "Period?", "LoopCurrent", "Procedure", "KGR", "Passed", "Failed", "MLFB Decoding", "MLFB Test Info", "MLFB Edit Info", "MLFB Edit", "MLFB Insert", "MLFB Delete", "ReportGeneralInfo", "ReportResultInfo", "ReportPath", "Generate Report", "Print Report", "New User", "Edit User", "Delete User", "Read User", "Voltage", "Time", "Current Calibration", "ErrorHandle", "StartTest", "ActiveLightCur", "Uninstall Record", "Get Uninstall Count", "Abort Test", "Test Model?", "CheckLoopCurrent", "Release HW Source", "Exit", "Close DB Connection", "Test UI BTN Status", "unTest UI BTN Status", "Disable All BTN", "AbortCalibration", "TprCalibration", "ClearReportInfo", "Set Uninstall", "TestResult", "SetLightCur", "CheckVoltage", "ShowTripTime"]
              }
              frame "lowAction2", "upAction2" {
                w1197 = T16[] [enum."Time", enum."Trip", enum."ShowInfo", enum."Abort Test", enum."Finish?", enum."Period?"] items=["Initial_Data", "Initial_HMI", "Language", "UI", "Login", "Authority", "Clear", "Initial Test Data", "Initial Test Data1", "Initial Test UI", "Test Parameter", "PowerRemote", "PowerON", "PowerCalibration", "PowerOFF", "Temperature", "TempOffset", "Trip", "ShowInfo", "Finish?", "Period?", "LoopCurrent", "Procedure", "KGR", "Passed", "Failed", "MLFB Decoding", "MLFB Test Info", "MLFB Edit Info", "MLFB Edit", "MLFB Insert", "MLFB Delete", "ReportGeneralInfo", "ReportResultInfo", "ReportPath", "Generate Report", "Print Report", "New User", "Edit User", "Delete User", "Read User", "Voltage", "Time", "Current Calibration", "ErrorHandle", "StartTest", "ActiveLightCur", "Uninstall Record", "Get Uninstall Count", "Abort Test", "Test Model?", "CheckLoopCurrent", "Release HW Source", "Exit", "Close DB Connection", "Test UI BTN Status", "unTest UI BTN Status", "Disable All BTN", "AbortCalibration", "TprCalibration", "ClearReportInfo", "Set Uninstall", "TestResult", "SetLightCur", "CheckVoltage", "ShowTripTime"]
              }
            }
          }
          frame True {
            w1204 = T16[] [enum."Time", enum."PowerOFF", enum."ShowTripTime", enum."Temperature", enum."TempOffset", enum."PowerON", enum."Time", enum."Time", enum."Trip", enum."ShowInfo", enum."LoopCurrent", enum."CheckLoopCurrent", enum."Abort Test", enum."Finish?", enum."Period?"] items=["Initial_Data", "Initial_HMI", "Language", "UI", "Login", "Authority", "Clear", "Initial Test Data", "Initial Test Data1", "Initial Test UI", "Test Parameter", "PowerRemote", "PowerON", "PowerCalibration", "PowerOFF", "Temperature", "TempOffset", "Trip", "ShowInfo", "Finish?", "Period?", "LoopCurrent", "Procedure", "KGR", "Passed", "Failed", "MLFB Decoding", "MLFB Test Info", "MLFB Edit Info", "MLFB Edit", "MLFB Insert", "MLFB Delete", "ReportGeneralInfo", "ReportResultInfo", "ReportPath", "Generate Report", "Print Report", "New User", "Edit User", "Delete User", "Read User", "Voltage", "Time", "Current Calibration", "ErrorHandle", "StartTest", "ActiveLightCur", "Uninstall Record", "Get Uninstall Count", "Abort Test", "Test Model?", "CheckLoopCurrent", "Release HW Source", "Exit", "Close DB Connection", "Test UI BTN Status", "unTest UI BTN Status", "Disable All BTN", "AbortCalibration", "TprCalibration", "ClearReportInfo", "Set Uninstall", "TestResult", "SetLightCur", "CheckVoltage", "ShowTripTime"]
            # "Next Period"
            n725 = Unbundle By Name(w1199) -> ("TrippedCount"=w1198:i32)
            n726 = Increment(x=w1202) -> (x+1=w1200:u8)
            n727 = Bundle By Name(cluster=w1199, "parameter.uninstallNum"=w1198, "Start"=TRUE ("Hold On"), "Period"=w1200) -> (w1203:T3)
          }
        }
      }
      frame "LoopCurrent" {
        n728 = Unbundle By Name(w1213) -> ("parameter.Instr.pwr485"=w1212:refnum<visa-resource-name>, "parameter.testCurrent"=w1211:dbl)
        n729 = Greater Or Equal?(x=w1211, y=5.0) -> (x >= y?=w1205:bool)
        n730 = Select(t=addrPower."300A power" ("addrPower"), s=w1205, f=addrPower."5A power" ("addrPower")) -> (s? t:f=w1207:T8)
        n731 = call "NewPower_GetCurrent.vi"("error in"=w1215, "addrPower"=w1207, "pwr485"=w1212) -> ("error out"=w1214:errorcluster, "Current"=→"current" →"valueCalibra":dbl)  [unwired: 1 in]
      }
      frame "Procedure" {
        w1219 = T16[] [enum."UI"] items=["Initial_Data", "Initial_HMI", "Language", "UI", "Login", "Authority", "Clear", "Initial Test Data", "Initial Test Data1", "Initial Test UI", "Test Parameter", "PowerRemote", "PowerON", "PowerCalibration", "PowerOFF", "Temperature", "TempOffset", "Trip", "ShowInfo", "Finish?", "Period?", "LoopCurrent", "Procedure", "KGR", "Passed", "Failed", "MLFB Decoding", "MLFB Test Info", "MLFB Edit Info", "MLFB Edit", "MLFB Insert", "MLFB Delete", "ReportGeneralInfo", "ReportResultInfo", "ReportPath", "Generate Report", "Print Report", "New User", "Edit User", "Delete User", "Read User", "Voltage", "Time", "Current Calibration", "ErrorHandle", "StartTest", "ActiveLightCur", "Uninstall Record", "Get Uninstall Count", "Abort Test", "Test Model?", "CheckLoopCurrent", "Release HW Source", "Exit", "Close DB Connection", "Test UI BTN Status", "unTest UI BTN Status", "Disable All BTN", "AbortCalibration", "TprCalibration", "ClearReportInfo", "Set Uninstall", "TestResult", "SetLightCur", "CheckVoltage", "ShowTripTime"]
      }
      frame "KGR" {
        n732 = Unbundle By Name(w1224) -> ("parameter.Tripped Time"=w1226:i32[], "parameter.Report.preLoad"=w1227:i32, "parameter.Report.Load"=w1228:i32, "parameter.consTime"=w1229:i32, "parameter.KG20"=w1225:dbl[])
        n733 = call "Formula_KG.vi"("KTu"=w1225, "Tripped Time"=w1226, "error in"=w1231, "consTime"=w1229, "Load Time"=w1228, "Preload Time"=w1227) -> ("error out"=w1230:errorcluster, "KGR"=w1222:dbl[])  [unwired: 4 in]
        n734 = Bundle By Name(cluster=w1224, "parameter.KGR"=w1222) -> (w1223:T3)
      }
      frame "Passed" {
        n735 = stacked-sequence {
          tunnel: w1236 -> [w1240 _ w1254]
          tunnel: [_ _ w1253] -> w1235
          tunnel: w1234 -> [_ w1246 _]
          frame #0 {
            n736 = Unbundle By Name(w1240) -> ("parameter.Authority"=w1241:u32)
            n737 = case shown="0, Default" w1241 {
              frame 1 {
                w1242 = T18."Enabled" ("Disabled")
                # "engineer"
                n738 = property on="Report" class="Bool (strict)"("DisabledEnum"=w1242) -> ()  [unwired: 2 in, 2 out]
                n739 = property on="Start" class="Bool"("DisabledEnum"=w1242) -> ()  [unwired: 2 in, 2 out]
                n740 = property on="New" class="Bool"("DisabledEnum"=w1242) -> ()  [unwired: 2 in, 2 out]
                n741 = property on="btnAbort" class="Bool (strict)"("DisabledEnum"=T18."Disabled and Grayed Out" ("Disabled")) -> ()  [unwired: 2 in, 2 out]
                n742 = property on="Edit" class="Bool"("DisabledEnum"=w1242) -> ()  [unwired: 2 in, 2 out]
                n743 = property on="Set" class="Bool"("DisabledEnum"=w1242) -> ()  [unwired: 2 in, 2 out]
                n744 = property on="exit" class="Bool"("DisabledEnum"=w1242) -> ()  [unwired: 2 in, 2 out]
              }
              frame 0, Default {
                w1244 = T18."Enabled" ("Disabled")
                # "worker"
                n745 = property on="Start" class="Bool"("DisabledEnum"=w1244) -> ()  [unwired: 2 in, 2 out]
                n746 = property on="Report" class="Bool (strict)"("DisabledEnum"=w1244) -> ()  [unwired: 2 in, 2 out]
                n747 = property on="exit" class="Bool"("DisabledEnum"=w1244) -> ()  [unwired: 2 in, 2 out]
                n748 = property on="btnAbort" class="Bool (strict)"("DisabledEnum"=T18."Disabled and Grayed Out" ("Disabled")) -> ()  [unwired: 2 in, 2 out]
              }
            }
          }
          frame #1 {
            n749 = case shown="\"中文\", Default" w1246 {
              tunnel: ["测试完成" "Test done"] -> w1249
              frame "中文", Default {
              }
              frame "English" {
              }
            }
            n750 = local read "RunInfo"() -> (w1247:string)
            n751 = Concatenate Strings(w1247, w1249, "\r") -> (w1248:string)
            n752 = local write "RunInfo"(w1248) -> ()
          }
          frame #2 {
            n753 = Unbundle By Name(w1254) -> ("Test Count"=w1255:u8)
            n754 = Increment(x=w1255) -> (x+1=w1256:u8)
            n755 = Bundle By Name(cluster=w1254, "Test Count"=w1256) -> (w1253:T3)
            "Pass" <- TRUE ("Pass")
          }
        }
      }
      frame "Failed" {
        n756 = stacked-sequence {
          tunnel: w1259 -> [w1264 _]
          tunnel: w1258 -> [_ w1269]
          frame #0 {
            n757 = Unbundle By Name(w1264) -> ("parameter.Authority"=w1263:u32)
            n758 = case shown="1" w1263 {
              frame 1 {
                w1265 = T18."Disabled and Grayed Out" ("Disabled")
                w1266 = T18."Enabled" ("Disabled")
                # "engineer"
                n759 = property on="Start" class="Bool"("DisabledEnum"=w1266) -> ()  [unwired: 2 in, 2 out]
                n760 = property on="New" class="Bool"("DisabledEnum"=w1266) -> ()  [unwired: 2 in, 2 out]
                n761 = property on="Edit" class="Bool"("DisabledEnum"=w1266) -> ()  [unwired: 2 in, 2 out]
                n762 = property on="Set" class="Bool"("DisabledEnum"=w1266) -> ()  [unwired: 2 in, 2 out]
                n763 = property on="exit" class="Bool"("DisabledEnum"=w1266) -> ()  [unwired: 2 in, 2 out]
                n764 = property on="btnAbort" class="Bool (strict)"("DisabledEnum"=w1265) -> ()  [unwired: 2 in, 2 out]
                n765 = property on="Report" class="Bool (strict)"("DisabledEnum"=w1265) -> ()  [unwired: 2 in, 2 out]
              }
              frame 0, Default {
                w1268 = T18."Enabled" ("Disabled")
                w1267 = T18."Disabled and Grayed Out" ("Disabled")
                # "worker"
                n766 = property on="Start" class="Bool"("DisabledEnum"=w1268) -> ()  [unwired: 2 in, 2 out]
                n767 = property on="exit" class="Bool"("DisabledEnum"=w1268) -> ()  [unwired: 2 in, 2 out]
                n768 = property on="btnAbort" class="Bool (strict)"("DisabledEnum"=w1267) -> ()  [unwired: 2 in, 2 out]
                n769 = property on="Report" class="Bool (strict)"("DisabledEnum"=w1267) -> ()  [unwired: 2 in, 2 out]
              }
            }
          }
          frame #1 {
            n770 = case shown="\"中文\", Default" w1269 {
              tunnel: ["测试失败" "Test failed"] -> w1274
              frame "中文", Default {
              }
              frame "English" {
              }
            }
            n771 = local read "RunInfo"() -> (w1271:string)
            n772 = Concatenate Strings(w1271, w1274, "\r") -> (w1272:string)
            n773 = local write "RunInfo"(w1272) -> ()
            "Fail" <- TRUE ("Fail")
          }
        }
      }
      frame "MLFB Decoding" {
        n774 = Unbundle By Name(w1288) -> ("parameter.MLFB"=w1283:T9, "parameter.MLFB Info.MLFB"=w1279:string)
        n775 = call "Database_Query.vi"("error in (no error)"=w1286, "Column"=w1279, "Table"="Products", "connection reference"=w1283) -> ("error out"=w1284:errorcluster, "size(s)"=w1281:i32, "connection reference 2"=w1280:T9)
        n776 = Not Equal To 0?(x=w1281) -> (x != 0?=w1282:bool)
        n777 = case shown="False" w1282 {
          tunnel: w1288 -> [w1297 w1308]
          tunnel: [w1297 w1307] -> w1287
          tunnel: [w1295 w1305] -> w1277
          tunnel: w1284 -> [w1295 w1304]
          tunnel: w1280 -> [_ w1303]
          tunnel: w1279 -> [_ w1302]
          tunnel: w1278 -> [w1296 w1301]
          frame False {
            n778 = case shown="\"English\"" w1296 {
              tunnel: ["MLFB无效" "Invalid MLFB"] -> w1293
              frame "中文" {
              }
              frame "English" {
              }
            }
            n779 = Unbundle By Name(w1295) -> ("source"=w1292:string)
            n780 = Concatenate Strings(w1293, "\r", w1292) -> (w1291:string)
            n781 = One Button Dialog(message=w1291) -> ()  [unwired: 1 in, 1 out]
          }
          frame True {
            n782 = call "Database_MLFB_Decoding.vi"("error in"=w1304, "Language"=w1301, "MLFB"=w1302, "connection reference"=w1303) -> ("error out"=w1305:errorcluster, "Message"=w1300:string, "MLFB_DATA"=w1306:T5)  [unwired: 1 out]
            n783 = Bundle By Name(cluster=w1308, "parameter.MLFB Info"=w1306) -> (w1307:T3)
            n784 = One Button Dialog(message=w1300) -> ()  [unwired: 1 in, 1 out]
          }
        }
      }
      frame "MLFB Test Info" {
        n785 = stacked-sequence {
          tunnel: w1309 -> [w1313 w1325 _]
          frame #0 {
            n786 = Unbundle By Name(w1313) -> ("parameter.MLFB Info.Frame"=→"Frame":string, "parameter.MLFB Info.IL_Current"=→"Current_IL":dbl, "parameter.MLFB Info.IL_KG"=→"KG20_IL":dbl, "parameter.MLFB Info.IL_consTIme"=→"consTime_IL":i32, "parameter.MLFB Info.uL_Current"=→"Current_uL":dbl, "parameter.MLFB Info.uL_KG"=→"KG20_uL":dbl, "parameter.MLFB Info.uL_consTIme"=→"consTime_uL":i32, "parameter.MLFB Info.DA"=→"DA_IL" →"DA_uL":dbl)
          }
          frame #1 {
            n787 = Unbundle By Name(w1325) -> ("parameter.buffer.temp"=w1322:dbl, "parameter.MLFB Info.Action_P1"=→"preload_Action":i32, "parameter.MLFB Info.Action_P2"=→"load_Action":i32, "parameter.MLFB Info.Limit_P1"=→"preload_Limit":i32, "parameter.MLFB Info.Limit_P2"=→"load_Limit":i32, "parameter.MLFB Info.reTemperature"=→"Reference temp":i32, "parameter.MLFB Info.iGauge"=→"Gauge_In":dbl, "parameter.MLFB Info.oGauge"=→"Gauge_Out":dbl, "parameter.MLFB Info.Torque"=→"Torque":string)
            n788 = Number To Fractional String(number=w1322, precision (6)=i16 2) -> (F-format string=→"Temperature":string)  [unwired: 2 in]
          }
          frame #2 {
            n789 = local read "Operator"() -> (→"Operator_test":string)
            n790 = Get Date/Time String() -> (date string=→"Test Date":string)  [unwired: 3 in, 1 out]
            n791 = property on="ok_Para" class="Bool"("DisabledEnum"=T18."Enabled" ("Disabled")) -> ()  [unwired: 2 in, 2 out]
          }
        }
      }
      frame "MLFB Edit Info" {
        n792 = stacked-sequence {
          tunnel: w1337 -> [w1341 w1352]
          frame #0 {
            n793 = Unbundle By Name(w1341) -> ("parameter.MLFB Info.Frame"=w1351:string, "parameter.MLFB Info.curRange"=w1350:string, "parameter.MLFB Info.thermoRs"=w1349:dbl, "parameter.MLFB Info.releaseRs"=w1348:dbl, "parameter.MLFB Info.circuitRs"=w1347:dbl, "parameter.MLFB Info.IL_Current"=w1346:dbl, "parameter.MLFB Info.IL_KG"=w1345:dbl, "parameter.MLFB Info.IL_consTIme"=w1344:i32, "parameter.MLFB Info.uL_Current"=w1343:dbl, "parameter.MLFB Info.uL_KG"=w1342:dbl)
            n794 = local write "Frame E"(w1351) -> ()
            n795 = local write "curRange E"(w1350) -> ()
            n796 = local write "thermoRs E"(w1349) -> ()
            n797 = local write "releaseRs E"(w1348) -> ()
            n798 = local write "circuitRs E"(w1347) -> ()
            n799 = local write "Current_IL E"(w1346) -> ()
            n800 = local write "KG_IL E"(w1345) -> ()
            n801 = local write "consTime_IL E"(w1344) -> ()
            n802 = local write "Current_uL E"(w1343) -> ()
            n803 = local write "KG_uL E"(w1342) -> ()
          }
          frame #1 {
            n804 = Unbundle By Name(w1352) -> ("parameter.MLFB Info.uL_consTIme"=w1362:i32, "parameter.MLFB Info.DA"=w1361:dbl, "parameter.MLFB Info.Action_P1"=w1360:i32, "parameter.MLFB Info.Action_P2"=w1359:i32, "parameter.MLFB Info.Limit_P1"=w1358:i32, "parameter.MLFB Info.Limit_P2"=w1357:i32, "parameter.MLFB Info.reTemperature"=w1356:i32, "parameter.MLFB Info.iGauge"=w1355:dbl, "parameter.MLFB Info.oGauge"=w1354:dbl, "parameter.MLFB Info.Torque"=w1353:string)
            n805 = local write "consTime_uL E"(w1362) -> ()
            n806 = local write "DA E"(w1361) -> ()
            n807 = local write "Preload_Action E"(w1360) -> ()
            n808 = local write "Load_Action E"(w1359) -> ()
            n809 = local write "Preload_Limit E"(w1358) -> ()
            n810 = local write "Load_Limit E"(w1357) -> ()
            n811 = local write "reTemperature E"(w1356) -> ()
            n812 = local write "Gauge_In E"(w1355) -> ()
            n813 = local write "Gauge_Out E"(w1354) -> ()
            n814 = local write "Torque E"(w1353) -> ()
          }
        }
      }
      frame "MLFB Edit" {
        n815 = Unbundle By Name(w1372) -> ("parameter.MLFB"=w1370:T9, "parameter.MLFB Info"=w1366:T5)
        n816 = for {
          N: 4 -> [_]
          shift-right: [w1375] -> w1365
          shift-left: w1366 -> [w1374]
          i -> [w1376]
          n817 = case shown="1" w1376 {
            tunnel: [w1384 w1392 w1398 w1404] -> w1375
            tunnel: w1374 -> [w1383 w1393 w1399 w1405]
            frame 0, Default {
              n818 = Bundle By Name(cluster=w1383, "MLFB"="MLFB E", "Frame"="Frame E", "curRange"="curRange E", "thermoRs"="thermoRs E", "releaseRs"="releaseRs E", "circuitRs"="circuitRs E") -> (w1384:T5)
            }
            frame 1 {
              n819 = Bundle By Name(cluster=w1393, "IL_Current"="Current_IL E", "IL_KG"="KG_IL E", "IL_consTIme"="consTime_IL E", "uL_Current"="Current_uL E", "uL_KG"="KG_uL E", "uL_consTIme"="consTime_uL E", "DA"="DA E") -> (w1392:T5)
            }
            frame 2 {
              n820 = Bundle By Name(cluster=w1399, "Action_P1"="Preload_Action E", "Action_P2"="Load_Action E", "Limit_P1"="Preload_Limit E", "Limit_P2"="Load_Limit E", "Limit_P3"="Load_Limit E", "Limit_P4"="Load_Limit E") -> (w1398:T5)
            }
            frame 3 {
              n821 = Bundle By Name(cluster=w1405, "reTemperature"="reTemperature E", "iGauge"="Gauge_In E", "oGauge"="Gauge_Out E", "Torque"="Torque E") -> (w1404:T5)
            }
          }
        }
        n822 = call "Database_MLFB_Edit.vi"("error in"=w1363, "Language"=w1368, "MLFB Data"=w1365, "connection reference"=w1370) -> ("error out"=w1371:errorcluster, "Message"=w1369:string)  [unwired: 1 out]
        n823 = One Button Dialog(message=w1369) -> ()  [unwired: 1 in, 1 out]
      }
      frame "MLFB Insert" {
        n824 = Unbundle By Name(w1415) -> ("parameter.MLFB"=w1412:T9, "parameter.MLFB Info"=w1409:T5)
        n825 = for {
          N: 4 -> [_]
          shift-right: [w1418] -> w1408
          shift-left: w1409 -> [w1417]
          i -> [w1419]
          n826 = case shown="3" w1419 {
            tunnel: [w1427 w1436 w1442 w1448] -> w1418
            tunnel: w1417 -> [w1420 w1428 w1437 w1443]
            frame 0, Default {
              n827 = Bundle By Name(cluster=w1420, "MLFB"="MLFB N", "Frame"="Frame N", "curRange"="curRange N", "thermoRs"="thermoRs", "releaseRs"="releaseRs", "circuitRs"="Resistance N") -> (w1427:T5)
            }
            frame 1 {
              n828 = Bundle By Name(cluster=w1428, "IL_Current"="Current_IL N", "IL_KG"="KG20_IL N", "IL_consTIme"="consTime_IL N", "uL_Current"="Current_uL N", "uL_KG"="KG20_uL N", "uL_consTIme"="consTime_uL N", "DA"="DA N") -> (w1436:T5)
            }
            frame 2 {
              n829 = Bundle By Name(cluster=w1437, "Action_P1"="Preload_Release N", "Action_P2"="Load_Release N", "Limit_P1"="Preload_Limit N", "Limit_P2"="Load_Limit N", "Limit_P3"="Load_Limit N", "Limit_P4"="Load_Limit N") -> (w1442:T5)
            }
            frame 3 {
              n830 = Bundle By Name(cluster=w1443, "reTemperature"="reTemperature N", "iGauge"="Gauge_In N", "oGauge"="Gauge_Out N", "Torque"="Torque N") -> (w1448:T5)
            }
          }
        }
        n831 = call "Database_MLFB_Insert.vi"("error in"=w1414, "Language"=w1410, "MLFB_Info"=w1408, "connection reference"=w1412) -> ("error out"=w1413:errorcluster, "Message"=w1411:string)  [unwired: 1 out]
        n832 = One Button Dialog(message=w1411) -> ()  [unwired: 1 in, 1 out]
      }
      frame "MLFB Delete" {
        n833 = Unbundle By Name(w1452) -> ("parameter.MLFB"=w1451:T9)
        n834 = local read "MLFB E"() -> (w1453:string)
        n835 = call "Database_MLFB_Delete.vi"("error in"=w1455, "Language"=w1449, "MLFB"=w1453, "connection reference"=w1451) -> ("error out"=w1454:errorcluster, "Message"=w1450:string)  [unwired: 1 out]
        n836 = One Button Dialog(message=w1450) -> ()  [unwired: 1 in, 1 out]
      }
      frame "ReportGeneralInfo" {
        n837 = Unbundle By Name(w1475) -> ("parameter.Report.preLoad"=w1474:i32, "parameter.Report.Load"=w1473:i32, "parameter.voltage"=w1472:dbl[], "parameter.MLFB Info.curRange"=w1471:string)
        n838 = local read "Test Date"() -> (w1465:string)
        n839 = local read "StartTime"() -> (w1464:string)
        n840 = local read "EndTime"() -> (w1463:string)
        n841 = local read "testCount"() -> (w1462:string)
        n842 = local read "Operator"() -> (w1461:string)
        n843 = local read "MLFB_show"() -> (w1460:string)
        n844 = Cluster To Array(cluster="Just Code") -> (array=w1469:string[])
        n845 = Bundle By Name(cluster=w1475, "parameter.Report.Title.预载荷时间"=w1474, "parameter.Report.Title.载荷时间"=w1473, "parameter.Report.Voltage"=w1472, "parameter.Report.Title.电流范围"=w1471, "parameter.Report.Title.订单数量"="orderCount", "parameter.Report.Title.订单号"="orderNum_P", "parameter.Report.Title.生产代码"="productCode", "parameter.Report.Title.日期"=w1465, "parameter.Report.Title.开始时间"=w1464, "parameter.Report.Title.结束时间"=w1463, "parameter.Report.Title.测试数量"=w1462, "parameter.Report.Title.检验员"=w1461, "parameter.Report.Title.MLFB"=w1460, "parameter.Report.Title.起动时间"="AccelerationTime", "parameter.Report.Title.快速时间范围"="ThermalTmFrame", "parameter.Report.JustCode"=w1469) -> (w1476:T3)
      }
      frame "ReportResultInfo" {
        n846 = Unbundle By Name(w1480) -> ("parameter.UL?"=w1491:bool, "parameter.KTu"=w1489:dbl[], "parameter.KG"=w1487:dbl, "parameter.temperature"=w1485:dbl[], "parameter.Tripped Time"=w1484:i32[], "parameter.KGR"=w1483:dbl[])
        n847 = Number To Fractional String(number=w1489, precision (6)=i16 2) -> (F-format string=w1488:string[])  [unwired: 2 in]
        n848 = Number To Fractional String(number=w1485, precision (6)=i16 2) -> (F-format string=w1482:string[])  [unwired: 2 in]
        n849 = case shown="True" w1491 {
          tunnel: [w1501 w1508] -> w1481
          tunnel: w1488 -> [w1500 w1507]
          tunnel: w1487 -> [w1496 w1503]
          tunnel: w1482 -> [w1499 w1506]
          tunnel: w1484 -> [w1498 w1505]
          tunnel: w1483 -> [w1497 w1504]
          tunnel: w1480 -> [w1495 w1502]
          frame False {
            # "IL"
            n850 = Bundle By Name(cluster=w1495, "parameter.Report.IL.KTU"=w1500, "parameter.Report.IL.KG"=w1496, "parameter.Report.IL.Testing temp"=w1499, "parameter.Report.IL.Tripped Time"=w1498, "parameter.Report.IL.KGR"=w1497) -> (w1501:T3)
          }
          frame True {
            # "uL"
            n851 = Bundle By Name(cluster=w1502, "parameter.Report.uL.KTU"=w1507, "parameter.Report.uL.KG"=w1503, "parameter.Report.uL.Testing temp"=w1506, "parameter.Report.uL.Tripped Time"=w1505, "parameter.Report.uL.KGR"=w1504) -> (w1508:T3)
          }
        }
      }
      frame "ReportPath" {
        n852 = Get Date/Time In Seconds() -> (seconds since 1Jan1904=w1516:timestamp)
        n853 = Unbundle By Name(w1509) -> ("File Path.initialPath"=w1523:path, "File Path.backupPath"=w1510:path)
        n854 = Format Date/Time String(time format string (%c)="%Y%m%d%#H", seconds (now)=w1516) -> (date/time string=w1515:string)  [unwired: 1 in]
        n855 = Concatenate Strings(w1515, ".xlsx") -> (w1511:string)
        n856 = call "File Dialog2"("start path"=w1523, "default name"=w1511, "error in"=w1524) -> ("selected path"=w1512:path, "cancelled"=w1521:bool, "error out"=w1513:errorcluster)  [unwired: 9 in, 1 out]
        n857 = Strip Path(path=w1512) -> (name=w1522:string)  [unwired: 1 out]
        n858 = Build Path(base path=w1510, name or relative path=w1522) -> (appended path=w1520:path)
        n859 = case shown="False" w1521 {
          tunnel: w1520 -> [w1529 _]
          tunnel: [w1528 w1530] -> w1519
          tunnel: w1512 -> [w1527 _]
          tunnel: w1509 -> [w1526 w1530]
          frame False {
            n860 = Bundle By Name(cluster=w1526, "parameter.path.Report path"=w1527, "parameter.path.Backup path"=w1529) -> (w1528:T3)
          }
          frame True {
          }
        }
      }
      frame "Generate Report" {
        n861 = stacked-sequence {
          tunnel: w1534 -> [_ w1540 _ _]
          tunnel: w1533 -> [_ w1539 _ w1552]
          tunnel: [_ w1538 _ _] -> w1532
          tunnel: [_ _ _ w1551] -> w1531
          frame #0 {
            n862 = property on="Report" class="Bool (strict)"("DisabledEnum"=T18."Disabled and Grayed Out" ("Disabled")) -> ()  [unwired: 2 in, 2 out]
          }
          frame #1 {
            n863 = Unbundle By Name(w1539) -> ("parameter.Report"=w1542:T6, "parameter.path.template (empty)"=w1543:path, "parameter.path.Report path"=w1544:path, "parameter.path.Backup path"=w1545:path)
            n864 = control-ref of="pirntProcess"() -> (w1546:refnum<vi>)
            n865 = call "Excel_Report.vi"("Process"=w1546, "Report"=w1542, "error in"=w1540, "Backup path"=w1545, "Report path"=w1544, "template (empty)"=w1543) -> ("error out"=w1538:errorcluster, "Message"=w1541:string)  [unwired: 4 in]
            n866 = local read "RunInfo"() -> (w1547:string)
            n867 = Concatenate Strings(w1547, w1541, "\r") -> (w1548:string)
            n868 = local write "RunInfo"(w1548) -> ()
          }
          frame #2 {
            n869 = property on="Report" class="Bool (strict)"("DisabledEnum"=T18."Enabled" ("Disabled")) -> ()  [unwired: 2 in, 2 out]
          }
          frame #3 {
            n870 = Bundle By Name(cluster=w1552, "Test Count"=u8 0) -> (w1551:T3)
          }
        }
      }
      frame "Print Report" {
        n871 = Unbundle By Name(w1563) -> ("parameter.path.Report path"=w1562:path)
        n872 = call "Print Report.vi"("error in"=w1561, "Language"=w1554, "Initial Path"=w1562) -> ("error IO"=w1557:errorcluster, "Message"=w1556:string)
        n873 = local read "RunInfo"() -> (w1559:string)
        n874 = Concatenate Strings(w1559, w1556, "\r") -> (w1558:string)
        n875 = local write "RunInfo"(w1558) -> ()
      }
      frame "New User" {
        n876 = Unbundle By Name(w1577) -> ("parameter.MLFB"=w1576:T9)
        n877 = Empty String/Path?(string/path="txtID") -> (empty?=w1569:bool)
        n878 = Empty String/Path?(string/path="txtName") -> (empty?=w1568:bool)
        n879 = Empty String/Path?(string/path="txtPassword") -> (empty?=w1567:bool)
        n880 = Compound Arithmetic op=OR(w1569, w1568, w1567) -> (w1566:bool)
        n881 = case shown="False" w1566 {
          tunnel: w1576 -> [w1589 _]
          tunnel: "txtID" -> [w1587 _]
          tunnel: "txtName" -> [w1586 _]
          tunnel: "txtPassword" -> [w1585 _]
          tunnel: w1565 -> [w1583 w1593]
          tunnel: [w1580 w1593] -> w1575
          tunnel: w1573 -> [w1581 w1592]
          frame False {
            n882 = Bundle(cluster=T20 {"ID_Number"="", "Name"="", "Password"="", "Authority"=0} ("UserRight"), "ID_Number"=w1587, "Name"=w1586, "Password"=w1585, "Authority"="Authority") -> (w1584:T20)
            n883 = call "Database_User_Add.vi"("error in"=w1583, "Language"=w1581, "User Info"=w1584, "connection reference"=w1589) -> ("error out"=w1580:errorcluster, "Message"=w1582:string)  [unwired: 1 in, 1 out]
            n884 = One Button Dialog(message=w1582) -> ()  [unwired: 1 in, 1 out]
            n885 = case shown="No Error" w1580 {
              frame No Error {
                w1590 = "" ("txtID")
                n886 = local write "txtID"(w1590) -> ()
                n887 = local write "txtName"(w1590) -> ()
                n888 = local write "txtPassword"(w1590) -> ()
              }
              frame Error {
              }
            }
          }
          frame True {
            n889 = case shown="\"English\"" w1592 {
              tunnel: ["输入用户信息不全" "User's information isn't enough"] -> w1591
              frame "中文" {
              }
              frame "English" {
              }
            }
            n890 = One Button Dialog(message=w1591) -> ()  [unwired: 1 in, 1 out]
          }
        }
      }
      frame "Edit User" {
        n891 = local read "txtPassword"() -> (w1599:string)
        n892 = local read "Authority"() -> (w1598:T15)
        n893 = local read "txtName"() -> (w1600:string)
        n894 = Unbundle By Name(w1607) -> ("parameter.MLFB"=w1606:T9)
        n895 = local read "txtID"() -> (w1601:string)
        n896 = Bundle(cluster=T20 {"ID_Number"="", "Name"="", "Password"="", "Authority"=0} ("UserRight"), "ID_Number"=w1601, "Name"=w1600, "Password"=w1599, "Authority"=w1598) -> (w1604:T20)
        n897 = call "Database_User_Edit.vi"("error in"=w1603, "UserRight"=w1604, "connection reference"=w1606) -> ("error out"=w1596:errorcluster, "Message"=w1602:string)  [unwired: 2 in, 1 out]
        n898 = One Button Dialog(message=w1602) -> ()  [unwired: 1 in, 1 out]
        n899 = case shown="No Error" w1596 {
          frame No Error {
            w1611 = "" ("txtID")
            n900 = local write "txtID"(w1611) -> ()
            n901 = local write "txtName"(w1611) -> ()
            n902 = local write "txtPassword"(w1611) -> ()
            n903 = local write "Authority"(Autority."Operator" ("Authority")) -> ()
            n904 = property on="txtID" class="Str"("DisabledEnum"=T18."Enabled" ("Disabled")) -> ()  [unwired: 2 in, 2 out]
          }
          frame Error {
          }
        }
      }
      frame "Delete User" {
        n905 = Unbundle By Name(w1623) -> ("parameter.MLFB"=w1620:T9)
        n906 = local read "txtID"() -> (w1617:string)
        n907 = call "Database_User_Query.vi"("error in (no error)"=w1624, "Column"=w1617, "Table"="Operators", "connection reference"=w1620) -> ("error out"=w1621:errorcluster, "size(s)"=w1619:i32, "connection reference 2"=w1618:T9)
        n908 = Not Equal To 0?(x=w1619) -> (x != 0?=w1616:bool)
        n909 = case shown="True" w1616 {
          tunnel: [w1630 w1638] -> w1613
          tunnel: w1621 -> [w1630 w1637]
          tunnel: w1618 -> [_ w1636]
          tunnel: w1617 -> [_ w1635]
          tunnel: [w1629 w1634] -> w1615
          tunnel: w1612 -> [w1628 w1633]
          frame False {
            n910 = case shown="\"English\"" w1628 {
              tunnel: ["ID 无效" "Invalid ID Number"] -> w1629
              frame "中文" {
              }
              frame "English" {
              }
            }
          }
          frame True {
            n911 = call "Database_User_Delete.vi"("error in"=w1637, "Language"=w1633, "ID_Number"=w1635, "connection reference"=w1636) -> ("error out"=w1638:errorcluster, "Message"=w1634:string)  [unwired: 1 in, 1 out]
          }
        }
        n912 = One Button Dialog(message=w1615) -> ()  [unwired: 1 in, 1 out]
        n913 = case shown="No Error" w1613 {
          frame No Error {
            w1627 = "" ("txtID")
            n914 = local write "txtID"(w1627) -> ()
            n915 = local write "txtName"(w1627) -> ()
            n916 = local write "txtPassword"(w1627) -> ()
            n917 = property on="txtID" class="Str"("DisabledEnum"=T18."Enabled" ("Disabled")) -> ()  [unwired: 2 in, 2 out]
          }
          frame Error {
          }
        }
      }
      frame "Read User" {
        n918 = property on="txtPassword" class="Str"(error in=w1642, "Display Style"=u32 2) -> (error out=w1641:errorcluster)  [unwired: 1 in, 1 out]
        n919 = Unbundle By Name(w1654) -> ("parameter.MLFB"=w1653:T9)
        n920 = local read "txtID"() -> (w1652:string)
        n921 = call "Database_User_Read.vi"("error in"=w1641, "Language"=w1644, "ID_Number"=w1652, "connection reference"=w1653) -> ("error out"=w1640:errorcluster, "Message"=w1639:string, "UserRight"=w1651:T20)  [unwired: 4 in, 1 out]
        n922 = Unbundle(w1651) -> ("ID_Number"=w1650:string, "Name"=w1649:string, "Password"=w1647:string, "Authority"=w1648:i32)
        n923 = case shown="\"Read Successful\", \"读取成功\"" w1639 {
          tunnel: [T18."Enabled" ("Disabled") T18."Disabled and Grayed Out" ("Disabled")] -> w1646
          frame "False", Default {
          }
          frame "Read Successful", "读取成功" {
          }
        }
        n924 = One Button Dialog(message=w1639) -> ()  [unwired: 1 in, 1 out]
        n925 = local write "txtID"(w1650) -> ()
        n926 = local write "txtName"(w1649) -> ()
        n927 = local write "txtPassword"(w1647) -> ()
        n928 = local write "Authority"(w1648) -> ()
        n929 = property on="txtID" class="Str"("DisabledEnum"=w1646) -> ()  [unwired: 2 in, 2 out]
      }
      frame "Voltage" {
        n930 = Unbundle By Name(w1660) -> ("parameter.recordVoltageTime"=w1659:i32)
        n931 = To Double Precision Float(number=w1659) -> (double precision float=w1658:dbl)
        n932 = call "Elapsed Time2"("Time Target (s)"=w1658, "Reset"="Voltage Reset") -> ("Time has Elapsed"=w1662:bool)  [unwired: 10 in, 7 out]
        n933 = case shown="True" w1662 {
          tunnel: w1663 -> [_ w1668]
          frame False {
          }
          frame True {
            n934 = flat-sequence {
              tunnel: w1668 -> [w1671]
              tunnel: [w1671] -> w1669
              tunnel: w1669 -> [w1672]
              frame #0 {
                n935 = local write "Keithly"(Keithly_Action."Get Voltage" ("Keithly")) -> ()
              }
              frame #1 {
                n936 = Set Occurrence(w1672) -> ()
              }
            }
            n937 = local write "Voltage Reset"(TRUE ("Voltage Reset")) -> ()
          }
        }
      }
      frame "Time" {
        n938 = local read "LightCurtain"() -> (w1673:bool)
        n939 = Unbundle By Name(w1678) -> ("Start"=w1676:bool, "Clear"=w1675:bool)
        n940 = Compound Arithmetic op=OR(w1676, w1673) -> (w1677:bool)
        n941 = call "CustomTimer.vi"("error in (no error)"=w1682, "Clear"=w1675, "Start"=w1677) -> ("error out"=w1681:errorcluster, "elapsedSecond"=w1680:i32)  [unwired: 1 in, 2 out]
        n942 = Bundle By Name(cluster=w1678, "Elapse"=w1680, "Clear"=TRUE) -> (w1679:T3)
      }
      frame "Current Calibration" {
      }
      frame "ErrorHandle" {
        w1692 = T10."Login" ("Tab")
        w1700 = T16[] [enum."Procedure"] items=["Initial_Data", "Initial_HMI", "Language", "UI", "Login", "Authority", "Clear", "Initial Test Data", "Initial Test Data1", "Initial Test UI", "Test Parameter", "PowerRemote", "PowerON", "PowerCalibration", "PowerOFF", "Temperature", "TempOffset", "Trip", "ShowInfo", "Finish?", "Period?", "LoopCurrent", "Procedure", "KGR", "Passed", "Failed", "MLFB Decoding", "MLFB Test Info", "MLFB Edit Info", "MLFB Edit", "MLFB Insert", "MLFB Delete", "ReportGeneralInfo", "ReportResultInfo", "ReportPath", "Generate Report", "Print Report", "New User", "Edit User", "Delete User", "Read User", "Voltage", "Time", "Current Calibration", "ErrorHandle", "StartTest", "ActiveLightCur", "Uninstall Record", "Get Uninstall Count", "Abort Test", "Test Model?", "CheckLoopCurrent", "Release HW Source", "Exit", "Close DB Connection", "Test UI BTN Status", "unTest UI BTN Status", "Disable All BTN", "AbortCalibration", "TprCalibration", "ClearReportInfo", "Set Uninstall", "TestResult", "SetLightCur", "CheckVoltage", "ShowTripTime"]
        n943 = Unbundle By Name(w1695) -> ("parameter.Authority"=w1694:u32)
        n944 = Equal?(x=w1692, y=w1693) -> (x = y?=w1689:bool)
        n945 = case shown="0, Default" w1694 {
          frame 1 {
            w1703 = T18."Enabled" ("Disabled")
            # "engineer"
            n946 = property on="Start" class="Bool"("DisabledEnum"=w1703) -> ()  [unwired: 2 in, 2 out]
            n947 = property on="New" class="Bool"("DisabledEnum"=w1703) -> ()  [unwired: 2 in, 2 out]
            n948 = property on="btnAbort" class="Bool (strict)"("DisabledEnum"=T18."Disabled and Grayed Out" ("Disabled")) -> ()  [unwired: 2 in, 2 out]
            n949 = property on="Edit" class="Bool"("DisabledEnum"=w1703) -> ()  [unwired: 2 in, 2 out]
            n950 = property on="Set" class="Bool"("DisabledEnum"=w1703) -> ()  [unwired: 2 in, 2 out]
            n951 = property on="exit" class="Bool"("DisabledEnum"=w1703) -> ()  [unwired: 2 in, 2 out]
          }
          frame 0, Default {
            w1705 = T18."Enabled" ("Disabled")
            # "worker"
            n952 = property on="btnAbort" class="Bool (strict)"("DisabledEnum"=T18."Disabled and Grayed Out" ("Disabled")) -> ()  [unwired: 2 in, 2 out]
            n953 = property on="Start" class="Bool"("DisabledEnum"=w1705) -> ()  [unwired: 2 in, 2 out]
            n954 = property on="exit" class="Bool"("DisabledEnum"=w1705) -> ()  [unwired: 2 in, 2 out]
          }
        }
        n955 = Select(t=w1692, s=w1689, f=T10."Test" ("Tab")) -> (s? t:f=w1690:T10)
        n956 = local read "RunInfo"() -> (w1696:string)
        n957 = Unbundle By Name(w1702) -> ("source"=w1697:string)
        n958 = Concatenate Strings(w1696, w1697, "\r") -> (w1699:string)
        n959 = local write "RunInfo"(w1699) -> ()
      }
      frame "StartTest" {
        n960 = local read "Run?"() -> (w1711:bool)
        n961 = case shown="True" w1711 {
          tunnel: w1710 -> [w1716 _]
          tunnel: [w1717 w1720] -> w1707
          tunnel: w1709 -> [w1714 _]
          tunnel: [w1714 T10."Test" ("Tab")] -> w1708
          frame False {
            w1717 = T16[] [enum."unTest UI BTN Status", enum."Procedure"] items=["Initial_Data", "Initial_HMI", "Language", "UI", "Login", "Authority", "Clear", "Initial Test Data", "Initial Test Data1", "Initial Test UI", "Test Parameter", "PowerRemote", "PowerON", "PowerCalibration", "PowerOFF", "Temperature", "TempOffset", "Trip", "ShowInfo", "Finish?", "Period?", "LoopCurrent", "Procedure", "KGR", "Passed", "Failed", "MLFB Decoding", "MLFB Test Info", "MLFB Edit Info", "MLFB Edit", "MLFB Insert", "MLFB Delete", "ReportGeneralInfo", "ReportResultInfo", "ReportPath", "Generate Report", "Print Report", "New User", "Edit User", "Delete User", "Read User", "Voltage", "Time", "Current Calibration", "ErrorHandle", "StartTest", "ActiveLightCur", "Uninstall Record", "Get Uninstall Count", "Abort Test", "Test Model?", "CheckLoopCurrent", "Release HW Source", "Exit", "Close DB Connection", "Test UI BTN Status", "unTest UI BTN Status", "Disable All BTN", "AbortCalibration", "TprCalibration", "ClearReportInfo", "Set Uninstall", "TestResult", "SetLightCur", "CheckVoltage", "ShowTripTime"]
            n962 = case shown="\"中文\", Default" w1716 {
              tunnel: ["请按下开始按钮" "Please Press Start Button"] -> w1715
              frame "中文", Default {
              }
              frame "English" {
              }
            }
            n963 = One Button Dialog(message=w1715) -> ()  [unwired: 1 in, 1 out]
          }
          frame True {
            w1720 = T16[] [enum."Disable All BTN", enum."Initial Test Data", enum."Initial Test Data1", enum."Initial Test UI", enum."Set Uninstall", enum."Test Parameter", enum."Temperature", enum."TempOffset", enum."PowerRemote", enum."PowerON", enum."Test UI BTN Status", enum."Time", enum."Trip", enum."ShowInfo", enum."Finish?", enum."Period?"] items=["Initial_Data", "Initial_HMI", "Language", "UI", "Login", "Authority", "Clear", "Initial Test Data", "Initial Test Data1", "Initial Test UI", "Test Parameter", "PowerRemote", "PowerON", "PowerCalibration", "PowerOFF", "Temperature", "TempOffset", "Trip", "ShowInfo", "Finish?", "Period?", "LoopCurrent", "Procedure", "KGR", "Passed", "Failed", "MLFB Decoding", "MLFB Test Info", "MLFB Edit Info", "MLFB Edit", "MLFB Insert", "MLFB Delete", "ReportGeneralInfo", "ReportResultInfo", "ReportPath", "Generate Report", "Print Report", "New User", "Edit User", "Delete User", "Read User", "Voltage", "Time", "Current Calibration", "ErrorHandle", "StartTest", "ActiveLightCur", "Uninstall Record", "Get Uninstall Count", "Abort Test", "Test Model?", "CheckLoopCurrent", "Release HW Source", "Exit", "Close DB Connection", "Test UI BTN Status", "unTest UI BTN Status", "Disable All BTN", "AbortCalibration", "TprCalibration", "ClearReportInfo", "Set Uninstall", "TestResult", "SetLightCur", "CheckVoltage", "ShowTripTime"]
          }
        }
      }
      frame "ActiveLightCur" {
        n964 = Unbundle By Name(w1729) -> ("parameter.buffer.PowerSwitch"=w1726:bool[], "parameter.pwrSwitch"=w1724:refnum<k21>)
        n965 = local read "LightCurtain"() -> (w1722:bool)
        n966 = Select(t=bool[] [FALSE, FALSE], s=w1722, f=w1726) -> (s? t:f=w1725:bool[])
        n967 = call "DigitalWrite_MultiTask.vi"("error in"=w1728, "input"=w1725, "mutiTask"=w1724) -> ("error out"=w1727:errorcluster)  [unwired: 1 in]
      }
      frame "Uninstall Record" {
        n968 = Unbundle By Name(w1736) -> ("parameter.unIndex"=w1740:bool[], "parameter.Tripped Time"=w1739:i32[], "parameter.KGR"=w1738:dbl[])
        n969 = local read "voltage"() -> (w1737:dbl[])
        n970 = for {
          tunnel: w1740 -> [w1750] mode=indexing
          tunnel: w1739 -> [w1749] mode=indexing
          tunnel: w1738 -> [w1748] mode=indexing
          tunnel: w1737 -> [w1747] mode=indexing
          tunnel: [w1746] -> w1734 mode=indexing
          tunnel: [w1745] -> w1733 mode=indexing
          tunnel: [w1744] -> w1732 mode=indexing
          n971 = case shown="False" w1750 {
            tunnel: [-1 w1756] -> w1746
            tunnel: w1749 -> [_ w1756]
            tunnel: [-1.0 ("Numeric") w1755] -> w1745
            tunnel: w1748 -> [_ w1755]
            tunnel: [-1.0 w1754] -> w1744
            tunnel: w1747 -> [_ w1754]
            frame False {
            }
            frame True {
            }
          }
        }
        n972 = Bundle By Name(cluster=w1736, "parameter.Tripped Time"=w1734, "parameter.KGR"=w1733, "parameter.voltage"=w1732) -> (w1735:T3)
      }
      frame "Get Uninstall Count" {
        n973 = Unbundle By Name(w1767) -> ("parameter.IO.Break"=w1769:refnum<k21>)
        n974 = call "Test_GetUninstall.vi"("error in"=w1768, "Break"=w1769) -> ("error out"=w1757:errorcluster, "unIndex"=w1765:bool[], "numUninstall"=w1759:i32)  [unwired: 1 in]
        n975 = local read "TestModel"() -> (w1760:T13)
        n976 = Subtract(x=20, y=w1759) -> (x-y=w1761:i32)
        n977 = case shown="\"lowLimit\", Default" w1760 {
          tunnel: [w1771 2 ("numUninstall") 2 ("numUninstall")] -> w1758
          tunnel: w1759 -> [w1771 _ _]
          frame "lowLimit", Default {
          }
          frame "lowAction2" {
          }
          frame "upAction2" {
          }
        }
        n978 = Number To Decimal String(number=w1761) -> (decimal integer string=→"testCount":string)  [unwired: 1 in]
        n979 = Bundle By Name(cluster=w1767, "parameter.uninstallNum"=w1758, "parameter.unIndex"=w1765) -> (w1766:T3)
      }
      frame "Abort Test" {
        n980 = case shown="True" "btnAbort" {
          tunnel: w1774 -> [_ w1784]
          frame False {
          }
          frame True {
            n981 = case shown="\"中文\", Default" w1784 {
              tunnel: ["确认终止测试" "Confirm to abort test"] -> w1783
              tunnel: ["确认" "Yes"] -> w1782
              tunnel: ["取消" "No"] -> w1781
              frame "中文", Default {
              }
              frame "English" {
              }
            }
            n982 = Two Button Dialog(message=w1783, 1:w1781, 2:w1782) -> (T button?=→"Abort":bool)
            n983 = local write "btnAbort"(FALSE ("btnAbort")) -> ()
          }
        }
      }
      frame "Test Model?" {
        n984 = Unbundle By Name(w1794) -> ("Test Count"=w1796:u8)
        n985 = property on="TestModel" class="RadioBtnsControl (strict)"() -> ("Controls[]"=w1795:refnum<vi>[])  [unwired: 2 in, 2 out]
        n986 = case shown="1" w1796 {
          selector: w1796 -> [_ w1815]
          tunnel: w1795 -> [w1801 w1816]
          tunnel: [u8 0 ("Test Count") w1815] -> w1792
          frame 1 {
            n987 = local read "TestModel"() -> (w1802:T13)
            n988 = for {
              tunnel: w1801 -> [w1807] mode=indexing
              tunnel: w1802 -> [w1806]
              i -> [w1808]
              n989 = case shown="\"upAction2\"" w1806 {
                tunnel: [1 0 3 2 5 4] -> w1805
                frame "lowLimit" {
                }
                frame "upLimit" {
                }
                frame "lowAction1" {
                }
                frame "upAction1" {
                }
                frame "lowAction2" {
                }
                frame "upAction2" {
                }
              }
              n990 = Equal?(x=w1805, y=w1808) -> (x = y?=w1804:bool)
              n991 = To Variant(anything=w1804) -> (Variant=w1803:variant)
              n992 = property class="Ctl"(reference=w1807, "Value"=w1803) -> ()  [unwired: 1 in, 2 out]
            }
          }
          frame 0, Default {
            n993 = for {
              tunnel: w1816 -> [w1820] mode=indexing
              i -> [w1817]
              n994 = Equal To 0?(x=w1817) -> (x = 0?=w1819:bool)
              n995 = To Variant(anything=w1819) -> (Variant=w1818:variant)
              n996 = property class="Ctl"(reference=w1820, "Value"=w1818) -> ()  [unwired: 1 in, 2 out]
            }
          }
        }
        n997 = Bundle By Name(cluster=w1794, "Test Count"=w1792) -> (w1793:T3)
      }
      frame "CheckLoopCurrent" {
        n998 = local read "current"() -> (w1823:dbl)
        n999 = Less Or Equal?(x=w1823, y=0.0) -> (x <= y?=w1821:bool)
        n1000 = case shown="True" w1821 {
          tunnel: w1825 -> [w1829 _]
          tunnel: [w1829 w1831] -> w1824
          frame False {
          }
          frame True {
            w1831 = T16[] [enum."Finish?"] items=["Initial_Data", "Initial_HMI", "Language", "UI", "Login", "Authority", "Clear", "Initial Test Data", "Initial Test Data1", "Initial Test UI", "Test Parameter", "PowerRemote", "PowerON", "PowerCalibration", "PowerOFF", "Temperature", "TempOffset", "Trip", "ShowInfo", "Finish?", "Period?", "LoopCurrent", "Procedure", "KGR", "Passed", "Failed", "MLFB Decoding", "MLFB Test Info", "MLFB Edit Info", "MLFB Edit", "MLFB Insert", "MLFB Delete", "ReportGeneralInfo", "ReportResultInfo", "ReportPath", "Generate Report", "Print Report", "New User", "Edit User", "Delete User", "Read User", "Voltage", "Time", "Current Calibration", "ErrorHandle", "StartTest", "ActiveLightCur", "Uninstall Record", "Get Uninstall Count", "Abort Test", "Test Model?", "CheckLoopCurrent", "Release HW Source", "Exit", "Close DB Connection", "Test UI BTN Status", "unTest UI BTN Status", "Disable All BTN", "AbortCalibration", "TprCalibration", "ClearReportInfo", "Set Uninstall", "TestResult", "SetLightCur", "CheckVoltage", "ShowTripTime"]
            "No Current" <- TRUE ("No Current")
          }
        }
      }
      frame "Release HW Source" {
        n1001 = Unbundle By Name(w1836) -> ("parameter.IO.Contactor"=w1833:refnum<k21>)
        n1002 = call "DigitalWrite_MultiTask.vi"("error in"=w1835, "input"=bool[] [FALSE, FALSE, FALSE, FALSE, FALSE, FALSE, FALSE, FALSE, FALSE, FALSE, FALSE, FALSE, FALSE, FALSE, FALSE, FALSE, FALSE, FALSE, FALSE, FALSE] ("data"), "mutiTask"=w1833) -> ("error out"=w1834:errorcluster)  [unwired: 1 in]
      }
      frame "Exit" {
        n1003 = control-ref of="This Application"() -> (w1843:refnum<vi>)
        n1004 = property class="App"(reference=w1843) -> ("App.Kind"=w1842:T21)  [unwired: 1 in, 2 out]
        n1005 = Equal?(x=w1842, y=T21."Run Time System" ("Application:Kind")) -> (x = y?=w1840:bool)
        n1006 = case shown="True" w1840 {
          tunnel: TRUE ("stop? (T)") -> [w1848 w1849]
          frame True {
            n1007 = Quit LabVIEW(quit? (T)=w1848) -> ()
          }
          frame False {
            n1008 = Stop(stop? (T)=w1849) -> ()
          }
        }
      }
      frame "Close DB Connection" {
        n1009 = Unbundle By Name(w1851) -> ("parameter.MLFB"=w1850:T9)
        n1010 = call "Database_CloseConnection.vi"("error in"=w1853, "connection reference"=w1850) -> ("error out"=w1852:errorcluster)  [unwired: 1 in]
      }
      frame "Test UI BTN Status" {
        w1856 = T18."Disabled and Grayed Out" ("Disabled")
        n1011 = property on="btnAbort" class="Bool (strict)"("DisabledEnum"=T18."Enabled" ("Disabled")) -> ()  [unwired: 2 in, 2 out]
        n1012 = property on="Edit" class="Bool"("DisabledEnum"=w1856) -> ()  [unwired: 2 in, 2 out]
        n1013 = property on="Set" class="Bool"("DisabledEnum"=w1856) -> ()  [unwired: 2 in, 2 out]
        n1014 = property on="ok_Para" class="Bool"("DisabledEnum"=w1856) -> ()  [unwired: 2 in, 2 out]
        n1015 = property on="Start" class="Bool"("DisabledEnum"=w1856) -> ()  [unwired: 2 in, 2 out]
        n1016 = property on="New" class="Bool"("DisabledEnum"=w1856) -> ()  [unwired: 2 in, 2 out]
        n1017 = property on="Report" class="Bool (strict)"("DisabledEnum"=w1856) -> ()  [unwired: 2 in, 2 out]
        n1018 = property on="exit" class="Bool"("DisabledEnum"=w1856) -> ()  [unwired: 2 in, 2 out]
      }
      frame "unTest UI BTN Status" {
        w1863 = T18."Enabled" ("Disabled")
        n1019 = property on="Edit" class="Bool"("DisabledEnum"=w1863) -> ()  [unwired: 2 in, 2 out]
        n1020 = property on="Set" class="Bool"("DisabledEnum"=w1863) -> ()  [unwired: 2 in, 2 out]
        n1021 = property on="exit" class="Bool"("DisabledEnum"=w1863) -> ()  [unwired: 2 in, 2 out]
        n1022 = property on="Start" class="Bool"("DisabledEnum"=w1863) -> ()  [unwired: 2 in, 2 out]
        n1023 = property on="New" class="Bool"("DisabledEnum"=w1863) -> ()  [unwired: 2 in, 2 out]
        n1024 = property on="Report" class="Bool (strict)"("DisabledEnum"=w1863) -> ()  [unwired: 2 in, 2 out]
        n1025 = property on="btnAbort" class="Bool (strict)"("DisabledEnum"=T18."Disabled and Grayed Out" ("Disabled")) -> ()  [unwired: 2 in, 2 out]
      }
      frame "Disable All BTN" {
        w1868 = T18."Disabled and Grayed Out" ("Disabled")
        n1026 = property on="Edit" class="Bool"("DisabledEnum"=w1868) -> ()  [unwired: 2 in, 2 out]
        n1027 = property on="Set" class="Bool"("DisabledEnum"=w1868) -> ()  [unwired: 2 in, 2 out]
        n1028 = property on="exit" class="Bool"("DisabledEnum"=w1868) -> ()  [unwired: 2 in, 2 out]
        n1029 = property on="btnAbort" class="Bool (strict)"("DisabledEnum"=w1868) -> ()  [unwired: 2 in, 2 out]
        n1030 = property on="Start" class="Bool"("DisabledEnum"=w1868) -> ()  [unwired: 2 in, 2 out]
        n1031 = property on="New" class="Bool"("DisabledEnum"=w1868) -> ()  [unwired: 2 in, 2 out]
        n1032 = property on="Report" class="Bool (strict)"("DisabledEnum"=w1868) -> ()  [unwired: 2 in, 2 out]
      }
      frame "AbortCalibration" {
        n1033 = call "DigitalWrite_MultiTask.vi"("error in"=w1876, "input"=bool[] [FALSE, FALSE], "mutiTask"=refnum<k21> "Power Calibration") -> ("error out"=w1873:errorcluster)  [unwired: 1 in]
      }
      frame "TprCalibration" {
        w1885 = 8 items=["Continuity", "Current AC", "Current DC", "Diode", "Frequency", "Resistance 4-wire", "Period", "Resistance 2-wire", "Temperature", "Voltage AC", "Voltage DC", "Voltage DC Ratio"] ("Measurement Function (10: Voltage DC)")
        n1034 = Unbundle By Name(w1888) -> ("parameter.Instr.34461"=w1887:refnum<visa-resource-name>, "parameter.Instr.PLC"=w1882:refnum<visa-resource-name>)
        n1035 = call-poly "PLC_OutPut.vi"("error in (no error)"=w1884, "Selection"=T17."Temperature", "Resistor"=31, "VISA resource name"=w1882) -> ("error out"=w1883:errorcluster)  [unwired: 1 in, 1 out]
        n1036 = call "Multi_Read_Single.vi"("error in"=w1883, "Measurement Function (10: Voltage DC)"=w1885, "VISA resource name"=w1887) -> ("error out"=w1889:errorcluster, "Measurement"=→"vlCalTpr":dbl)  [unwired: 7 in]
      }
      frame "ClearReportInfo" {
        w1894 = T6 {"Title"={"订单数量"="", "订单号"="", "生产代码"="", "日期"="", "开始时间"="", "结束时间"="", "测试数量"="", "预载荷时间"=0, "载荷时间"=0, "检验员"="", "MLFB"="", "电流范围"="", "起动时间"="", "快速时间范围"=""}, "uL"={"KTU"=[], "Testing temp"=[], "consTime"=0, "KG"=0.0, "Tripped Time"=[], "test?"=FALSE, "KGR"=[]}, "IL"={"KTU"=[], "Testing temp"=[], "consTime"=0, "KG"=0.0, "Tripped Time"=[], "test?"=FALSE, "KGR"=[]}, "Voltage"=[], "preLoad"=0, "Load"=0, "Total"=0, "JustCode"=[]}  # Report Info
        n1037 = Bundle By Name(cluster=w1893, "parameter.Report"=w1894) -> (w1892:T3)
      }
      frame "Set Uninstall" {
        n1038 = Unbundle By Name(w1902) -> ("parameter.IO.Contactor"=w1900:refnum<k21>, "parameter.unIndex"=w1901:bool[])
        n1039 = local read "TestModel"() -> (w1898:T13)
        n1040 = call "Test_SetUninstall.vi"("error in"=w1904, "TestModel"=w1898, "Uninstall"=w1901, "Contactor"=w1900) -> ("error out"=w1903:errorcluster)  [unwired: 1 in]
      }
      frame "TestResult" {
        n1041 = local read "TestModel"() -> (w1906:T13)
        n1042 = case shown="\"lowLimit\", Default" w1906 {
          tunnel: w1910 -> [w1915 w1937]
          tunnel: [w1914 w1938] -> w1908
          tunnel: [w1913 w1936] -> w1907
          frame "lowLimit", Default {
            n1043 = Unbundle By Name(w1915) -> ("Test Count"=w1916:u8, "Period"=w1918:u8, "parameter.trip"=w1917:bool[])
            n1044 = case shown="1, Default" w1918 {
              tunnel: w1917 -> [_ w1924]
              tunnel: [w1919 w1923] -> w1913
              tunnel: [w1920 w1921] -> w1914
              tunnel: w1916 -> [w1920 w1922]
              frame 0 {
                w1919 = T16[] [enum."Failed", enum."CheckVoltage", enum."Procedure"] items=["Initial_Data", "Initial_HMI", "Language", "UI", "Login", "Authority", "Clear", "Initial Test Data", "Initial Test Data1", "Initial Test UI", "Test Parameter", "PowerRemote", "PowerON", "PowerCalibration", "PowerOFF", "Temperature", "TempOffset", "Trip", "ShowInfo", "Finish?", "Period?", "LoopCurrent", "Procedure", "KGR", "Passed", "Failed", "MLFB Decoding", "MLFB Test Info", "MLFB Edit Info", "MLFB Edit", "MLFB Insert", "MLFB Delete", "ReportGeneralInfo", "ReportResultInfo", "ReportPath", "Generate Report", "Print Report", "New User", "Edit User", "Delete User", "Read User", "Voltage", "Time", "Current Calibration", "ErrorHandle", "StartTest", "ActiveLightCur", "Uninstall Record", "Get Uninstall Count", "Abort Test", "Test Model?", "CheckLoopCurrent", "Release HW Source", "Exit", "Close DB Connection", "Test UI BTN Status", "unTest UI BTN Status", "Disable All BTN", "AbortCalibration", "TprCalibration", "ClearReportInfo", "Set Uninstall", "TestResult", "SetLightCur", "CheckVoltage", "ShowTripTime"]
                # "Failed"
              }
              frame 1, Default {
                n1045 = Or Array Elements(Boolean array=w1924) -> (logical OR=w1926:bool)
                n1046 = Not(x=w1926) -> (.not. x?=w1925:bool)
                n1047 = case shown="True" w1925 {
                  tunnel: [w1928 w1929] -> w1923
                  tunnel: [w1927 w1930] -> w1921
                  tunnel: w1922 -> [w1927 w1931]
                  frame False {
                    w1928 = T16[] [enum."Failed", enum."CheckVoltage", enum."Procedure"] items=["Initial_Data", "Initial_HMI", "Language", "UI", "Login", "Authority", "Clear", "Initial Test Data", "Initial Test Data1", "Initial Test UI", "Test Parameter", "PowerRemote", "PowerON", "PowerCalibration", "PowerOFF", "Temperature", "TempOffset", "Trip", "ShowInfo", "Finish?", "Period?", "LoopCurrent", "Procedure", "KGR", "Passed", "Failed", "MLFB Decoding", "MLFB Test Info", "MLFB Edit Info", "MLFB Edit", "MLFB Insert", "MLFB Delete", "ReportGeneralInfo", "ReportResultInfo", "ReportPath", "Generate Report", "Print Report", "New User", "Edit User", "Delete User", "Read User", "Voltage", "Time", "Current Calibration", "ErrorHandle", "StartTest", "ActiveLightCur", "Uninstall Record", "Get Uninstall Count", "Abort Test", "Test Model?", "CheckLoopCurrent", "Release HW Source", "Exit", "Close DB Connection", "Test UI BTN Status", "unTest UI BTN Status", "Disable All BTN", "AbortCalibration", "TprCalibration", "ClearReportInfo", "Set Uninstall", "TestResult", "SetLightCur", "CheckVoltage", "ShowTripTime"]
                    # "Failed"
                  }
                  frame True {
                    w1929 = T16[] [enum."KGR", enum."Uninstall Record", enum."Passed", enum."CheckVoltage", enum."ReportGeneralInfo", enum."ReportResultInfo", enum."Procedure"] items=["Initial_Data", "Initial_HMI", "Language", "UI", "Login", "Authority", "Clear", "Initial Test Data", "Initial Test Data1", "Initial Test UI", "Test Parameter", "PowerRemote", "PowerON", "PowerCalibration", "PowerOFF", "Temperature", "TempOffset", "Trip", "ShowInfo", "Finish?", "Period?", "LoopCurrent", "Procedure", "KGR", "Passed", "Failed", "MLFB Decoding", "MLFB Test Info", "MLFB Edit Info", "MLFB Edit", "MLFB Insert", "MLFB Delete", "ReportGeneralInfo", "ReportResultInfo", "ReportPath", "Generate Report", "Print Report", "New User", "Edit User", "Delete User", "Read User", "Voltage", "Time", "Current Calibration", "ErrorHandle", "StartTest", "ActiveLightCur", "Uninstall Record", "Get Uninstall Count", "Abort Test", "Test Model?", "CheckLoopCurrent", "Release HW Source", "Exit", "Close DB Connection", "Test UI BTN Status", "unTest UI BTN Status", "Disable All BTN", "AbortCalibration", "TprCalibration", "ClearReportInfo", "Set Uninstall", "TestResult", "SetLightCur", "CheckVoltage", "ShowTripTime"]
                    # "Passed"
                    n1048 = Increment(x=w1931) -> (x+1=w1930:u8)
                  }
                }
              }
            }
          }
          frame "lowAction2", "upAction2" {
            n1049 = Unbundle By Name(w1937) -> ("Test Count"=w1935:u8, "parameter.trip"=w1932:bool[])
            n1050 = Or Array Elements(Boolean array=w1932) -> (logical OR=w1934:bool)
            n1051 = Not(x=w1934) -> (.not. x?=w1933:bool)
            n1052 = case shown="False" w1933 {
              tunnel: [w1940 w1941] -> w1936
              tunnel: [w1939 w1942] -> w1938
              tunnel: w1935 -> [w1939 w1943]
              frame False {
                w1940 = T16[] [enum."Failed", enum."CheckVoltage", enum."Procedure"] items=["Initial_Data", "Initial_HMI", "Language", "UI", "Login", "Authority", "Clear", "Initial Test Data", "Initial Test Data1", "Initial Test UI", "Test Parameter", "PowerRemote", "PowerON", "PowerCalibration", "PowerOFF", "Temperature", "TempOffset", "Trip", "ShowInfo", "Finish?", "Period?", "LoopCurrent", "Procedure", "KGR", "Passed", "Failed", "MLFB Decoding", "MLFB Test Info", "MLFB Edit Info", "MLFB Edit", "MLFB Insert", "MLFB Delete", "ReportGeneralInfo", "ReportResultInfo", "ReportPath", "Generate Report", "Print Report", "New User", "Edit User", "Delete User", "Read User", "Voltage", "Time", "Current Calibration", "ErrorHandle", "StartTest", "ActiveLightCur", "Uninstall Record", "Get Uninstall Count", "Abort Test", "Test Model?", "CheckLoopCurrent", "Release HW Source", "Exit", "Close DB Connection", "Test UI BTN Status", "unTest UI BTN Status", "Disable All BTN", "AbortCalibration", "TprCalibration", "ClearReportInfo", "Set Uninstall", "TestResult", "SetLightCur", "CheckVoltage", "ShowTripTime"]
                # "Failed"
              }
              frame True {
                w1941 = T16[] [enum."KGR", enum."Uninstall Record", enum."Passed", enum."CheckVoltage", enum."ReportGeneralInfo", enum."ReportResultInfo", enum."Procedure"] items=["Initial_Data", "Initial_HMI", "Language", "UI", "Login", "Authority", "Clear", "Initial Test Data", "Initial Test Data1", "Initial Test UI", "Test Parameter", "PowerRemote", "PowerON", "PowerCalibration", "PowerOFF", "Temperature", "TempOffset", "Trip", "ShowInfo", "Finish?", "Period?", "LoopCurrent", "Procedure", "KGR", "Passed", "Failed", "MLFB Decoding", "MLFB Test Info", "MLFB Edit Info", "MLFB Edit", "MLFB Insert", "MLFB Delete", "ReportGeneralInfo", "ReportResultInfo", "ReportPath", "Generate Report", "Print Report", "New User", "Edit User", "Delete User", "Read User", "Voltage", "Time", "Current Calibration", "ErrorHandle", "StartTest", "ActiveLightCur", "Uninstall Record", "Get Uninstall Count", "Abort Test", "Test Model?", "CheckLoopCurrent", "Release HW Source", "Exit", "Close DB Connection", "Test UI BTN Status", "unTest UI BTN Status", "Disable All BTN", "AbortCalibration", "TprCalibration", "ClearReportInfo", "Set Uninstall", "TestResult", "SetLightCur", "CheckVoltage", "ShowTripTime"]
                # "Passed"
                n1053 = Increment(x=w1943) -> (x+1=w1942:u8)
              }
            }
          }
        }
        n1054 = Bundle By Name(cluster=w1910, "Test Count"=w1908) -> (w1909:T3)
      }
      frame "SetLightCur" {
        n1055 = Unbundle By Name(w1948) -> ("DelayInCase"=w1946:dbl, "DelayByUser"=w1947:dbl)
        n1056 = case shown="False" "DisableCurtain" {
          selector: "DisableCurtain" -> [_ w1972]
          tunnel: w1944 -> [w1955 _]
          tunnel: w1947 -> [_ w1973]
          tunnel: w1946 -> [w1953 _]
          frame False {
            n1057 = local read "IOLightCurtain"() -> (w1954:bool)
            n1058 = case shown="True" w1954 {
              tunnel: w1955 -> [_ w1963]
              tunnel: w1953 -> [_ w1959]
              tunnel: [FALSE ("LightCurtain") TRUE ("LightCurtain")] -> w1952
              frame False {
                n1059 = local write "LCOneT"(TRUE ("LCOneT")) -> ()
              }
              frame True {
                n1060 = case shown="True" "LCOneT" {
                  tunnel: w1963 -> [_ w1968]
                  frame False {
                  }
                  frame True {
                    n1061 = case shown="\"English\"" w1968 {
                      tunnel: ["光幕触发" "Light Curtain Actived"] -> w1966
                      frame "中文", Default {
                      }
                      frame "English" {
                      }
                    }
                    n1062 = local read "RunInfo"() -> (w1969:string)
                    n1063 = Concatenate Strings(w1969, w1966, "\r") -> (w1967:string)
                    n1064 = local write "LCOneT"(FALSE ("LCOneT")) -> ()
                    n1065 = local write "RunInfo"(w1967) -> ()
                  }
                }
                n1066 = call "ActivedInCase"("Time Target (s)"=w1959, "Reset"=FALSE) -> ("Time has Elapsed"=w1961:bool)  [unwired: 10 in, 7 out]
                n1067 = local write "Abort"(w1961) -> ()
              }
            }
            "LightCurtain" <- w1952
          }
          frame True {
            n1068 = Not(x=w1972) -> (.not. x?=w1976:bool)
            n1069 = call "Elapsed Time3"("Time Target (s)"=w1973, "Reset"=w1976) -> ("Time has Elapsed"=w1975:bool)  [unwired: 10 in, 7 out]
            n1070 = Not(x=w1975) -> (.not. x?=w1974:bool)
            n1071 = local write "DisableCurtain"(w1974) -> ()
          }
        }
      }
      frame "CheckVoltage" {
        n1072 = Unbundle By Name(w1980) -> ("CheckVoltage"=w1981:bool, "parameter.voltage"=w1979:dbl[])
        n1073 = case shown="True" w1981 {
          tunnel: w1979 -> [_ w1986]
          tunnel: w1978 -> [w1984 w1993]
          tunnel: [w1984 w1985] -> w1977
          frame False {
          }
          frame True {
            n1074 = call "ReadConfig.vi"("error in"=w1993, "section"="Voltage") -> ("error out"=w1985:errorcluster, "value"=w1992:string[])  [unwired: 3 in, 1 out]
            n1075 = Index Array(array=w1992, index #1=2 ("index")) -> (element #1=w1990:string, element #2=w1989:string)  [unwired: 1 in]
            n1076 = property on="trippedStatus" class="Clust (strict)"() -> ("AllObjs[]"=w1995:refnum<vi>[])  [unwired: 2 in, 2 out]
            n1077 = Fract/Exp String To Number(string=w1990) -> (number=w1988:dbl)  [unwired: 3 in, 1 out]
            n1078 = Fract/Exp String To Number(string=w1989) -> (number=w1987:dbl)  [unwired: 3 in, 1 out]
            n1079 = for {
              tunnel: w1995 -> [w2000] mode=indexing
              tunnel: w1988 -> [w1998]
              tunnel: w1987 -> [w1997]
              tunnel: w1986 -> [w1996] mode=indexing
              n1080 = In Range and Coerce(upper limit=w1998, x=w1996, lower limit=w1997) -> (In Range?=w1999:bool)  [unwired: 1 out]
              n1081 = case shown="False" w1999 {
                tunnel: w2000 -> [w2002 _]
                frame False {
                  w2004 = refnum<vi> refnum  # Boolean
                  n1082 = To More Specific Class(target class=w2004, reference=w2002) -> (specific class reference=w2003:refnum<vi>)  [unwired: 1 in, 1 out]
                  n1083 = property class="Bool"(reference=w2003, "Colors [4]"=cluster{u32, u32}[] [{16776960, 16776960}, {16776960, 16776960}, {13816530, 16744703}, {3381759, 16777088}] ("Array")) -> ()  [unwired: 1 in, 2 out]
                }
                frame True {
                }
              }
            }
          }
        }
      }
      frame "ShowTripTime" {
        n1084 = Unbundle By Name(w2012) -> ("parameter.Tripped Time"=w2011:i32[], "parameter.Report.preLoad"=w2010:i32, "parameter.Report.Load"=w2009:i32, "parameter.trip"=w2007:bool[])
        n1085 = property on="ShowTripTime" class="Clust (strict)"() -> ("Controls[]"=w2008:refnum<vi>[])  [unwired: 2 in, 2 out]
        n1086 = for {
          tunnel: w2011 -> [w2020] mode=indexing
          tunnel: w2010 -> [w2019]
          tunnel: w2009 -> [w2018]
          tunnel: w2008 -> [w2017] mode=indexing
          tunnel: w2007 -> [w2021] mode=indexing
          tunnel: [w2016] -> w2006 mode=indexing
          n1087 = case shown="False" w2021 {
            tunnel: w2020 -> [w2027 _]
            tunnel: w2019 -> [w2026 _]
            tunnel: w2018 -> [w2025 _]
            tunnel: w2017 -> [w2023 _]
            tunnel: [w2024 0 ("PeriodTime")] -> w2016
            frame False {
              n1088 = call "ShowPeriodByTripTime.vi"("Load"=w2025, "Preload"=w2026, "Trip"=w2027) -> ("Period"=w2022:string, "PeriodTime"=w2024:i32)
              n1089 = property class="Ctl"(reference=w2023, "Caption.Text"=w2022) -> ()  [unwired: 1 in, 2 out]
            }
            frame True {
            }
          }
        }
        n1090 = Array To Cluster(array=w2006) -> (cluster=→"ShowTripTime":T23)
      }
    }
    "Tab" <- w70
  }
  n1091 = disable-structure shown="Enabled" {
    disable-tunnel: "Output" -> [w2031 w2041]
    disable-tunnel: "Input" -> [w2030 w2042]
    disable-tunnel: errorcluster {"status"=FALSE, "code"=0, "source"=""} ("error out") -> [w2029 w2040]
    frame Disabled {
      n1092 = while {
        tunnel: w2031 -> [w2035]
        tunnel: w2030 -> [w2034]
        shift-right: [w2036] -> _
        shift-left: w2029 -> [w2037]
        stop <- w2036 stop-if-true
        n1093 = local read "Abort"() -> (w2032:bool)
        n1094 = case shown="True" w2032 {
          selector: w2032 -> [_ w2039]
          frame False {
          }
          frame True {
            n1095 = Not(x=w2039) -> (.not. x?=w2038:bool)
            n1096 = local write "Abort"(w2038) -> ()
          }
        }
        n1097 = call "IO_Control.vi"("error in"=w2037, "btnAbort"=w2032, "output"=w2035, "input"=w2034) -> ("error out"=w2036:errorcluster)  [unwired: 2 out]
        n1098 = Wait (ms)(milliseconds to wait=u32 100 ("millisecond multiple")) -> ()  [unwired: 1 out]
      }
    }
    frame Enabled {
      n1099 = while {
        tunnel: w2042 -> [w2053]
        tunnel: w2041 -> [w2052]
        shift-right: [w2049] -> _
        shift-left: _ -> [w2050]
        shift-right: [w2044] -> _
        shift-left: w2040 -> [w2051]
        stop <- w2044 stop-if-true
        n1100 = local read "Abort"() -> (w2045:bool)
        n1101 = Wait (ms)(milliseconds to wait=u32 100) -> ()  [unwired: 1 out]
        n1102 = call "IO_Control_New.vi"("btnAbort"=w2045, "error in"=w2051, "output"=w2052, "input"=w2053, "Previous"=w2050) -> ("error out"=w2044:errorcluster, "lightCurtain"=→"IOLightCurtain":bool, "On?"=→"Run?":bool, "ThisArray"=w2049:bool[])  [unwired: 3 in]
        n1103 = case shown="True" w2045 {
          selector: w2045 -> [_ w2062]
          frame False {
          }
          frame True {
            n1104 = Not(x=w2062) -> (.not. x?=w2061:bool)
            n1105 = local write "Abort"(w2061) -> ()
          }
        }
        n1106 = local read "Lang"() -> (w2043:T2)
        n1107 = case shown="Error" w2044 {
          tunnel: w2043 -> [_ w2054]
          frame No Error {
          }
          frame Error {
            n1108 = case shown="\"English\"" w2054 {
              tunnel: ["板卡异常，重启电脑" "Borad work error，rebot system"] -> w2055
              frame "中文", Default {
              }
              frame "English" {
              }
            }
            n1109 = local read "RunInfo"() -> (w2056:string)
            n1110 = Concatenate Strings(w2056, w2055, "\r") -> (w2057:string)
            n1111 = local write "RunInfo"(w2057) -> ()
          }
        }
      }
    }
  }
